vi "数据采集传输系统.vi"(8 "停止 2":bool) -> ()   [LabVIEW 2016]
uses:
  <vilib>/Averna/Notify Icon/NotifyIcon.llb/BalloonIcon.ctl
  <vilib>/Utility/miscctls.llb/LVPointTypeDef.ctl
  <vilib>/Utility/config.llb/Read Key (String).vi
  <vilib>/Utility/config.llb/Read Key (I32).vi
  <vilib>/Utility/config.llb/Read Key (Boolean).vi
  <vilib>/Utility/config.llb/Write Key (String).vi
  <vilib>/Utility/config.llb/Write Key (U32).vi
  <vilib>/Utility/config.llb/Write Key (I32).vi
  <vilib>/Utility/config.llb/Write Key (Boolean).vi
  <vilib>/Averna/Notify Icon/NotifyIcon.llb/GetSelectedItemEvent.vi
  <vilib>/Averna/Notify Icon/NotifyIcon.llb/SetVisible.vi
  <vilib>/Averna/Notify Icon/NotifyIcon.llb/SetMenuDefaultItem.vi
  <vilib>/Averna/Notify Icon/NotifyIcon.llb/SetTipText.vi
  <vilib>/Averna/Notify Icon/NotifyIcon.llb/NotifyIcon.lvclass
  <vilib>/Utility/config.llb/NI_LVConfig.lvlib
  data/FreeMem.dll
  <vilib>/ptbypt/NI_PtbyPt.lvlib
panel:
  in  "日志、参数发送":bool
  in  "2011发送":bool
  in  "判断数据反馈":bool
  in  "数据发送协议":enum16{"2005-212协议", "2017-212协议"}(ring)=enum."2017-212协议"
  in  "数据发送通道":enum16{"TCP", "VISA"}(ring)
  in  "baud rate":u32=9600 caption="波特率"
  in  "VISA resource name":refnum<visa-resource-name> caption="VISA资源名称"
  in  "查询质控数据起始时间":bool
  in  "返回主界面":bool
  out "零点核查索引起始时间":string
  out "跨度核查索引起始时间":string
  out "加标回收索引起始时间":string
  out "标样核查索引起始时间":string
  out "数据接收超时指示灯":bool
  in  "重发时间":T1(ring)
  in  "重发日期":T2(ring)
  in  "锁":bool
  in  "开机启动":bool
  in  "确定更改起始时间":bool
  in  "更改起始时间":bool
  in  "数据发送起始时间":timestamp format="%<%.3X\n%Y/%m/%d>T"
  in  "每周自动重发":bool=TRUE
  in  "确定":bool
  in  "返回":bool
  in  "PW":string
  in  "MN":string
  in  "PORT":string
  in  "IP":string
  in  "站点设备":string
  in  "站点名称":string
  out "设置超时时间/min":i32=1
  in  "实时数据发送时间间隔/min":u32=1
  out "空闲时间/s":string
  out "状态信息":T3={"1st Error to Convert "=63, "步骤 "=enum."打开连接", "元素"="实时数据", "TCP服务端掉线计数"=4, "TCP掉线时间节点"="2019/05/08 15:24:17"} {"1st Error to Convert" items=["无错误", "参数错误", "内存已满", "超出区域", "文件结束", "文件已打开", "一般文件IO错误", "未找到文件", "文件权限错误", "磁盘已满", "路径副本", "打开过多文件", "未启用", "未找到资源文件", "无法添加资源", "未找到资源", "未找到图像", "图像内存错误", "画笔不存在", "配置错误类型", "配置未找到解析段", "配置解析错误", "配置内存错误", "错误外部代码格式", "错误外部代码偏移量", "外部代码不存在", "空窗口", "销毁窗口错误", "空菜单", "打印已中止", "错误打印记录", "打印驱动程序错误", "打印时窗口错误", "打印时内存错误", "打印对话框错误", "一般打印错误", "无效设备引用句柄", "设备未找到", "设备参数错误", "设备单位错误", "无法打开设备", "设备调用已中止", "一般错误", "用户已取消", "对象ID过低", "对象ID过高", "对象不在堆中", "未知的堆", "错误DefProc ID", "DefProc不在表格中", "范围外信息", "空方法", "未知信息", "不支持管理器调用", "错误地址", "连接过程中", "连接超时", "连接过程中", "不支持网络属性", "网络错误", "正在使用的地址", "系统缺少内存", "连接已中止", "连接已拒绝", "连接未建立", "连接已建立", "连接已关闭", "初始化错误（交互应用程序管理器）", "错误事件发生", "等待无约束事件发生处理程序", "事件发生队列溢出", "错误路径", "未发出信号量", "未识别类型（交互应用程序管理器）"]}
  out "系统时间":string
  out "实时小时数据上传":bool
  out "系统状态改变":bool
  out "软件版本":string
  out "掉线指示":bool
  out "核查数据上传":bool
  out "通信状态":bool
  out "重发数据":bool
  out "配置信息":T4
  in  "参数配置":bool
  out "查询数据发送":bool
  out "读取报文显示":string
  out "发送报文显示":string
  out "心跳包":bool
  in  "参数数值":T5={"CODMn"=TRUE, "CODCr"=TRUE, "DO"=TRUE, "铜"=TRUE, "PH"=TRUE, "氨氮"=TRUE, "比电导率"=TRUE, "水温"=TRUE, "盐度(海水)"=TRUE, "浊度"=TRUE, "总氮"=TRUE, "总磷"=TRUE, "叶绿素a"=TRUE, "藻密度"=TRUE, "水位"=TRUE, "流速"=TRUE, "瞬时流量"=TRUE, "累积流量"=TRUE}
  in  "系统编码选择框":string(combo)="地表水质量监测"
  out "主队列输出":refnum<queue>
  in  "TCP掉线时间节点":string
  out "TCP服务端掉线计数":i32
  out "元素":string
  out "步骤":T6(ring)
  out "1st Error to Convert":i32(ring)=56 items=["无错误", "参数错误", "内存已满", "超出区域", "文件结束", "文件已打开", "一般文件IO错误", "未找到文件", "文件权限错误", "磁盘已满", "路径副本", "打开过多文件", "未启用", "未找到资源文件", "无法添加资源", "未找到资源", "未找到图像", "图像内存错误", "画笔不存在", "配置错误类型", "配置未找到解析段", "配置解析错误", "配置内存错误", "错误外部代码格式", "错误外部代码偏移量", "外部代码不存在", "空窗口", "销毁窗口错误", "空菜单", "打印已中止", "错误打印记录", "打印驱动程序错误", "打印时窗口错误", "打印时内存错误", "打印对话框错误", "一般打印错误", "无效设备引用句柄", "设备未找到", "设备参数错误", "设备单位错误", "无法打开设备", "设备调用已中止", "一般错误", "用户已取消", "对象ID过低", "对象ID过高", "对象不在堆中", "未知的堆", "错误DefProc ID", "DefProc不在表格中", "范围外信息", "空方法", "未知信息", "不支持管理器调用", "错误地址", "连接过程中", "连接超时", "连接过程中", "不支持网络属性", "网络错误", "正在使用的地址", "系统缺少内存", "连接已中止", "连接已拒绝", "连接未建立", "连接已建立", "连接已关闭", "初始化错误（交互应用程序管理器）", "错误事件发生", "等待无约束事件发生处理程序", "事件发生队列溢出", "错误路径", "未发出信号量", "未识别类型（交互应用程序管理器）"]
  out "QN":string
  out "时间QN":string
  out "系统编码ST":string
  out "命令编码CN":string
  out "密码PW":string
  out "设备编码MN":string
  out "拆分包及应答Flag":string
  out "数据":string
  in  "实时数据参数选择框":T7={"水样测量数据"=FALSE, "零点核查数据"=TRUE, "跨度核查数据"=TRUE, "加标回收数据"=TRUE, "平行样数据"=FALSE, "标样核查"=TRUE, "集成干预测试"=TRUE}
  out "数据输出":string
  in  "table元素":string
  out "数组":string[](array[string])
  out "数组 2":string[](array[string])
  out "空闲时间":dbl
  out "错误输出":errorcluster
  out "error out":errorcluster
  # "数 据 采 集 传 输 系 统"
  # "读取的参数区"
  # "水样测量数据"
  # "空白测试数据"
  # "跨度核查数据"
  # "加标回收数据"
  # "平行样数据"
  # "标样核查"
  # "集成干预测试"
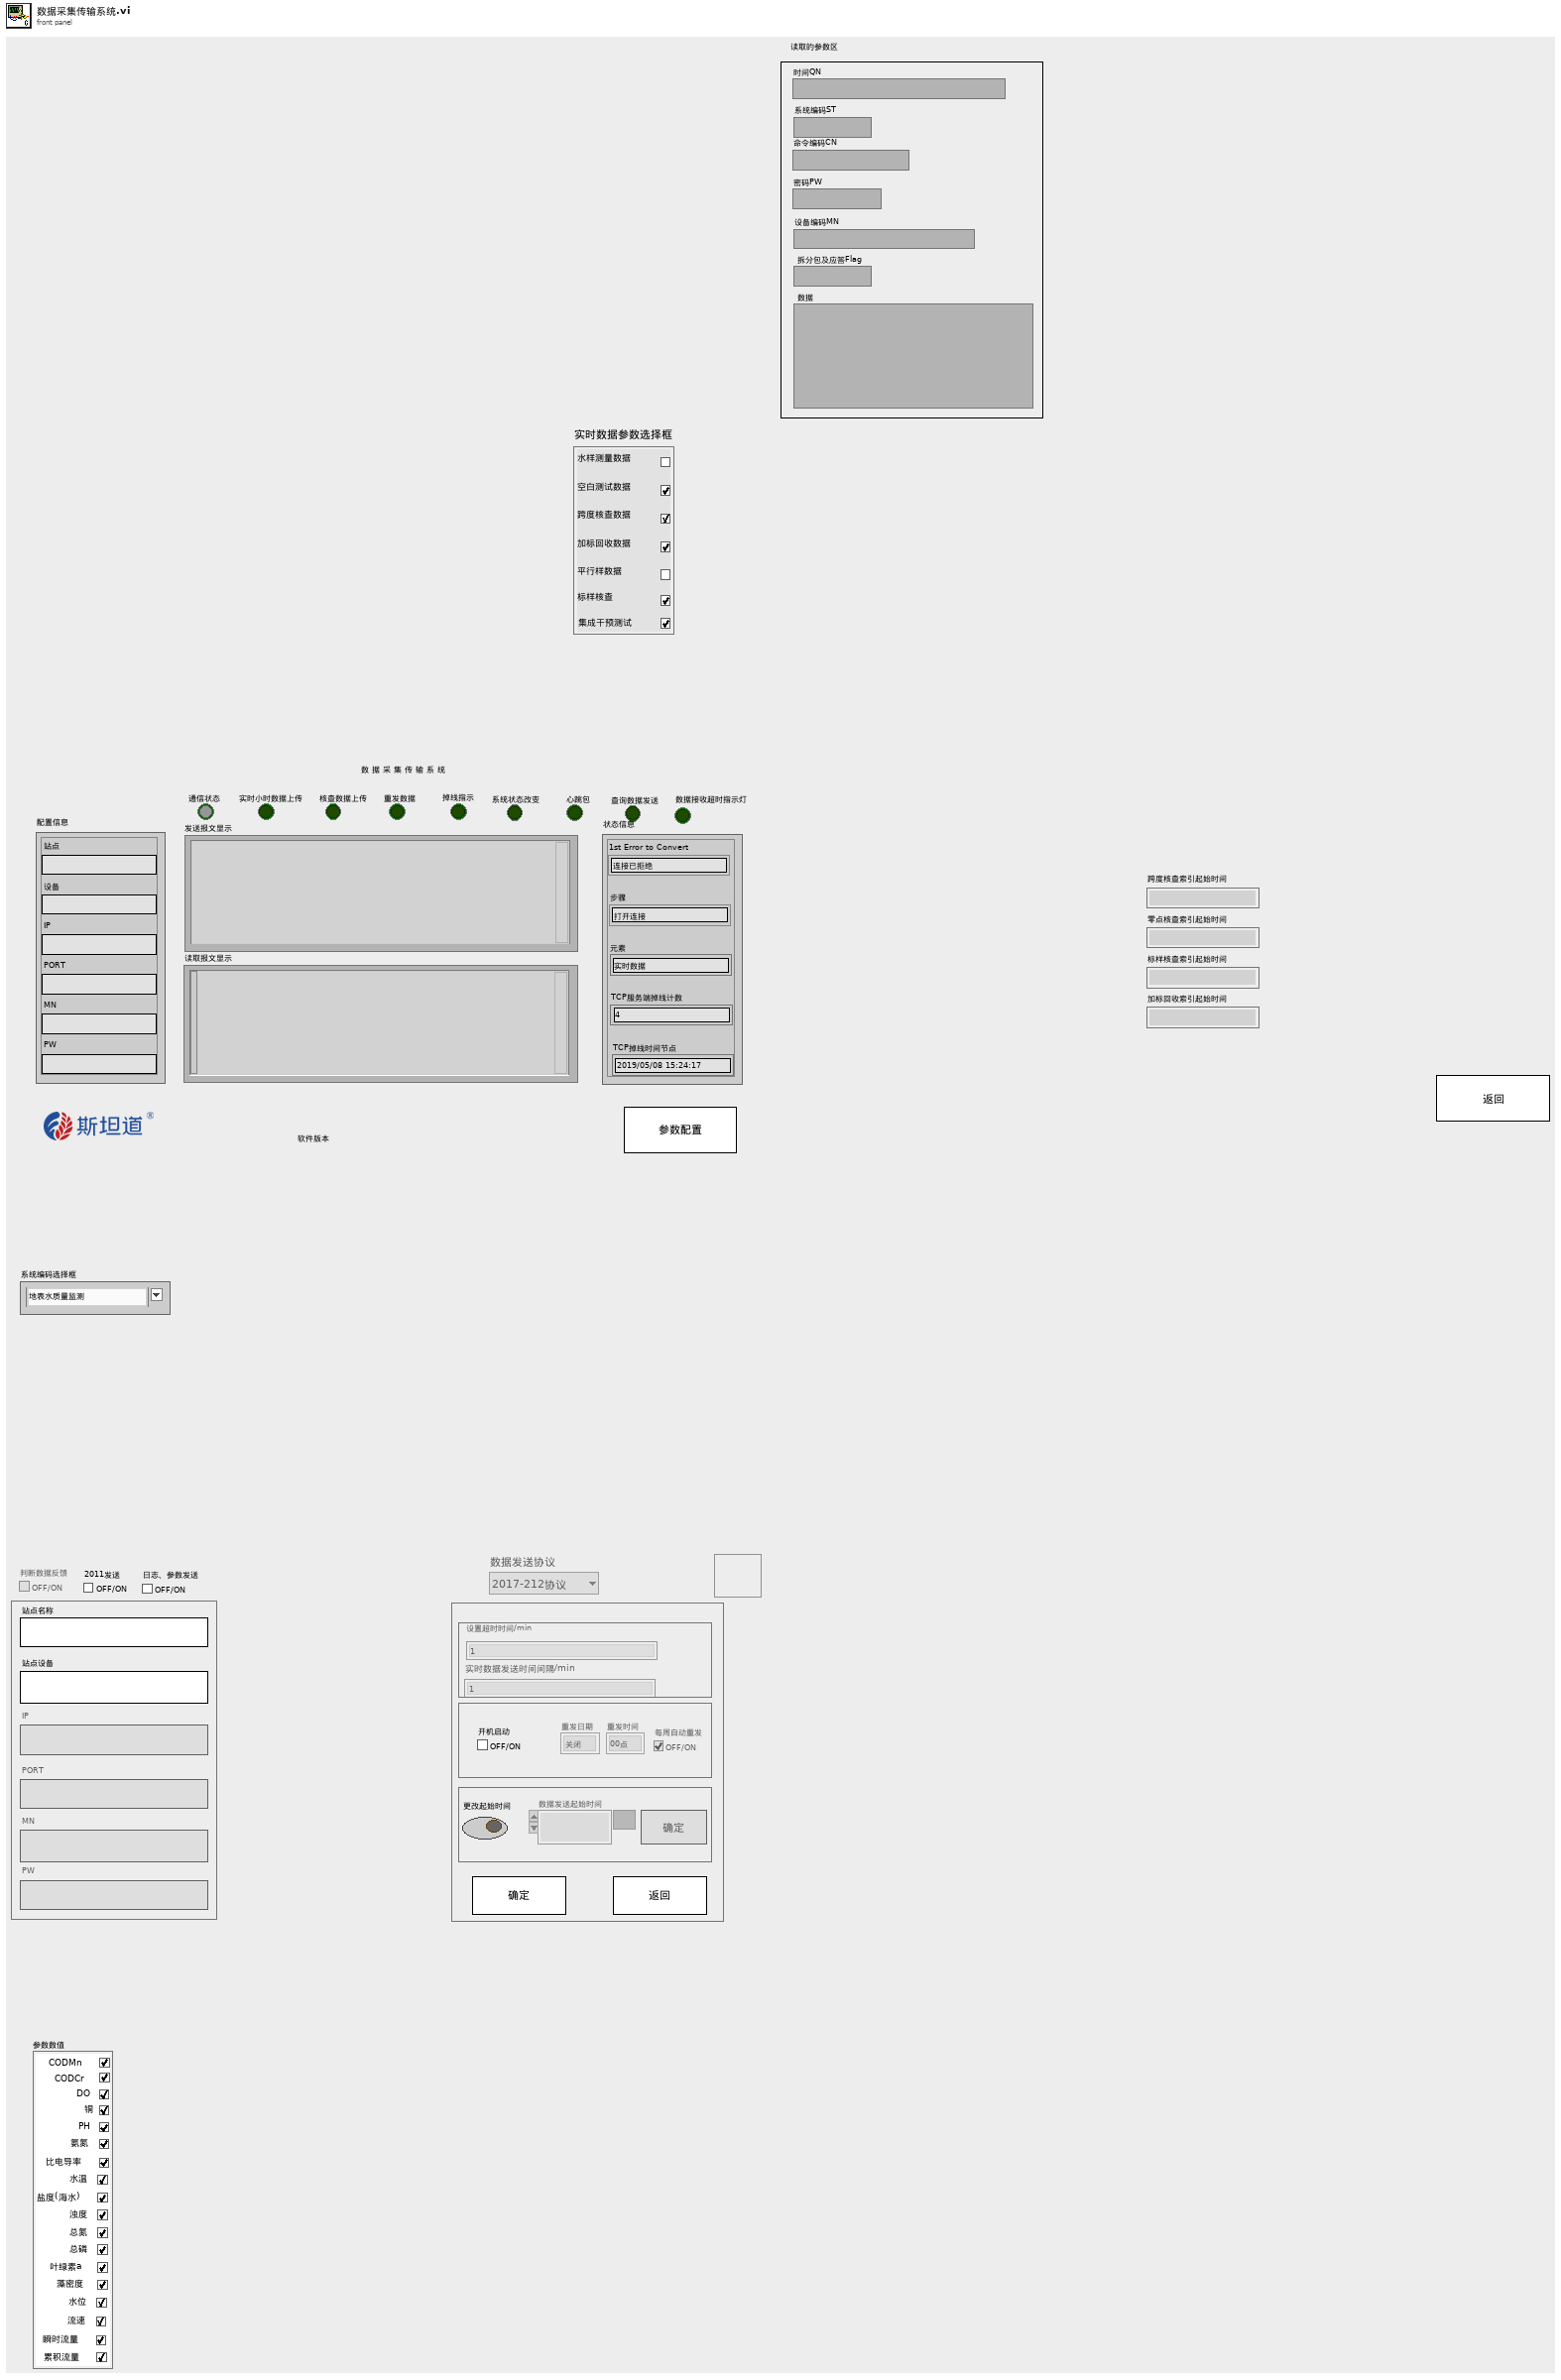
[diagram p1: front panel]
types:
  T1 = enum16{"00点", "01点", "02点", "03点", "04点", "05点", "06点", "07点", "08点", "09点", "10点", "11点", "12点", "13点", "14点", "15点", "16点", "17点", "18点", "19点", "20点", "21点", "22点", "23点"}
  T2 = enum16{"关闭", "星期日", "星期一", "星期二", "星期三", "星期四", "星期五", "星期六"}
  T3 = cluster{"1st Error to Convert ":i32, "步骤 ":enum16{"初始化", "打开连接", "表格比对", "发送数据", "读取数据", "数据处理"}, "元素":string, "TCP服务端掉线计数":i32, "TCP掉线时间节点":string}
  T4 = cluster{"站点":string, "设备":string, "IP":string, "PORT":string, "MN":string, "PW":string}
  T5 = cluster{"CODMn":bool, "CODCr":bool, "DO":bool, "铜":bool, "PH":bool, "氨氮":bool, "比电导率":bool, "水温":bool, "盐度(海水)":bool, "浊度":bool, "总氮":bool, "总磷":bool, "叶绿素a":bool, "藻密度":bool, "水位":bool, "流速":bool, "瞬时流量":bool, "累积流量":bool}
  T6 = enum16{"初始化", "打开连接", "表格比对", "发送数据", "读取数据", "数据处理"}
  T7 = cluster{"水样测量数据":bool, "零点核查数据":bool, "跨度核查数据":bool, "加标回收数据":bool, "平行样数据":bool, "标样核查":bool, "集成干预测试":bool}
  T8 = typedef "NI_LVConfig.lvlib/Config Data RefNum.ctl" = refnum<k1>
  T9 = typedef "LVDateTimeRec.ctl" = cluster{"秒数的小数部分":dbl, "秒":i32, "分":i32, "时":i32, "日":i32, "月":i32, "年":i32, "天数（周）":i32, "天数（年）":i32, "DST":i32}
  T10 = cluster{"PH":string[][], "CODCr":string[][], "氨氮":string[][], "CODMn":string[][], "总氮":string[][], "总磷":string[][], "电导率":string[][], "水温":string[][], "DO":string[][], "浊度":string[][], "叶绿素":string[][], "藻密度":string[][], "铜":string[][], "盐度":string[][], "水位":string[][], "流速":string[][], "瞬时流量":string[][], "累积流量":string[][]}
  T11 = typedef "LVPointTypeDef.ctl" = cluster{"Horizontal":i16, "Vertical":i16}
  T12 = enum8{"Enabled", "Disabled", "Disabled and Grayed Out"}
  T13 = typedef "imagedata.ctl" = cluster{"image type":i32, "image depth":i32, "image":u8[], "mask":u8[], "colors":u32[], "Rectangle":cluster{"left":i16, "top":i16, "right":i16, "bottom":i16}}
  T14 = enum32{"invalid app kind", "Development System", "Run Time System", "Student Edition", "Embedded LabVIEW", "Evaluation", "Custom"}
  T15 = enum32{"Invalid", "Standard", "Closed", "Hidden", "Minimized", "Maximized"}
  T16 = enum16{"水样测试", "小时数据", "日志信息", "报警信息", "零点核查", "标样核查", "平行样", "加标回收"}
  T17 = enum16{"CODMn", "CODCr", "氨氮", "总磷", "总氮", "数采仪"}
  T18 = cluster{"高锰酸盐":string, "化学需氧量":string, "氨氮":string, "总磷":string, "总氮":string, "数采仪":string, "高锰酸盐":bool, "化学需氧量":bool, "氨氮":bool, "总磷":bool, "总氮":bool, "数采仪":bool}
  T19 = typedef "NotifyIcon.lvlib/NotifyIcon.lvclass/BalloonIcon.ctl" = enum32{"None", "Information", "Warning", "Error"}
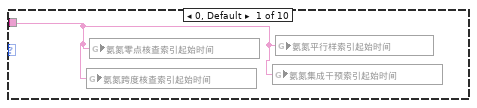
[diagram p5: hidden frame]
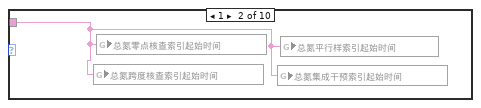
[diagram p6: hidden frame]
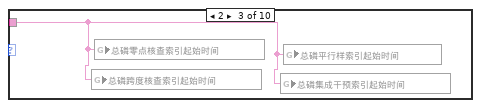
[diagram p7: hidden frame]
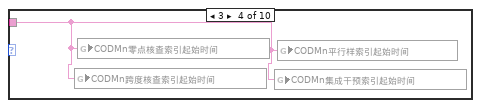
[diagram p8: hidden frame]
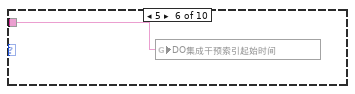
[diagram p9: hidden frame]
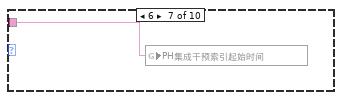
[diagram p10: hidden frame]
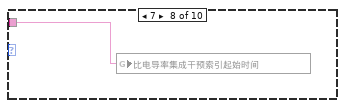
[diagram p11: hidden frame]
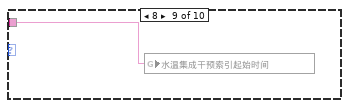
[diagram p12: hidden frame]
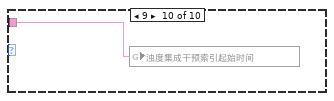
[diagram p13: hidden frame]
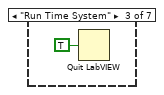
[diagram p16: hidden frame]
diagram:
  w23 = string[] ["OPEN线程一", "APP_SEPARATOR", "EXIT线程一"]
  (unwired) string[] ["CODMn", "CODCr", "DO", "DOper", "PH", "氨氮", "电导率", "水温", "盐度", "浊度", "总氮", "总磷", "叶绿素a", "藻密度", "水位", "流速", "瞬时流量", "累积流量"] ("查询参数数组")
  (unwired) 0 items=["无错误", "参数错误", "内存已满", "超出区域", "文件结束", "文件已打开", "一般文件IO错误", "未找到文件", "文件权限错误", "磁盘已满", "路径副本", "打开过多文件", "未启用", "未找到资源文件", "无法添加资源", "未找到资源", "未找到图像", "图像内存错误", "画笔不存在", "配置错误类型", "配置未找到解析段", "配置解析错误", "配置内存错误", "错误外部代码格式", "错误外部代码偏移量", "外部代码不存在", "空窗口", "销毁窗口错误", "空菜单", "打印已中止", "错误打印记录", "打印驱动程序错误", "打印时窗口错误", "打印时内存错误", "打印对话框错误", "一般打印错误", "无效设备引用句柄", "设备未找到", "设备参数错误", "设备单位错误", "无法打开设备", "设备调用已中止", "一般错误", "用户已取消", "对象ID过低", "对象ID过高", "对象不在堆中", "未知的堆", "错误DefProc ID", "DefProc不在表格中", "范围外信息", "空方法", "未知信息", "不支持管理器调用", "错误地址", "连接过程中", "连接超时", "连接过程中", "不支持网络属性", "网络错误", "正在使用的地址", "系统缺少内存", "连接已中止", "连接已拒绝", "连接未建立", "连接已建立", "连接已关闭", "初始化错误（交互应用程序管理器）", "错误事件发生", "等待无约束事件发生处理程序", "事件发生队列溢出", "错误路径", "未发出信号量", "未识别类型（交互应用程序管理器）"] ("1st Error to Convert")
  # "6."
  # "3."
  # "1."
  # "判定当数据没有传送完毕并掉线，将数据存储入临时表格"
  # "上传本地时间点的实时数据"
  # "目前时间太短，如果掉线了，数据存不了临时表格"
  # "获取需要发送的数据表"
  n1 = Cluster To Array(cluster="参数数值") -> (array=w33:bool[])
  n2 = for {
    tunnel: w33 -> [_] mode=indexing
    tunnel: [w73] -> w32
    i -> [w73]
    w62 = "线程一数据重发功能" ("section")
    # "初始化水样搜索起始时间"
    n3 = case shown="3" w73 {
      tunnel: [w104 w106 w108 w110 w112 w114 w116 w118 w120 w122 w124 w126 w128 w130 w132 w134 w136 w138] -> w77
      frame 0, Default {
        n4 = control-ref of="CODMn"() -> (w105:refnum<vi>)
        n5 = property class="Bool (严格)"(reference=w105) -> ("Label.Text"=w104:string)  [unwired: 1 in, 2 out]
      }
      frame 1 {
        n6 = control-ref of="CODCr"() -> (w107:refnum<vi>)
        n7 = property class="Bool (严格)"(reference=w107) -> ("Label.Text"=w106:string)  [unwired: 1 in, 2 out]
      }
      frame 2 {
        n8 = control-ref of="DO"() -> (w109:refnum<vi>)
        n9 = property class="Bool (严格)"(reference=w109) -> ("Label.Text"=w108:string)  [unwired: 1 in, 2 out]
      }
      frame 3 {
        n10 = control-ref of="铜"() -> (w111:refnum<vi>)
        n11 = property class="Bool (严格)"(reference=w111) -> ("Label.Text"=w110:string)  [unwired: 1 in, 2 out]
      }
      frame 4 {
        n12 = control-ref of="PH"() -> (w113:refnum<vi>)
        n13 = property class="Bool (严格)"(reference=w113) -> ("Label.Text"=w112:string)  [unwired: 1 in, 2 out]
      }
      frame 5 {
        n14 = control-ref of="氨氮"() -> (w115:refnum<vi>)
        n15 = property class="Bool (严格)"(reference=w115) -> ("Label.Text"=w114:string)  [unwired: 1 in, 2 out]
      }
      frame 6 {
        n16 = control-ref of="比电导率"() -> (w117:refnum<vi>)
        n17 = property class="Bool (严格)"(reference=w117) -> ("Label.Text"=w116:string)  [unwired: 1 in, 2 out]
      }
      frame 7 {
        n18 = control-ref of="水温"() -> (w119:refnum<vi>)
        n19 = property class="Bool (严格)"(reference=w119) -> ("Label.Text"=w118:string)  [unwired: 1 in, 2 out]
      }
      frame 8 {
        n20 = control-ref of="盐度(海水)"() -> (w121:refnum<vi>)
        n21 = property class="Bool (严格)"(reference=w121) -> ("Label.Text"=w120:string)  [unwired: 1 in, 2 out]
      }
      frame 9 {
        n22 = control-ref of="浊度"() -> (w123:refnum<vi>)
        n23 = property class="Bool (严格)"(reference=w123) -> ("Label.Text"=w122:string)  [unwired: 1 in, 2 out]
      }
      frame 10 {
        n24 = control-ref of="总氮"() -> (w125:refnum<vi>)
        n25 = property class="Bool (严格)"(reference=w125) -> ("Label.Text"=w124:string)  [unwired: 1 in, 2 out]
      }
      frame 11 {
        n26 = control-ref of="总磷"() -> (w127:refnum<vi>)
        n27 = property class="Bool (严格)"(reference=w127) -> ("Label.Text"=w126:string)  [unwired: 1 in, 2 out]
      }
      frame 12 {
        n28 = control-ref of="叶绿素a"() -> (w129:refnum<vi>)
        n29 = property class="Bool (严格)"(reference=w129) -> ("Label.Text"=w128:string)  [unwired: 1 in, 2 out]
      }
      frame 13 {
        n30 = control-ref of="藻密度"() -> (w131:refnum<vi>)
        n31 = property class="Bool (严格)"(reference=w131) -> ("Label.Text"=w130:string)  [unwired: 1 in, 2 out]
      }
      frame 14 {
        n32 = control-ref of="水位"() -> (w133:refnum<vi>)
        n33 = property class="Bool (严格)"(reference=w133) -> ("Label.Text"=w132:string)  [unwired: 1 in, 2 out]
      }
      frame 15 {
        n34 = control-ref of="流速"() -> (w135:refnum<vi>)
        n35 = property class="Bool (严格)"(reference=w135) -> ("Label.Text"=w134:string)  [unwired: 1 in, 2 out]
      }
      frame 16 {
        n36 = control-ref of="瞬时流量"() -> (w137:refnum<vi>)
        n37 = property class="Bool (严格)"(reference=w137) -> ("Label.Text"=w136:string)  [unwired: 1 in, 2 out]
      }
      frame 17 {
        n38 = control-ref of="累积流量"() -> (w139:refnum<vi>)
        n39 = property class="Bool (严格)"(reference=w139) -> ("Label.Text"=w138:string)  [unwired: 1 in, 2 out]
      }
    }
    n40 = call <vilib>:"Application Directory.vi"() -> ("Application Directory"=w83:path)
    n41 = Build Path(base path=w83, name or relative path="data\\Set.ini" ("名称或相对路径")) -> (appended path=w81:path)
    n42 = call <vilib>:"Open Config Data.vi"("configuration file path"=w81) -> ("error out"=w79:errorcluster, "refnum"=w80:T8)  [unwired: 8 in, 1 out]
    n43 = call-poly <vilib>:"Read Key.vi"("section"="线程一数据搜索起始时间", "error in (no error)"=w79, "key"=w77, "refnum"=w80) -> ("error out"=w71:errorcluster, "value"=w74:string, "refnum out"=w72:T8)  [unwired: 4 in, 1 out]
    n44 = Empty String/Path?(string/path=w74) -> (empty?=w76:bool)
    n45 = case shown="真" w76 {
      tunnel: [w84 "1904/01/01 00:00:00"] -> w75
      tunnel: w74 -> [w84 _]
      frame False {
      }
      frame True {
      }
    }
    n46 = call-poly <vilib>:"Read Key.vi"("section"=w62, "error in (no error)"=w71, "key"="重发功能", "refnum"=w72) -> ("error out"=w65:errorcluster, "value"=w69:bool, "refnum out"=w66:T8)  [unwired: 4 in, 1 out]
    n47 = local write "每周自动重发"(w69) -> ()
    n48 = call-poly <vilib>:"Read Key.vi"("section"=w62, "error in (no error)"=w65, "key"="重发日期", "refnum"=w66) -> ("error out"=w63:errorcluster, "value"=w59:i32, "refnum out"=w64:T8)  [unwired: 4 in, 1 out]
    n49 = local write "重发日期"(w59) -> ()
    n50 = case shown="3" w73 {
      tunnel: w75 -> [w86 w87 w88 w89 w90 w91 w92 w93 w94 w95 w96 w97 w98 w99 w100 w101 w102 w103]
      frame 0, Default {
        n51 = global write "全局 水样时间.vi" "time1"(w86) -> ()
      }
      frame 1 {
        n52 = global write "全局 水样时间.vi" "time2"(w87) -> ()
      }
      frame 2 {
        n53 = global write "全局 水样时间.vi" "time3"(w88) -> ()
      }
      frame 3 {
        n54 = global write "全局 水样时间.vi" "time4"(w89) -> ()
      }
      frame 4 {
        n55 = global write "全局 水样时间.vi" "time5"(w90) -> ()
      }
      frame 5 {
        n56 = global write "全局 水样时间.vi" "time6"(w91) -> ()
      }
      frame 6 {
        n57 = global write "全局 水样时间.vi" "time7"(w92) -> ()
      }
      frame 7 {
        n58 = global write "全局 水样时间.vi" "time8"(w93) -> ()
      }
      frame 8 {
        n59 = global write "全局 水样时间.vi" "time9"(w94) -> ()
      }
      frame 9 {
        n60 = global write "全局 水样时间.vi" "time10"(w95) -> ()
      }
      frame 10 {
        n61 = global write "全局 水样时间.vi" "time11"(w96) -> ()
      }
      frame 11 {
        n62 = global write "全局 水样时间.vi" "time12"(w97) -> ()
      }
      frame 12 {
        n63 = global write "全局 水样时间.vi" "time13"(w98) -> ()
      }
      frame 13 {
        n64 = global write "全局 水样时间.vi" "time14"(w99) -> ()
      }
      frame 14 {
        n65 = global write "全局 水样时间.vi" "time15"(w100) -> ()
      }
      frame 15 {
        n66 = global write "全局 水样时间.vi" "time16"(w101) -> ()
      }
      frame 16 {
        n67 = global write "全局 水样时间.vi" "time17"(w102) -> ()
      }
      frame 17 {
        n68 = global write "全局 水样时间.vi" "time18"(w103) -> ()
      }
    }
    n69 = call-poly <vilib>:"Read Key.vi"("section"=w62, "error in (no error)"=w63, "key"="重发时间", "refnum"=w64) -> ("error out"=w60:errorcluster, "value"=w58:i32, "refnum out"=w61:T8)  [unwired: 4 in, 1 out]
    n70 = local write "重发时间"(w58) -> ()
    n71 = call <vilib>:"Close Config Data.vi"("error in (no error)"=w60, "refnum"=w61) -> ()  [unwired: 8 in, 2 out]
  }
  n72 = Obtain Queue(name (unnamed)="数据发送" ("名称（未命名）"), element data type="") -> (queue out=w38:refnum<queue>, error out=w37:errorcluster)  [unwired: 3 in, 1 out]
  n73 = Obtain Queue(name (unnamed)="实时数据参数选择" ("名称（未命名）"), element data type="") -> (queue out=w39:refnum<queue>, error out=w36:errorcluster)  [unwired: 3 in, 1 out]
  n74 = while {
    tunnel: w38 -> [w155]
    stop <- FALSE stop-if-true
    # "核查和质控数据的定期发送在实时数据周期上传"
    # "指定周期发一次核查数据，仪器参数日志"
    n75 = local read "核查数据上传"() -> (w141:bool)
    n76 = local read "查询数据发送"() -> (w150:bool)
    n77 = local read "实时小时数据上传"() -> (w154:bool)
    n78 = local read "重发数据"() -> (w151:bool)
    n79 = Multiply(x="实时数据发送时间间隔/min", y=u32 60000 ("等待时间（毫秒）")) -> (x*y=w158:u32)
    n80 = local read "步骤"() -> (w149:T6)
    n81 = Not(x=w141) -> (.not. x?=w140:bool)
    n82 = Not(x=w150) -> (.not. x?=w146:bool)
    n83 = Wait (ms)(milliseconds to wait=w158) -> ()  [unwired: 1 out]
    n84 = Not(x=w151) -> (.not. x?=w145:bool)
    n85 = Not(x=w154) -> (.not. x?=w152:bool)
    n86 = First Call?() -> (First Call?: T/F=w156:bool)
    n87 = Equal?(x=w149, y=T6."读取数据" ("步骤")) -> (x = y?=w147:bool)
    n88 = case shown="真" w156 {
      tunnel: w155 -> [_ _]
      frame False {
      }
      frame True {
        (unwired) "1994/01/01 00:00:00"
        # "上传最近一年的质控数据"
        n89 = Get Date/Time In Seconds() -> (seconds since 1Jan1904=w193:timestamp)
        n90 = Seconds To Date/Time(time stamp (now)=w193) -> (date time rec=w191:T9)  [unwired: 1 in]
        n91 = Unbundle By Name(w191) -> ("年"=w192:i32)
        n92 = Decrement(x=w192) -> (x-1=w190:i32)
        n93 = Bundle By Name(cluster=w191, "年"=w190) -> (w188:T9)
        n94 = Date/Time To Seconds(2:w188) -> (0:w189:timestamp)  [unwired: 1 in]
        n95 = Format Date/Time String(time format string (%c)="%Y/%m/%d %H:%M:%S" ("时间格式字符串(%c)"), seconds (now)=w189) -> (date/time string=w186:string)  [unwired: 1 in]
        n96 = global write "全局 时间2.vi" "跨度核查索引起始时间"(w186) -> ()
        n97 = global write "全局 时间2.vi" "零点核查索引起始时间"(w186) -> ()
        n98 = global write "全局 时间2.vi" "平行样索引起始时间"(w186) -> ()
        n99 = global write "全局 时间2.vi" "加标回收索引起始时间"(w186) -> ()
        n100 = global write "全局 时间2.vi" "标样核查索引起始时间"(w186) -> ()
        n101 = call <vilib>:"Application Directory.vi"() -> ("Application Directory"=w183:path)
        n102 = Build Path(base path=w183, name or relative path="data\\hecha.ini" ("名称或相对路径")) -> (appended path=w185:path)
        n103 = call <vilib>:"Open Config Data.vi"("configuration file path"=w185) -> ("error out"=w179:errorcluster, "refnum"=w180:T8)  [unwired: 8 in, 1 out]
        n104 = vi-ref "全局 时间2.vi"() -> (w181:refnum<vi>)
        n105 = call <userlib>:"Read Panel from INI__ogtk.vi"("error in (no error)"=w179, "VI ref"=w181, "refnum"=w180) -> ("error out"=w178:errorcluster, "refnum out"=w182:T8)  [unwired: 7 in]
        n106 = call <vilib>:"Close Config Data.vi"("error in (no error)"=w178, "refnum"=w182) -> ("error out"=w177:errorcluster)  [unwired: 8 in, 1 out]
        n107 = disable-structure shown="禁用" {
          disable-tunnel: w186 -> [w196 _]
          disable-tunnel: w177 -> [w194 _]
          frame Disabled {
            n108 = for {
              N: 10 -> [_]
              tunnel: w196 -> [w197]
              tunnel: w194 -> [_]
              i -> [w198]
              n109 = case shown="4" w198 {
                tunnel: w197 -> [w199 w200 w201 w202 w203 w204 w205 w206 w207 w208]
                frame 0, Default {
                  n110 = global write "全局 时间2.vi" "氨氮跨度核查索引起始时间"(w199) -> ()
                  n111 = global write "全局 时间2.vi" "氨氮零点核查索引起始时间"(w199) -> ()
                  n112 = global write "全局 时间2.vi" "氨氮集成干预索引起始时间"(w199) -> ()
                  n113 = global write "全局 时间2.vi" "氨氮平行样索引起始时间"(w199) -> ()
                }
                frame 1 {
                  n114 = global write "全局 时间2.vi" "总氮跨度核查索引起始时间"(w200) -> ()
                  n115 = global write "全局 时间2.vi" "总氮零点核查索引起始时间"(w200) -> ()
                  n116 = global write "全局 时间2.vi" "总氮集成干预索引起始时间"(w200) -> ()
                  n117 = global write "全局 时间2.vi" "总氮平行样索引起始时间"(w200) -> ()
                }
                frame 2 {
                  n118 = global write "全局 时间2.vi" "总磷跨度核查索引起始时间"(w201) -> ()
                  n119 = global write "全局 时间2.vi" "总磷零点核查索引起始时间"(w201) -> ()
                  n120 = global write "全局 时间2.vi" "总磷集成干预索引起始时间"(w201) -> ()
                  n121 = global write "全局 时间2.vi" "总磷平行样索引起始时间"(w201) -> ()
                }
                frame 3 {
                  n122 = global write "全局 时间2.vi" "CODMn跨度核查索引起始时间"(w202) -> ()
                  n123 = global write "全局 时间2.vi" "CODMn零点核查索引起始时间"(w202) -> ()
                  n124 = global write "全局 时间2.vi" "CODMn集成干预索引起始时间"(w202) -> ()
                  n125 = global write "全局 时间2.vi" "CODMn平行样索引起始时间"(w202) -> ()
                }
                frame 4 {
                  n126 = global write "全局 时间2.vi" "CODCr跨度核查索引起始时间"(w203) -> ()
                  n127 = global write "全局 时间2.vi" "CODCr零点核查索引起始时间"(w203) -> ()
                  n128 = global write "全局 时间2.vi" "CODCr集成干预索引起始时间"(w203) -> ()
                  n129 = global write "全局 时间2.vi" "CODCr平行样索引起始时间"(w203) -> ()
                }
                frame 5 {
                  n130 = global write "全局 时间2.vi" "DO集成干预索引起始时间"(w204) -> ()
                }
                frame 6 {
                  n131 = global write "全局 时间2.vi" "PH集成干预索引起始时间"(w205) -> ()
                }
                frame 7 {
                  n132 = global write "全局 时间2.vi" "比电导率集成干预索引起始时间"(w206) -> ()
                }
                frame 8 {
                  n133 = global write "全局 时间2.vi" "水温集成干预索引起始时间"(w207) -> ()
                }
                frame 9 {
                  n134 = global write "全局 时间2.vi" "浊度集成干预索引起始时间"(w208) -> ()
                }
              }
            }
          }
          frame Enabled {
          }
        }
      }
    }
    n135 = local read "数据发送协议"() -> (w144:enum16{"2005-212协议", "2017-212协议"})
    n136 = Equal?(x=w144, y=enum16{"2005-212协议", "2017-212协议"}."2017-212协议" ("数据发送协议")) -> (x = y?=w142:bool)
    n137 = Compound Arithmetic op=AND ("复合运算")(w140, w142, w145, w146, w147, w152) -> (w153:bool)
    n138 = case shown="真" w153 {
      tunnel: w155 -> [_ w165]
      frame False {
      }
      frame True {
        n139 = call "实时数据参数入列队.vi"("实时数据参数选择框"="实时数据参数选择框") -> ("错误输出"=w167:errorcluster)  [unwired: 10 in]
        n140 = local read "日志、参数发送"() -> (w161:bool)
        n141 = call <vilib>:"Clear Errors.vi"("error in (no error)"=w167) -> ()  [unwired: 5 in, 2 out]
        n142 = Enqueue Element(queue=w165, element="send" ("元素")) -> (queue out=w164:refnum<queue>, error out=w163:errorcluster)  [unwired: 2 in, 1 out]
        n143 = case shown="真" w161 {
          tunnel: w164 -> [_ w174]
          tunnel: w163 -> [_ w173]
          frame False {
          }
          frame True {
            n144 = Enqueue Element(queue=w174, element="操作日志" ("元素"), error in (no error)=w173) -> (queue out=w171:refnum<queue>, error out=w170:errorcluster)  [unwired: 1 in, 1 out]
            n145 = Enqueue Element(queue=w171, element="仪器参数" ("元素"), error in (no error)=w170) -> (queue out=w169:refnum<queue>, error out=w168:errorcluster)  [unwired: 1 in, 1 out]
            n146 = Enqueue Element(queue=w169, element="报警信息" ("元素"), error in (no error)=w168) -> ()  [unwired: 1 in, 3 out]
          }
        }
      }
    }
  }
  n147 = while "While循环" {
    tunnel: w38 -> [w221]
    tunnel: w39 -> [w225]
    tunnel: w37 -> [w224]
    tunnel: w36 -> [w223]
    stop <- FALSE stop-if-true
    # "判定数据发送时要发送实时数据"
    # "所有的主动上传数据都是有数据才会上传"
    n148 = Get Queue Status(queue=w221) -> (# elements in queue=w213:i32)  [unwired: 2 in, 7 out]
    n149 = local read "查询数据发送"() -> (w219:bool)
    n150 = global read "全局 数据发送重叠.vi" "主动上报数据中"() -> (w211:bool)
    n151 = local read "重发数据"() -> (w210:bool)
    n152 = Not Equal To 0?(x=w213) -> (x != 0?=w220:bool)
    n153 = And(x=w220, y=w219) -> (x .and. y?=w212:bool)
    n154 = call <vilib>:"Boolean Crossing PtByPt.vi"("direction"=enum16{"either", "false-true", "true-false"}."false-true", "input"=w212) -> ("crossing"=w218:bool)  [unwired: 1 in]
    n155 = Not(x=w211) -> (.not. x?=w215:bool)
    n156 = Not(x=w210) -> (.not. x?=w209:bool)
    n157 = Not(x=w219) -> (.not. x?=w216:bool)
    n158 = case shown="真" w218 {
      frame False {
      }
      frame True {
        n159 = Get Date/Time In Seconds() -> (seconds since 1Jan1904=w231:timestamp)
        n160 = Seconds To Date/Time(time stamp (now)=w231) -> (date time rec=w228:T9)  [unwired: 1 in]
        n161 = Date/Time To Seconds(2:w228) -> (0:w230:timestamp)  [unwired: 1 in]
        n162 = Format Date/Time String(time format string (%c)="%Y/%m/%d %H:%M:%S" ("时间格式字符串(%c)"), seconds (now)=w230) -> (date/time string=w227:string)  [unwired: 1 in]
        n163 = global write "全局 数据发送重叠.vi" "数据发送重叠开始时间戳"(w227) -> ()
      }
    }
    n164 = Compound Arithmetic op=AND ("复合运算")(w216, w215, w209) -> (w214:bool)
    n165 = Wait (ms)(milliseconds to wait=u32 1000 ("等待时间（毫秒）")) -> ()  [unwired: 1 out]
    n166 = case shown="真" w214 {
      tunnel: w221 -> [_ w241]
      tunnel: w225 -> [_ w240]
      tunnel: w224 -> [_ w239]
      tunnel: w223 -> [_ w238]
      tunnel: w213 -> [_ w234]
      tunnel: w212 -> [_ w233]
      frame False {
        n167 = local write "核查数据上传"(FALSE ("数据上传")) -> ()
      }
      frame True {
        n168 = Equal To 0?(x=w234) -> (x = 0?=w235:bool)
        n169 = global write "全局 数据发送重叠.vi" "数据发送重叠"(w233) -> ()
        n170 = Not(x=w235) -> (.not. x?=w236:bool)
        n171 = local write "核查数据上传"(w236) -> ()
        n172 = Dequeue Element(queue=w241, error in (no error)=w239) -> (element=w237:string)  [unwired: 1 in, 3 out]
        n173 = case shown="\"send\"" w237 {
          tunnel: w240 -> [_ w243 _ _ _ _ _ _ _ _ _]
          tunnel: w238 -> [_ w242 _ _ _ _ _ _ _ _ _]
          frame "假", Default {
          }
          frame "send" {
            # "间隔时间上传"
            n174 = while {
              tunnel: w243 -> [w247]
              tunnel: w242 -> [w244]
              stop <- w248 stop-if-true
              n175 = Dequeue Element(queue=w247, error in (no error)=w244) -> (queue out=w246:refnum<queue>, element=w249:string)  [unwired: 1 in, 2 out]
              n176 = case shown="\"空白测试\"" w249 {
                tunnel: [_ _ _ w415 _ _ _ w622] -> w248
                tunnel: w246 -> [_ _ _ _ _ _ _ w625]
                frame "水样测试" {
                  n177 = flat-sequence {
                    frame #0 {
                      n178 = global write "全局 小时数据发送次数.vi" "小时数据发送次数"(0 ("小时数据发送次数")) -> ()
                      n179 = global write "全局 实时数据参数.vi" "实时数据参数"("水样测试") -> ()
                      n180 = global write "全局1.vi" "枚举"(enum16{"返回请求应答", "上传数据", "返回执行结果"}."上传数据" ("枚举")) -> ()
                    }
                    frame #1 {
                      n181 = call "从数据库获取数据通用可配置(子VI).vi"("table输入"="实时数据" ("新元素/子数组"), "列队名（唯一）"="a") -> ()  [unwired: 8 in, 2 out]
                    }
                    frame #2 {
                      n182 = call "实时小时数据处理整合 (子VI).vi"("枚举"=enum16{"实时数据排序", "小时数据排序"}."实时数据排序") -> ("已排序的数组"=w256:string[])  [unwired: 10 in]
                      n183 = Array Size(array=w256) -> (size(s)=w257:i32)
                      n184 = global write "全局 数据数组大小.vi" "数据数组大小"(w257) -> ()
                    }
                    frame #3 {
                      n185 = while {
                        stop <- w262 stop-if-true
                        n186 = property on="TCP服务端掉线计数" class="DigNum (严格)"() -> ("Value"=w265:i32)  [unwired: 2 in, 2 out]
                        n187 = Greater Or Equal?(x=w265, y=1) -> (x >= y?=w264:bool)
                        n188 = case shown="假" w264 {
                          frame False {
                            n189 = global read "全局 数据数组大小.vi" "数据数组大小"() -> (w267:i32)
                            n190 = Greater Than 0?(x=w267) -> (x > 0?=w268:bool)
                            n191 = case shown="真" w268 {
                              frame False {
                              }
                              frame True {
                                n192 = local read "MN"() -> (w274:string)
                                n193 = local read "PW"() -> (w273:string)
                                n194 = local read "数据发送通道"() -> (w272:enum16{"TCP", "VISA"})
                                n195 = call "数据编码.vi"("table输入"="实时数据" ("新元素/子数组"), "MN"=w274, "PW"=w273) -> ("通讯包字符串"=w269:string)  [unwired: 11 in, 1 out]
                                n196 = local write "发送报文显示"(w269) -> ()
                                n197 = call "VISATCP组合选择发送.vi"("数据发送通道"=w272, "命令"="write", "写入缓冲区"=w269) -> ("错误输出"=→"错误输出":errorcluster)  [unwired: 9 in, 3 out]
                                n198 = Build Array(w269) -> (w276:string[])
                                n199 = call "发送数据记录到文档(子VI).vi"("数组"=w276) -> ()  [unwired: 9 in, 1 out]
                                "核查数据上传" <- TRUE ("主动数据上传")
                              }
                            }
                          }
                          frame True {
                          }
                        }
                        n200 = Wait (ms)(milliseconds to wait=u32 500 ("等待时间（毫秒）")) -> ()  [unwired: 1 out]
                        n201 = global read "全局 数据数组大小.vi" "数据数组大小"() -> (w259:i32)
                        n202 = global read "全局 小时数据发送次数.vi" "小时数据发送次数"() -> (w263:i32)
                        n203 = Decrement(x=w259) -> (x-1=w258:i32)
                        n204 = Greater Or Equal?(x=w263, y=w258) -> (x >= y?=w261:bool)
                        n205 = Compound Arithmetic op=OR ("复合运算")(w261) -> (w262:bool)
                      }
                    }
                  }
                }
                frame "空白测试" {
                  n206 = flat-sequence {
                    frame #0 {
                      n207 = global write "全局 小时数据发送次数.vi" "小时数据发送次数"(0 ("小时数据发送次数")) -> ()
                      n208 = global write "全局 实时数据参数.vi" "实时数据参数"("空白测试") -> ()
                      n209 = global write "全局1.vi" "枚举"(enum16{"返回请求应答", "上传数据", "返回执行结果"}."上传数据" ("枚举")) -> ()
                    }
                    frame #1 {
                      n210 = call "从数据库获取数据通用可配置(子VI).vi"("table输入"="实时数据" ("新元素/子数组"), "列队名（唯一）"="b") -> ()  [unwired: 8 in, 2 out]
                    }
                    frame #2 {
                      n211 = for {
                        N: 5 -> [_]
                        i -> [w285]
                        # "行数大于零"
                        n212 = case shown="3" w285 {
                          tunnel: [w289 w290 w291 w292 w293] -> w284
                          frame 0, Default {
                            n213 = global read "全局 所有参数.vi" "氨氮"() -> (w289:string[][])
                          }
                          frame 1 {
                            n214 = global read "全局 所有参数.vi" "总氮"() -> (w290:string[][])
                          }
                          frame 2 {
                            n215 = global read "全局 所有参数.vi" "总磷"() -> (w291:string[][])
                          }
                          frame 3 {
                            n216 = global read "全局 所有参数.vi" "CODMn"() -> (w292:string[][])
                          }
                          frame 4 {
                            n217 = global read "全局 所有参数.vi" "CODCr"() -> (w293:string[][])
                          }
                        }
                        n218 = Array Size(array=w284) -> (size(s)=w287:i32[])
                        n219 = Index Array(array=w287) -> (element=w286:i32)  [unwired: 1 in]
                        n220 = Greater Than 0?(x=w286) -> (x > 0?=w288:bool)
                        n221 = case shown="真" w288 {
                          tunnel: w285 -> [_ w299]
                          tunnel: w286 -> [_ _]
                          tunnel: w284 -> [_ w297]
                          frame False {
                          }
                          frame True {
                            # "最新时间戳加1分钟"
                            n222 = Index Array(array=w297, index (row)=0 ("禁用的索引 (行)"), index (col)=0 ("禁用的索引 (列)")) -> (element=w296:string)
                            n223 = call "日期时间字符串转换分钟数加一.vi"("data[0]"=w296) -> ("日期/时间字符串"=w295:string)  [unwired: 10 in]
                            n224 = case shown="0, 默认" w299 {
                              tunnel: w295 -> [w300 w301 w302 w303 w304]
                              frame 0, Default {
                                n225 = global write "全局 时间2.vi" "氨氮零点核查索引起始时间"(w300) -> ()
                              }
                              frame 1 {
                                n226 = global write "全局 时间2.vi" "总氮零点核查索引起始时间"(w301) -> ()
                              }
                              frame 2 {
                                n227 = global write "全局 时间2.vi" "总磷零点核查索引起始时间"(w302) -> ()
                              }
                              frame 3 {
                                n228 = global write "全局 时间2.vi" "CODMn零点核查索引起始时间"(w303) -> ()
                              }
                              frame 4 {
                                n229 = global write "全局 时间2.vi" "CODCr零点核查索引起始时间"(w304) -> ()
                              }
                            }
                          }
                        }
                      }
                    }
                    frame #3 {
                      n230 = call <vilib>:"Application Directory.vi"() -> ("Application Directory"=w318:path)
                      n231 = Build Path(base path=w318, name or relative path="data\\hecha.ini" ("名称或相对路径")) -> (appended path=w316:path)
                      n232 = call <vilib>:"Open Config Data.vi"("configuration file path"=w316) -> ("error out"=w312:errorcluster, "refnum"=w315:T8)  [unwired: 8 in, 1 out]
                      n233 = call "数据处理整合 (子VI).vi"("枚举"=enum16{"实时数据排序", "小时数据排序"}."实时数据排序") -> ("已排序的数组"=w321:string[])  [unwired: 10 in]
                      n234 = vi-ref "全局 时间2.vi"() -> (w314:refnum<vi>)
                      n235 = Array Size(array=w321) -> (size(s)=w320:i32)
                      n236 = call <userlib>:"Write Panel to INI__ogtk.vi"("error in (no error)"=w312, "VI ref"=w314, "refnum"=w315) -> ("error out"=w311:errorcluster, "refnum out"=w313:T8)  [unwired: 7 in]
                      n237 = call <vilib>:"Close Config Data.vi"("error in (no error)"=w311, "refnum"=w313) -> ("error out"=w306:errorcluster, "file path"=w305:path)  [unwired: 8 in]
                      n238 = global write "全局 数据数组大小.vi" "数据数组大小"(w320) -> ()
                      n239 = Open/Create/Replace File(file path (use dialog)=w305, error in=w306) -> (refnum out=w309:refnum<file>, error out=w310:errorcluster)  [unwired: 4 in, 1 out]
                      n240 = Flush File(refnum=w309, error in=w310) -> (refnum out=w308:refnum<file>, error out=w307:errorcluster)
                      n241 = Close File(refnum=w308, error in=w307) -> ()  [unwired: 2 out]
                    }
                    frame #4 {
                      n242 = while {
                        stop <- w324 stop-if-true
                        n243 = property on="TCP服务端掉线计数" class="DigNum (严格)"() -> ("Value"=w328:i32)  [unwired: 2 in, 2 out]
                        n244 = Greater Or Equal?(x=w328, y=1) -> (x >= y?=w327:bool)
                        n245 = case shown="假" w327 {
                          frame False {
                            n246 = global read "全局 数据数组大小.vi" "数据数组大小"() -> (w331:i32)
                            n247 = Greater Than 0?(x=w331) -> (x > 0?=w330:bool)
                            n248 = case shown="真" w330 {
                              frame False {
                              }
                              frame True {
                                w332 = 0 ("禁用的索引 (列)")
                                n249 = global read "插值后的新数组.vi" "插值后的数组元素"() -> (w342:T10)
                                n250 = local write "核查数据上传"(TRUE ("数据上传")) -> ()
                                n251 = local read "MN"() -> (w338:string)
                                n252 = local read "PW"() -> (w337:string)
                                n253 = local read "数据发送通道"() -> (w336:enum16{"TCP", "VISA"})
                                n254 = call "数据编码.vi"("table输入"="实时数据" ("新元素/子数组"), "MN"=w338, "PW"=w337) -> ("通讯包字符串"=w334:string)  [unwired: 11 in, 1 out]
                                n255 = Unbundle By Name(w342) -> ("氨氮"=w341:string[][])
                                n256 = local write "发送报文显示"(w334) -> ()
                                n257 = Build Array(w334) -> (w344:string[])
                                n258 = call "VISATCP组合选择发送.vi"("数据发送通道"=w336, "命令"="write", "写入缓冲区"=w334) -> ("错误输出"=w333:errorcluster)  [unwired: 9 in, 3 out]
                                n259 = Index Array(array=w341, index (row)=w332, index (col)=w332) -> (element=w340:string)
                                n260 = call "发送数据记录到文档(子VI).vi"("数组"=w344) -> ()  [unwired: 9 in, 1 out]
                                n261 = local write "错误输出"(w333) -> ()
                                n262 = call "日期时间字符串转换分钟数加一.vi"("data[0]"=w340) -> ("日期/时间字符串"=w339:string)  [unwired: 10 in]
                                n263 = global write "全局 时间2.vi" "零点核查索引起始时间"(w339) -> ()
                              }
                            }
                          }
                          frame True {
                          }
                        }
                        n264 = Wait (ms)(milliseconds to wait=u32 500 ("等待时间（毫秒）")) -> ()  [unwired: 1 out]
                        n265 = global read "全局 数据数组大小.vi" "数据数组大小"() -> (w322:i32)
                        n266 = global read "全局 小时数据发送次数.vi" "小时数据发送次数"() -> (w326:i32)
                        n267 = Greater Or Equal?(x=w326, y=w322) -> (x >= y?=w325:bool)
                        n268 = Compound Arithmetic op=OR ("复合运算")(w325) -> (w324:bool)
                      }
                    }
                  }
                }
                frame "跨度核查" {
                  n269 = flat-sequence {
                    frame #0 {
                      n270 = global write "全局 小时数据发送次数.vi" "小时数据发送次数"(0 ("小时数据发送次数")) -> ()
                      n271 = global write "全局 实时数据参数.vi" "实时数据参数"("跨度核查") -> ()
                      n272 = global write "全局1.vi" "枚举"(enum16{"返回请求应答", "上传数据", "返回执行结果"}."上传数据" ("枚举")) -> ()
                    }
                    frame #1 {
                      n273 = call "从数据库获取数据通用可配置(子VI).vi"("table输入"="实时数据" ("新元素/子数组"), "列队名（唯一）"="c") -> ()  [unwired: 8 in, 2 out]
                    }
                    frame #2 {
                      n274 = for {
                        N: 5 -> [_]
                        i -> [w352]
                        # "行数大于零"
                        n275 = case shown="3" w352 {
                          tunnel: [w357 w358 w359 w360 w361] -> w353
                          frame 0, Default {
                            n276 = global read "全局 所有参数.vi" "氨氮"() -> (w357:string[][])
                          }
                          frame 1 {
                            n277 = global read "全局 所有参数.vi" "总氮"() -> (w358:string[][])
                          }
                          frame 2 {
                            n278 = global read "全局 所有参数.vi" "总磷"() -> (w359:string[][])
                          }
                          frame 3 {
                            n279 = global read "全局 所有参数.vi" "CODMn"() -> (w360:string[][])
                          }
                          frame 4 {
                            n280 = global read "全局 所有参数.vi" "CODCr"() -> (w361:string[][])
                          }
                        }
                        n281 = Array Size(array=w353) -> (size(s)=w355:i32[])
                        n282 = Index Array(array=w355) -> (element=w354:i32)  [unwired: 1 in]
                        n283 = Greater Than 0?(x=w354) -> (x > 0?=w356:bool)
                        n284 = case shown="真" w356 {
                          tunnel: w352 -> [_ w367]
                          tunnel: w354 -> [_ _]
                          tunnel: w353 -> [_ w365]
                          frame False {
                          }
                          frame True {
                            # "最新时间戳加1分钟"
                            n285 = Index Array(array=w365, index (row)=0 ("禁用的索引 (行)"), index (col)=0 ("禁用的索引 (列)")) -> (element=w364:string)
                            n286 = call "日期时间字符串转换分钟数加一.vi"("data[0]"=w364) -> ("日期/时间字符串"=w363:string)  [unwired: 10 in]
                            n287 = case shown="3" w367 {
                              tunnel: w363 -> [w368 w369 w370 w371 w372]
                              frame 0, Default {
                                n288 = global write "全局 时间2.vi" "氨氮跨度核查索引起始时间"(w368) -> ()
                              }
                              frame 1 {
                                n289 = global write "全局 时间2.vi" "总氮跨度核查索引起始时间"(w369) -> ()
                              }
                              frame 2 {
                                n290 = global write "全局 时间2.vi" "总磷跨度核查索引起始时间"(w370) -> ()
                              }
                              frame 3 {
                                n291 = global write "全局 时间2.vi" "CODMn跨度核查索引起始时间"(w371) -> ()
                              }
                              frame 4 {
                                n292 = global write "全局 时间2.vi" "CODCr跨度核查索引起始时间"(w372) -> ()
                              }
                            }
                          }
                        }
                      }
                    }
                    frame #3 {
                      n293 = call <vilib>:"Application Directory.vi"() -> ("Application Directory"=w386:path)
                      n294 = call "数据处理整合 (子VI).vi"("枚举"=enum16{"实时数据排序", "小时数据排序"}."实时数据排序") -> ("已排序的数组"=w389:string[])  [unwired: 10 in]
                      n295 = Build Path(base path=w386, name or relative path="data\\hecha.ini" ("名称或相对路径")) -> (appended path=w384:path)
                      n296 = call <vilib>:"Open Config Data.vi"("configuration file path"=w384) -> ("error out"=w380:errorcluster, "refnum"=w383:T8)  [unwired: 8 in, 1 out]
                      n297 = Array Size(array=w389) -> (size(s)=w388:i32)
                      n298 = vi-ref "全局 时间2.vi"() -> (w382:refnum<vi>)
                      n299 = global write "全局 数据数组大小.vi" "数据数组大小"(w388) -> ()
                      n300 = call <userlib>:"Write Panel to INI__ogtk.vi"("error in (no error)"=w380, "VI ref"=w382, "refnum"=w383) -> ("error out"=w379:errorcluster, "refnum out"=w381:T8)  [unwired: 7 in]
                      n301 = call <vilib>:"Close Config Data.vi"("error in (no error)"=w379, "refnum"=w381) -> ("error out"=w374:errorcluster, "file path"=w373:path)  [unwired: 8 in]
                      n302 = Open/Create/Replace File(file path (use dialog)=w373, error in=w374) -> (refnum out=w377:refnum<file>, error out=w378:errorcluster)  [unwired: 4 in, 1 out]
                      n303 = Flush File(refnum=w377, error in=w378) -> (refnum out=w376:refnum<file>, error out=w375:errorcluster)
                      n304 = Close File(refnum=w376, error in=w375) -> ()  [unwired: 2 out]
                    }
                    frame #4 {
                      n305 = while {
                        stop <- w392 stop-if-true
                        n306 = property on="TCP服务端掉线计数" class="DigNum (严格)"() -> ("Value"=w396:i32)  [unwired: 2 in, 2 out]
                        n307 = property on="TCP服务端掉线计数" class="DigNum (严格)" props=["Value"]() -> ()  [unwired: 2 in, 3 out]
                        n308 = Greater Or Equal?(x=w396, y=1) -> (x >= y?=w395:bool)
                        n309 = case shown="假" w395 {
                          frame False {
                            n310 = global read "全局 数据数组大小.vi" "数据数组大小"() -> (w399:i32)
                            n311 = Greater Than 0?(x=w399) -> (x > 0?=w398:bool)
                            n312 = case shown="真" w398 {
                              frame False {
                              }
                              frame True {
                                w400 = 0 ("禁用的索引 (列)")
                                n313 = global read "插值后的新数组.vi" "插值后的数组元素"() -> (w410:T10)
                                n314 = local read "QN"() -> (w413:string)
                                n315 = local read "MN"() -> (w406:string)
                                n316 = local read "PW"() -> (w405:string)
                                n317 = local read "数据发送通道"() -> (w404:enum16{"TCP", "VISA"})
                                n318 = Unbundle By Name(w410) -> ("氨氮"=w409:string[][])
                                n319 = call "数据编码.vi"("table输入"="实时数据" ("新元素/子数组"), "QN"=w413, "MN"=w406, "PW"=w405) -> ("通讯包字符串"=w402:string)  [unwired: 10 in, 1 out]
                                n320 = local write "发送报文显示"(w402) -> ()
                                n321 = Index Array(array=w409, index (row)=w400, index (col)=w400) -> (element=w408:string)
                                n322 = call "VISATCP组合选择发送.vi"("数据发送通道"=w404, "命令"="write", "写入缓冲区"=w402) -> ("错误输出"=w401:errorcluster)  [unwired: 9 in, 3 out]
                                n323 = Build Array(w402) -> (w412:string[])
                                n324 = local write "核查数据上传"(TRUE ("数据上传")) -> ()
                                n325 = call "日期时间字符串转换分钟数加一.vi"("data[0]"=w408) -> ("日期/时间字符串"=w407:string)  [unwired: 10 in]
                                n326 = local write "错误输出"(w401) -> ()
                                n327 = call "发送数据记录到文档(子VI).vi"("数组"=w412) -> ()  [unwired: 9 in, 1 out]
                                n328 = global write "全局 时间2.vi" "跨度核查索引起始时间"(w407) -> ()
                              }
                            }
                          }
                          frame True {
                          }
                        }
                        n329 = Wait (ms)(milliseconds to wait=u32 500 ("等待时间（毫秒）")) -> ()  [unwired: 1 out]
                        n330 = global read "全局 数据数组大小.vi" "数据数组大小"() -> (w390:i32)
                        n331 = global read "全局 小时数据发送次数.vi" "小时数据发送次数"() -> (w394:i32)
                        n332 = Greater Or Equal?(x=w394, y=w390) -> (x >= y?=w393:bool)
                        n333 = Compound Arithmetic op=OR ("复合运算")(w393) -> (w392:bool)
                      }
                    }
                  }
                }
                frame "标样核查" {
                  n334 = flat-sequence {
                    tunnel: [w424] -> w415
                    frame #0 {
                      n335 = global write "全局 小时数据发送次数.vi" "小时数据发送次数"(0 ("小时数据发送次数")) -> ()
                      n336 = global write "全局 实时数据参数.vi" "实时数据参数"("核查数据") -> ()
                      n337 = global write "全局1.vi" "枚举"(enum16{"返回请求应答", "上传数据", "返回执行结果"}."上传数据" ("枚举")) -> ()
                    }
                    frame #1 {
                      n338 = call "从数据库获取数据通用可配置(子VI).vi"("table输入"="实时数据" ("新元素/子数组"), "列队名（唯一）"="n") -> ()  [unwired: 8 in, 2 out]
                    }
                    frame #2 {
                      n339 = call "数据处理整合 (子VI).vi"("枚举"=enum16{"实时数据排序", "小时数据排序"}."实时数据排序") -> ("已排序的数组"=w423:string[])  [unwired: 10 in]
                      n340 = Array Size(array=w423) -> (size(s)=w422:i32)
                      n341 = global write "全局 数据数组大小.vi" "数据数组大小"(w422) -> ()
                    }
                    frame #3 {
                      n342 = while {
                        tunnel: [w425] -> w424
                        stop <- w425 stop-if-true
                        n343 = property on="TCP服务端掉线计数" class="DigNum (严格)"() -> ("Value"=w431:i32)  [unwired: 2 in, 2 out]
                        n344 = property on="TCP服务端掉线计数" class="DigNum (严格)" props=["Value"]() -> ()  [unwired: 2 in, 3 out]
                        n345 = Greater Or Equal?(x=w431, y=1) -> (x >= y?=w430:bool)
                        n346 = case shown="假" w430 {
                          frame False {
                            n347 = global read "全局 数据数组大小.vi" "数据数组大小"() -> (w434:i32)
                            n348 = Greater Than 0?(x=w434) -> (x > 0?=w433:bool)
                            n349 = case shown="真" w433 {
                              frame False {
                              }
                              frame True {
                                w435 = 0 ("禁用的索引 (列)")
                                n350 = global read "插值后的新数组.vi" "插值后的数组元素"() -> (w445:T10)
                                n351 = local read "QN"() -> (w448:string)
                                n352 = local read "MN"() -> (w441:string)
                                n353 = local read "PW"() -> (w440:string)
                                n354 = local read "数据发送通道"() -> (w439:enum16{"TCP", "VISA"})
                                n355 = Unbundle By Name(w445) -> ("氨氮"=w444:string[][])
                                n356 = call "数据编码.vi"("table输入"="实时数据" ("新元素/子数组"), "QN"=w448, "MN"=w441, "PW"=w440) -> ("通讯包字符串"=w437:string)  [unwired: 10 in, 1 out]
                                n357 = local write "发送报文显示"(w437) -> ()
                                n358 = call "VISATCP组合选择发送.vi"("数据发送通道"=w439, "命令"="write", "写入缓冲区"=w437) -> ("错误输出"=w436:errorcluster)  [unwired: 9 in, 3 out]
                                n359 = Index Array(array=w444, index (row)=w435, index (col)=w435) -> (element=w443:string)
                                n360 = Build Array(w437) -> (w447:string[])
                                n361 = local write "核查数据上传"(TRUE ("数据上传")) -> ()
                                n362 = call "日期时间字符串转换分钟数加一.vi"("data[0]"=w443) -> ("日期/时间字符串"=w442:string)  [unwired: 10 in]
                                n363 = local write "错误输出"(w436) -> ()
                                n364 = call "发送数据记录到文档(子VI).vi"("数组"=w447) -> ()  [unwired: 9 in, 1 out]
                                n365 = global write "全局 时间2.vi" "标样核查索引起始时间"(w442) -> ()
                              }
                            }
                          }
                          frame True {
                          }
                        }
                        n366 = Wait (ms)(milliseconds to wait=u32 500 ("等待时间（毫秒）")) -> ()  [unwired: 1 out]
                        n367 = global read "全局 数据数组大小.vi" "数据数组大小"() -> (w426:i32)
                        n368 = global read "全局 小时数据发送次数.vi" "小时数据发送次数"() -> (w429:i32)
                        n369 = Greater Or Equal?(x=w429, y=w426) -> (x >= y?=w428:bool)
                        n370 = Compound Arithmetic op=OR ("复合运算")(w428) -> (w425:bool)
                      }
                    }
                  }
                }
                frame "加标回收" {
                  n371 = flat-sequence {
                    frame #0 {
                      n372 = global write "全局 小时数据发送次数.vi" "小时数据发送次数"(0 ("小时数据发送次数")) -> ()
                      n373 = global write "全局 实时数据参数.vi" "实时数据参数"("加标回收测试") -> ()
                      n374 = global write "全局1.vi" "枚举"(enum16{"返回请求应答", "上传数据", "返回执行结果"}."上传数据" ("枚举")) -> ()
                    }
                    frame #1 {
                      n375 = call "从数据库获取数据通用可配置(子VI).vi"("table输入"="加标回收" ("新元素/子数组"), "列队名（唯一）"="d") -> ()  [unwired: 8 in, 2 out]
                    }
                    frame #2 {
                      n376 = call "加标回收数据处理整合 (子VI).vi"("枚举"=enum16{"实时数据排序", "小时数据排序"}."实时数据排序") -> ("已排序的数组"=w456:string[])  [unwired: 10 in]
                      n377 = Array Size(array=w456) -> (size(s)=w457:i32)
                      n378 = global write "全局 数据数组大小.vi" "数据数组大小"(w457) -> ()
                    }
                    frame #3 {
                      n379 = while {
                        stop <- w460 stop-if-true
                        n380 = property on="TCP服务端掉线计数" class="DigNum (严格)"() -> ("Value"=w465:i32)  [unwired: 2 in, 2 out]
                        n381 = Greater Or Equal?(x=w465, y=1) -> (x >= y?=w463:bool)
                        n382 = case shown="假" w463 {
                          frame False {
                            n383 = global read "全局 数据数组大小.vi" "数据数组大小"() -> (w467:i32)
                            n384 = Greater Than 0?(x=w467) -> (x > 0?=w466:bool)
                            n385 = case shown="真" w466 {
                              frame False {
                              }
                              frame True {
                                n386 = global read "全局 数据数组大小.vi" "数据数组大小"() -> (w477:i32)
                                n387 = global read "插值后的新数组.vi" "插值后的数组元素"() -> (w480:T10)
                                n388 = local read "MN"() -> (w473:string)
                                n389 = local read "PW"() -> (w472:string)
                                n390 = local read "数据发送通道"() -> (w471:enum16{"TCP", "VISA"})
                                n391 = Decrement(x=w477) -> (x-1=w476:i32)
                                n392 = call "数据编码.vi"("table输入"="实时数据" ("新元素/子数组"), "MN"=w473, "PW"=w472) -> ("通讯包字符串"=w469:string)  [unwired: 11 in, 1 out]
                                n393 = Unbundle By Name(w480) -> ("氨氮"=w479:string[][])
                                n394 = local write "发送报文显示"(w469) -> ()
                                n395 = call "VISATCP组合选择发送.vi"("数据发送通道"=w471, "命令"="write", "写入缓冲区"=w469) -> ("错误输出"=w468:errorcluster)  [unwired: 9 in, 3 out]
                                n396 = Index Array(array=w479, index (row)=w476, index (col)=0 ("禁用的索引 (列)")) -> (element=w475:string)
                                n397 = local write "核查数据上传"(TRUE ("数据上传")) -> ()
                                n398 = Build Array(w469) -> (w482:string[])
                                n399 = call "日期时间字符串转换分钟数加一.vi"("data[0]"=w475) -> ("日期/时间字符串"=w474:string)  [unwired: 10 in]
                                n400 = local write "错误输出"(w468) -> ()
                                n401 = call "发送数据记录到文档(子VI).vi"("数组"=w482) -> ()  [unwired: 9 in, 1 out]
                                n402 = global write "全局 时间2.vi" "加标回收索引起始时间"(w474) -> ()
                              }
                            }
                          }
                          frame True {
                          }
                        }
                        n403 = Wait (ms)(milliseconds to wait=u32 500 ("等待时间（毫秒）")) -> ()  [unwired: 1 out]
                        n404 = global read "全局 数据数组大小.vi" "数据数组大小"() -> (w458:i32)
                        n405 = global read "全局 小时数据发送次数.vi" "小时数据发送次数"() -> (w462:i32)
                        n406 = Greater Or Equal?(x=w462, y=w458) -> (x >= y?=w461:bool)
                        n407 = Compound Arithmetic op=OR ("复合运算")(w461) -> (w460:bool)
                      }
                    }
                  }
                }
                frame "平行样" {
                  n408 = flat-sequence {
                    frame #0 {
                      n409 = global write "全局 小时数据发送次数.vi" "小时数据发送次数"(0 ("小时数据发送次数")) -> ()
                      n410 = global write "全局 实时数据参数.vi" "实时数据参数"("平行样测试") -> ()
                      n411 = global write "全局1.vi" "枚举"(enum16{"返回请求应答", "上传数据", "返回执行结果"}."上传数据" ("枚举")) -> ()
                    }
                    frame #1 {
                      n412 = call "从数据库获取数据通用可配置(子VI).vi"("table输入"="平行样测试" ("新元素/子数组"), "列队名（唯一）"="e") -> ()  [unwired: 8 in, 2 out]
                    }
                    frame #2 {
                      n413 = for {
                        N: 5 -> [_]
                        i -> [w490]
                        # "行数大于零"
                        n414 = case shown="3" w490 {
                          tunnel: [w495 w496 w497 w498 w499] -> w491
                          frame 0, Default {
                            n415 = global read "全局 所有参数.vi" "氨氮"() -> (w495:string[][])
                          }
                          frame 1 {
                            n416 = global read "全局 所有参数.vi" "总氮"() -> (w496:string[][])
                          }
                          frame 2 {
                            n417 = global read "全局 所有参数.vi" "总磷"() -> (w497:string[][])
                          }
                          frame 3 {
                            n418 = global read "全局 所有参数.vi" "CODMn"() -> (w498:string[][])
                          }
                          frame 4 {
                            n419 = global read "全局 所有参数.vi" "CODCr"() -> (w499:string[][])
                          }
                        }
                        n420 = Array Size(array=w491) -> (size(s)=w493:i32[])
                        n421 = Index Array(array=w493) -> (element=w492:i32)  [unwired: 1 in]
                        n422 = Greater Than 0?(x=w492) -> (x > 0?=w494:bool)
                        n423 = case shown="真" w494 {
                          tunnel: w490 -> [_ w505]
                          tunnel: w492 -> [_ _]
                          tunnel: w491 -> [_ w503]
                          frame False {
                          }
                          frame True {
                            # "最新时间戳加1分钟"
                            n424 = Index Array(array=w503, index (row)=0 ("禁用的索引 (行)"), index (col)=0 ("禁用的索引 (列)")) -> (element=w502:string)
                            n425 = call "日期时间字符串转换分钟数加一.vi"("data[0]"=w502) -> ("日期/时间字符串"=w501:string)  [unwired: 10 in]
                            n426 = case shown="0, 默认" w505 {
                              tunnel: w501 -> [w506 w507 w508 w509 w510]
                              frame 0, Default {
                                n427 = global write "全局 时间2.vi" "氨氮平行样索引起始时间"(w506) -> ()
                              }
                              frame 1 {
                                n428 = global write "全局 时间2.vi" "总氮平行样索引起始时间"(w507) -> ()
                              }
                              frame 2 {
                                n429 = global write "全局 时间2.vi" "总磷平行样索引起始时间"(w508) -> ()
                              }
                              frame 3 {
                                n430 = global write "全局 时间2.vi" "CODMn平行样索引起始时间"(w509) -> ()
                              }
                              frame 4 {
                                n431 = global write "全局 时间2.vi" "CODCr平行样索引起始时间"(w510) -> ()
                              }
                            }
                          }
                        }
                      }
                    }
                    frame #3 {
                      n432 = call "数据处理整合 (子VI).vi"("枚举"=enum16{"实时数据排序", "小时数据排序"}."实时数据排序") -> ("已排序的数组"=w527:string[])  [unwired: 10 in]
                      n433 = Array Size(array=w527) -> (size(s)=w526:i32)
                      n434 = call <vilib>:"Application Directory.vi"() -> ("Application Directory"=w524:path)
                      n435 = Build Path(base path=w524, name or relative path="data\\hecha.ini" ("名称或相对路径")) -> (appended path=w522:path)
                      n436 = global write "全局 数据数组大小.vi" "数据数组大小"(w526) -> ()
                      n437 = call <vilib>:"Open Config Data.vi"("configuration file path"=w522) -> ("error out"=w518:errorcluster, "refnum"=w521:T8)  [unwired: 8 in, 1 out]
                      n438 = vi-ref "全局 时间2.vi"() -> (w520:refnum<vi>)
                      n439 = call <userlib>:"Write Panel to INI__ogtk.vi"("error in (no error)"=w518, "VI ref"=w520, "refnum"=w521) -> ("error out"=w517:errorcluster, "refnum out"=w519:T8)  [unwired: 7 in]
                      n440 = call <vilib>:"Close Config Data.vi"("error in (no error)"=w517, "refnum"=w519) -> ("error out"=w512:errorcluster, "file path"=w511:path)  [unwired: 8 in]
                      n441 = Open/Create/Replace File(file path (use dialog)=w511, error in=w512) -> (refnum out=w515:refnum<file>, error out=w516:errorcluster)  [unwired: 4 in, 1 out]
                      n442 = Flush File(refnum=w515, error in=w516) -> (refnum out=w514:refnum<file>, error out=w513:errorcluster)
                      n443 = Close File(refnum=w514, error in=w513) -> ()  [unwired: 2 out]
                    }
                    frame #4 {
                      n444 = while {
                        stop <- w530 stop-if-true
                        n445 = property on="TCP服务端掉线计数" class="DigNum (严格)"() -> ("Value"=w536:i32)  [unwired: 2 in, 2 out]
                        n446 = property on="TCP服务端掉线计数" class="DigNum (严格)" props=["Value"]() -> ()  [unwired: 2 in, 3 out]
                        n447 = Greater Or Equal?(x=w536, y=1) -> (x >= y?=w534:bool)
                        n448 = case shown="假" w534 {
                          frame False {
                            n449 = global read "全局 数据数组大小.vi" "数据数组大小"() -> (w538:i32)
                            n450 = Greater Than 0?(x=w538) -> (x > 0?=w537:bool)
                            n451 = case shown="真" w537 {
                              frame False {
                              }
                              frame True {
                                n452 = local read "MN"() -> (w544:string)
                                n453 = local read "PW"() -> (w543:string)
                                n454 = local read "数据发送通道"() -> (w542:enum16{"TCP", "VISA"})
                                n455 = local write "核查数据上传"(TRUE ("数据上传")) -> ()
                                n456 = call "数据编码.vi"("table输入"="实时数据" ("新元素/子数组"), "MN"=w544, "PW"=w543) -> ("通讯包字符串"=w540:string)  [unwired: 11 in, 1 out]
                                n457 = local write "发送报文显示"(w540) -> ()
                                n458 = call "VISATCP组合选择发送.vi"("数据发送通道"=w542, "命令"="write", "写入缓冲区"=w540) -> ("错误输出"=w539:errorcluster)  [unwired: 9 in, 3 out]
                                n459 = Build Array(w540) -> (w546:string[])
                                n460 = call "发送数据记录到文档(子VI).vi"("数组"=w546) -> ()  [unwired: 9 in, 1 out]
                                n461 = local write "错误输出"(w539) -> ()
                              }
                            }
                          }
                          frame True {
                          }
                        }
                        n462 = Wait (ms)(milliseconds to wait=u32 500 ("等待时间（毫秒）")) -> ()  [unwired: 1 out]
                        n463 = global read "全局 数据数组大小.vi" "数据数组大小"() -> (w533:i32)
                        n464 = global read "全局 小时数据发送次数.vi" "小时数据发送次数"() -> (w532:i32)
                        n465 = Decrement(x=w533) -> (x-1=w529:i32)
                        n466 = Greater Or Equal?(x=w532, y=w529) -> (x >= y?=w531:bool)
                        n467 = Compound Arithmetic op=OR ("复合运算")(w531) -> (w530:bool)
                      }
                    }
                  }
                }
                frame "集成干预" {
                  n468 = flat-sequence {
                    frame #0 {
                      n469 = global write "全局 小时数据发送次数.vi" "小时数据发送次数"(0 ("小时数据发送次数")) -> ()
                      n470 = global write "全局 实时数据参数.vi" "实时数据参数"("集成干预测试") -> ()
                      n471 = global write "全局1.vi" "枚举"(enum16{"返回请求应答", "上传数据", "返回执行结果"}."上传数据" ("枚举")) -> ()
                    }
                    frame #1 {
                      n472 = call "从数据库获取数据通用可配置(子VI).vi"("table输入"="集成干预测试" ("新元素/子数组"), "列队名（唯一）"="f") -> ()  [unwired: 8 in, 2 out]
                    }
                    frame #2 {
                      n473 = for {
                        N: 10 -> [_]
                        i -> [w554]
                        # "行数大于零"
                        n474 = case shown="9" w554 {
                          tunnel: [w559 w560 w561 w562 w563 w564 w565 w566 w567 w568] -> w555
                          frame 0, Default {
                            n475 = global read "全局 所有参数.vi" "氨氮"() -> (w559:string[][])
                          }
                          frame 1 {
                            n476 = global read "全局 所有参数.vi" "总氮"() -> (w560:string[][])
                          }
                          frame 2 {
                            n477 = global read "全局 所有参数.vi" "总磷"() -> (w561:string[][])
                          }
                          frame 3 {
                            n478 = global read "全局 所有参数.vi" "CODMn"() -> (w562:string[][])
                          }
                          frame 4 {
                            n479 = global read "全局 所有参数.vi" "CODCr"() -> (w563:string[][])
                          }
                          frame 5 {
                            n480 = global read "全局 所有参数.vi" "DO"() -> (w564:string[][])
                          }
                          frame 6 {
                            n481 = global read "全局 所有参数.vi" "PH"() -> (w565:string[][])
                          }
                          frame 7 {
                            n482 = global read "全局 所有参数.vi" "电导率"() -> (w566:string[][])
                          }
                          frame 8 {
                            n483 = global read "全局 所有参数.vi" "水温"() -> (w567:string[][])
                          }
                          frame 9 {
                            n484 = global read "全局 所有参数.vi" "浊度"() -> (w568:string[][])
                          }
                        }
                        n485 = Array Size(array=w555) -> (size(s)=w557:i32[])
                        n486 = Index Array(array=w557) -> (element=w556:i32)  [unwired: 1 in]
                        n487 = Greater Than 0?(x=w556) -> (x > 0?=w558:bool)
                        n488 = case shown="真" w558 {
                          tunnel: w554 -> [_ w574]
                          tunnel: w556 -> [_ _]
                          tunnel: w555 -> [_ w572]
                          frame False {
                          }
                          frame True {
                            # "最新时间戳加1分钟"
                            n489 = Index Array(array=w572, index (row)=0 ("禁用的索引 (行)"), index (col)=0 ("禁用的索引 (列)")) -> (element=w571:string)
                            n490 = call "日期时间字符串转换分钟数加一.vi"("data[0]"=w571) -> ("日期/时间字符串"=w570:string)  [unwired: 10 in]
                            n491 = case shown="9" w574 {
                              tunnel: w570 -> [w575 w576 w577 w578 w579 w580 w581 w582 w583 w584]
                              frame 0, Default {
                                n492 = global write "全局 时间2.vi" "氨氮集成干预索引起始时间"(w575) -> ()
                              }
                              frame 1 {
                                n493 = global write "全局 时间2.vi" "总氮集成干预索引起始时间"(w576) -> ()
                              }
                              frame 2 {
                                n494 = global write "全局 时间2.vi" "总磷集成干预索引起始时间"(w577) -> ()
                              }
                              frame 3 {
                                n495 = global write "全局 时间2.vi" "CODMn集成干预索引起始时间"(w578) -> ()
                              }
                              frame 4 {
                                n496 = global write "全局 时间2.vi" "CODCr集成干预索引起始时间"(w579) -> ()
                              }
                              frame 5 {
                                n497 = global write "全局 时间2.vi" "DO集成干预索引起始时间"(w580) -> ()
                              }
                              frame 6 {
                                n498 = global write "全局 时间2.vi" "PH集成干预索引起始时间"(w581) -> ()
                              }
                              frame 7 {
                                n499 = global write "全局 时间2.vi" "比电导率集成干预索引起始时间"(w582) -> ()
                              }
                              frame 8 {
                                n500 = global write "全局 时间2.vi" "水温集成干预索引起始时间"(w583) -> ()
                              }
                              frame 9 {
                                n501 = global write "全局 时间2.vi" "浊度集成干预索引起始时间"(w584) -> ()
                              }
                            }
                          }
                        }
                      }
                    }
                    frame #3 {
                      n502 = call "数据处理整合 (子VI).vi"("枚举"=enum16{"实时数据排序", "小时数据排序"}."实时数据排序") -> ("已排序的数组"=w601:string[])  [unwired: 10 in]
                      n503 = Array Size(array=w601) -> (size(s)=w600:i32)
                      n504 = call <vilib>:"Application Directory.vi"() -> ("Application Directory"=w598:path)
                      n505 = Build Path(base path=w598, name or relative path="data\\hecha.ini" ("名称或相对路径")) -> (appended path=w596:path)
                      n506 = global write "全局 数据数组大小.vi" "数据数组大小"(w600) -> ()
                      n507 = call <vilib>:"Open Config Data.vi"("configuration file path"=w596) -> ("error out"=w592:errorcluster, "refnum"=w595:T8)  [unwired: 8 in, 1 out]
                      n508 = vi-ref "全局 时间2.vi"() -> (w594:refnum<vi>)
                      n509 = call <userlib>:"Write Panel to INI__ogtk.vi"("error in (no error)"=w592, "VI ref"=w594, "refnum"=w595) -> ("error out"=w591:errorcluster, "refnum out"=w593:T8)  [unwired: 7 in]
                      n510 = call <vilib>:"Close Config Data.vi"("error in (no error)"=w591, "refnum"=w593) -> ("error out"=w586:errorcluster, "file path"=w585:path)  [unwired: 8 in]
                      n511 = Open/Create/Replace File(file path (use dialog)=w585, error in=w586) -> (refnum out=w589:refnum<file>, error out=w590:errorcluster)  [unwired: 4 in, 1 out]
                      n512 = Flush File(refnum=w589, error in=w590) -> (refnum out=w588:refnum<file>, error out=w587:errorcluster)
                      n513 = Close File(refnum=w588, error in=w587) -> ()  [unwired: 2 out]
                    }
                    frame #4 {
                      n514 = while {
                        stop <- w604 stop-if-true
                        n515 = property on="TCP服务端掉线计数" class="DigNum (严格)"() -> ("Value"=w610:i32)  [unwired: 2 in, 2 out]
                        n516 = property on="TCP服务端掉线计数" class="DigNum (严格)" props=["Value"]() -> ()  [unwired: 2 in, 3 out]
                        n517 = Greater Or Equal?(x=w610, y=1) -> (x >= y?=w608:bool)
                        n518 = case shown="假" w608 {
                          frame False {
                            n519 = global read "全局 数据数组大小.vi" "数据数组大小"() -> (w612:i32)
                            n520 = Greater Than 0?(x=w612) -> (x > 0?=w611:bool)
                            n521 = case shown="真" w611 {
                              frame False {
                              }
                              frame True {
                                n522 = local read "MN"() -> (w618:string)
                                n523 = local read "PW"() -> (w617:string)
                                n524 = local read "数据发送通道"() -> (w616:enum16{"TCP", "VISA"})
                                n525 = local write "核查数据上传"(TRUE ("数据上传")) -> ()
                                n526 = call "数据编码.vi"("table输入"="实时数据" ("新元素/子数组"), "MN"=w618, "PW"=w617) -> ("通讯包字符串"=w614:string)  [unwired: 11 in, 1 out]
                                n527 = local write "发送报文显示"(w614) -> ()
                                n528 = call "VISATCP组合选择发送.vi"("数据发送通道"=w616, "命令"="write", "写入缓冲区"=w614) -> ("错误输出"=w613:errorcluster)  [unwired: 9 in, 3 out]
                                n529 = Build Array(w614) -> (w620:string[])
                                n530 = call "发送数据记录到文档(子VI).vi"("数组"=w620) -> ()  [unwired: 9 in, 1 out]
                                n531 = local write "错误输出"(w613) -> ()
                              }
                            }
                          }
                          frame True {
                          }
                        }
                        n532 = Wait (ms)(milliseconds to wait=u32 500 ("等待时间（毫秒）")) -> ()  [unwired: 1 out]
                        n533 = global read "全局 数据数组大小.vi" "数据数组大小"() -> (w607:i32)
                        n534 = global read "全局 小时数据发送次数.vi" "小时数据发送次数"() -> (w606:i32)
                        n535 = Decrement(x=w607) -> (x-1=w603:i32)
                        n536 = Greater Or Equal?(x=w606, y=w603) -> (x >= y?=w605:bool)
                        n537 = Compound Arithmetic op=OR ("复合运算")(w605) -> (w604:bool)
                      }
                    }
                  }
                }
                frame "", Default {
                  n538 = Get Queue Status(queue=w625) -> (# elements in queue=w624:i32)  [unwired: 2 in, 7 out]
                  n539 = Equal To 0?(x=w624) -> (x = 0?=w623:bool)
                  n540 = case shown="真" w623 {
                    tunnel: [_ TRUE] -> w622
                    frame False {
                    }
                    frame True {
                    }
                  }
                }
              }
              n541 = Wait (ms)(milliseconds to wait=u32 1000 ("等待时间（毫秒）")) -> ()  [unwired: 1 out]
            }
          }
          frame "小时数据" {
            # "间隔时间上传"
            n542 = flat-sequence {
              frame #0 {
                # "发送前2小时的数据"
                n543 = global write "全局 小时数据发送次数.vi" "小时数据发送次数"(1 ("小时数据发送次数")) -> ()
                n544 = global write "全局1.vi" "枚举"(enum16{"返回请求应答", "上传数据", "返回执行结果"}."上传数据" ("枚举")) -> ()
              }
              frame #1 {
                n545 = call "从数据库获取数据通用可配置(子VI).vi"("table输入"="小时数据" ("新元素/子数组"), "列队名（唯一）"="XS" ("名称（未命名）")) -> ()  [unwired: 8 in, 2 out]
              }
              frame #2 {
                n546 = property on="TCP服务端掉线计数" class="DigNum (严格)"() -> ("Value"=w632:i32)  [unwired: 2 in, 2 out]
                n547 = Greater Or Equal?(x=w632, y=1) -> (x >= y?=w631:bool)
                n548 = case shown="假" w631 {
                  frame False {
                    # "数据处理整合"
                    n549 = call "实时小时数据处理整合 (子VI).vi"("枚举"=enum16{"实时数据排序", "小时数据排序"}."小时数据排序") -> ("已排序的数组"=w634:string[])  [unwired: 10 in]
                    n550 = Array Size(array=w634) -> (size(s)=w637:i32)
                    n551 = global write "全局 数据数组大小.vi" "数据数组大小"(1 ("数据数组大小")) -> ()
                    n552 = Greater Than 0?(x=w637) -> (x > 0?=w638:bool)
                    n553 = case shown="真" w638 {
                      frame False {
                      }
                      frame True {
                        n554 = local write "核查数据上传"(TRUE ("数据上传")) -> ()
                        n555 = Get Date/Time In Seconds() -> (seconds since 1Jan1904=w649:timestamp)
                        n556 = Format Date/Time String(time format string (%c)="%Y%m%d%H%M%S%3u" ("时间格式字符串(%c)"), seconds (now)=w649) -> (date/time string=w650:string)  [unwired: 1 in]
                        n557 = local read "MN"() -> (w644:string)
                        n558 = local read "PW"() -> (w643:string)
                        n559 = Search and Replace String(input string=w650, search string="." ("搜索字符串")) -> (result string=w652:string)  [unwired: 6 in, 3 out]
                        n560 = local read "数据发送通道"() -> (w642:enum16{"TCP", "VISA"})
                        n561 = call "数据编码.vi"("table输入"="小时数据" ("新元素/子数组"), "QN"=w652, "MN"=w644, "PW"=w643) -> ("通讯包字符串"=w640:string)  [unwired: 10 in, 1 out]
                        n562 = local write "发送报文显示"(w640) -> ()
                        n563 = call "VISATCP组合选择发送.vi"("数据发送通道"=w642, "命令"="write", "写入缓冲区"=w640) -> ("错误输出"=w639:errorcluster)  [unwired: 9 in, 3 out]
                        n564 = Build Array(w640) -> (w646:string[])
                        n565 = local write "错误输出"(w639) -> ()
                        n566 = call "发送数据记录到文档(子VI).vi"("数组"=w646) -> ()  [unwired: 9 in, 1 out]
                      }
                    }
                  }
                  frame True {
                  }
                }
              }
            }
          }
          frame "操作日志" {
            # "间隔时间上传"
            # "直接1分钟查询 一次,有数据就按数据上传,没数据就不上传,在数据发送那边有做处理"
            n567 = flat-sequence {
              frame #0 {
                # "时间"
                n568 = global read "全局 数据发送重叠.vi" "数据发送重叠开始时间戳"() -> (w654:string)
                n569 = global read "全局 数据发送重叠.vi" "数据发送重叠"() -> (w653:bool)
                n570 = global write "全局 小时数据发送次数.vi" "小时数据发送次数"(0 ("小时数据发送次数")) -> ()
                n571 = global write "全局1.vi" "枚举"(enum16{"返回请求应答", "上传数据", "返回执行结果"}."上传数据" ("枚举")) -> ()
                n572 = call "日志信息主动发送(子VI).vi"("是否正在查询数据"=w653, "查询数据发送时间节点"=w654) -> ()  [unwired: 10 in]
              }
              frame #1 {
                n573 = call "获取操作日志 (子VI).vi"("table输入"="操作日志") -> ()  [unwired: 11 in]
              }
              frame #2 {
                n574 = call "数据处理整合 (子VI).vi"("枚举"=enum16{"实时数据排序", "小时数据排序"}."实时数据排序") -> ("已排序的数组"=w660:string[])  [unwired: 10 in]
                n575 = Array Size(array=w660) -> (size(s)=w659:i32)
                n576 = global write "全局 数据数组大小.vi" "数据数组大小"(w659) -> ()
              }
              frame #3 {
                n577 = while {
                  stop <- w661 stop-if-true
                  # "判定是否存表"
                  n578 = property on="TCP服务端掉线计数" class="DigNum (严格)"() -> ("Value"=w667:i32)  [unwired: 2 in, 2 out]
                  n579 = Greater Or Equal?(x=w667, y=1) -> (x >= y?=w666:bool)
                  n580 = case shown="假" w666 {
                    frame False {
                      n581 = global read "全局 数据数组大小.vi" "数据数组大小"() -> (w669:i32)
                      n582 = Greater Than 0?(x=w669) -> (x > 0?=w670:bool)
                      n583 = case shown="真" w670 {
                        frame False {
                        }
                        frame True {
                          n584 = global read "全局 小时数据发送次数.vi" "小时数据发送次数"() -> (w679:i32)
                          n585 = local write "核查数据上传"(TRUE ("数据上传")) -> ()
                          n586 = Get Date/Time In Seconds() -> (seconds since 1Jan1904=w684:timestamp)
                          n587 = Increment(x=w679) -> (x+1=w678:i32)
                          n588 = Format Date/Time String(time format string (%c)="%Y%m%d%H%M%S%3u" ("时间格式字符串(%c)"), seconds (now)=w684) -> (date/time string=w683:string)  [unwired: 1 in]
                          n589 = global write "全局 小时数据发送次数.vi" "小时数据发送次数"(w678) -> ()
                          n590 = Search and Replace String(input string=w683, search string="." ("搜索字符串")) -> (result string=w681:string)  [unwired: 6 in, 3 out]
                          n591 = local read "MN"() -> (w676:string)
                          n592 = local read "PW"() -> (w675:string)
                          n593 = call "数据编码.vi"("table输入"="操作日志" ("新元素/子数组"), "QN"=w681, "MN"=w676, "PW"=w675) -> ("通讯包字符串"=w672:string)  [unwired: 10 in, 1 out]
                          n594 = local read "数据发送通道"() -> (w674:enum16{"TCP", "VISA"})
                          n595 = local write "发送报文显示"(w672) -> ()
                          n596 = call "VISATCP组合选择发送.vi"("数据发送通道"=w674, "命令"="write", "写入缓冲区"=w672) -> ("错误输出"=w671:errorcluster)  [unwired: 9 in, 3 out]
                          n597 = Build Array(w672) -> (w680:string[])
                          n598 = local write "错误输出"(w671) -> ()
                          n599 = call "发送数据记录到文档(子VI).vi"("数组"=w680) -> ()  [unwired: 9 in, 1 out]
                        }
                      }
                    }
                    frame True {
                    }
                  }
                  n600 = Wait (ms)(milliseconds to wait=u32 500 ("等待时间（毫秒）")) -> ()  [unwired: 1 out]
                  n601 = global read "全局 数据数组大小.vi" "数据数组大小"() -> (w663:i32)
                  n602 = global read "全局 小时数据发送次数.vi" "小时数据发送次数"() -> (w665:i32)
                  n603 = Decrement(x=w663) -> (x-1=w662:i32)
                  n604 = Greater Or Equal?(x=w665, y=w662) -> (x >= y?=w661:bool)
                }
              }
            }
          }
          frame "仪器参数" {
            # "间隔时间上传"
            # "直接1分钟查询 一次,有数据就按数据上传,没数据就不上传,在数据发送那边有做处理"
            n605 = flat-sequence {
              frame #0 {
                # "时间"
                n606 = global read "全局 数据发送重叠.vi" "数据发送重叠开始时间戳"() -> (w688:string)
                n607 = global read "全局 数据发送重叠.vi" "数据发送重叠"() -> (w687:bool)
                n608 = global write "全局 小时数据发送次数.vi" "小时数据发送次数"(0 ("小时数据发送次数")) -> ()
                n609 = global write "全局1.vi" "枚举"(enum16{"返回请求应答", "上传数据", "返回执行结果"}."上传数据" ("枚举")) -> ()
                n610 = call "日志信息主动发送(子VI).vi"("是否正在查询数据"=w687, "查询数据发送时间节点"=w688) -> ()  [unwired: 10 in]
              }
              frame #1 {
                n611 = call "获取操作日志 (子VI).vi"("table输入"="仪器参数") -> ()  [unwired: 11 in]
              }
              frame #2 {
                n612 = call "数据处理整合 (子VI).vi"("枚举"=enum16{"实时数据排序", "小时数据排序"}."实时数据排序") -> ("已排序的数组"=w694:string[])  [unwired: 10 in]
                n613 = Array Size(array=w694) -> (size(s)=w693:i32)
                n614 = global write "全局 数据数组大小.vi" "数据数组大小"(w693) -> ()
              }
              frame #3 {
                n615 = while {
                  stop <- w695 stop-if-true
                  # "判定是否存表"
                  n616 = property on="TCP服务端掉线计数" class="DigNum (严格)"() -> ("Value"=w701:i32)  [unwired: 2 in, 2 out]
                  n617 = Greater Or Equal?(x=w701, y=1) -> (x >= y?=w700:bool)
                  n618 = case shown="假" w700 {
                    frame False {
                      n619 = global read "全局 数据数组大小.vi" "数据数组大小"() -> (w703:i32)
                      n620 = Greater Than 0?(x=w703) -> (x > 0?=w704:bool)
                      n621 = case shown="真" w704 {
                        frame False {
                        }
                        frame True {
                          n622 = global read "全局 小时数据发送次数.vi" "小时数据发送次数"() -> (w713:i32)
                          n623 = local write "核查数据上传"(TRUE ("数据上传")) -> ()
                          n624 = Get Date/Time In Seconds() -> (seconds since 1Jan1904=w718:timestamp)
                          n625 = Increment(x=w713) -> (x+1=w712:i32)
                          n626 = Format Date/Time String(time format string (%c)="%Y%m%d%H%M%S%3u" ("时间格式字符串(%c)"), seconds (now)=w718) -> (date/time string=w717:string)  [unwired: 1 in]
                          n627 = global write "全局 小时数据发送次数.vi" "小时数据发送次数"(w712) -> ()
                          n628 = Search and Replace String(input string=w717, search string="." ("搜索字符串")) -> (result string=w715:string)  [unwired: 6 in, 3 out]
                          n629 = local read "MN"() -> (w710:string)
                          n630 = local read "PW"() -> (w709:string)
                          n631 = call "数据编码.vi"("table输入"="仪器参数" ("新元素/子数组"), "QN"=w715, "MN"=w710, "PW"=w709) -> ("通讯包字符串"=w706:string)  [unwired: 10 in, 1 out]
                          n632 = local read "数据发送通道"() -> (w708:enum16{"TCP", "VISA"})
                          n633 = local write "发送报文显示"(w706) -> ()
                          n634 = call "VISATCP组合选择发送.vi"("数据发送通道"=w708, "命令"="write", "写入缓冲区"=w706) -> ("错误输出"=w705:errorcluster)  [unwired: 9 in, 3 out]
                          n635 = Build Array(w706) -> (w714:string[])
                          n636 = local write "错误输出"(w705) -> ()
                          n637 = call "发送数据记录到文档(子VI).vi"("数组"=w714) -> ()  [unwired: 9 in, 1 out]
                        }
                      }
                    }
                    frame True {
                    }
                  }
                  n638 = Wait (ms)(milliseconds to wait=u32 500 ("等待时间（毫秒）")) -> ()  [unwired: 1 out]
                  n639 = global read "全局 数据数组大小.vi" "数据数组大小"() -> (w697:i32)
                  n640 = global read "全局 小时数据发送次数.vi" "小时数据发送次数"() -> (w699:i32)
                  n641 = Decrement(x=w697) -> (x-1=w696:i32)
                  n642 = Greater Or Equal?(x=w699, y=w696) -> (x >= y?=w695:bool)
                }
              }
            }
          }
          frame "系统状态" {
            # "直接1分钟查询 一次,有变化就按上传,没变化就不上传"
            n643 = flat-sequence {
              frame #0 {
                # "时间"
                n644 = global write "全局 小时数据发送次数.vi" "小时数据发送次数"(0 ("小时数据发送次数")) -> ()
                n645 = global write "全局 数据数组大小.vi" "数据数组大小"(1 ("数据数组大小")) -> ()
                n646 = global write "全局1.vi" "枚举"(enum16{"返回请求应答", "上传数据", "返回执行结果"}."上传数据" ("枚举")) -> ()
              }
              frame #1 {
                # "判定是否存表"
                n647 = property on="TCP服务端掉线计数" class="DigNum (严格)"() -> ("Value"=w725:i32)  [unwired: 2 in, 2 out]
                n648 = Greater Or Equal?(x=w725, y=1) -> (x >= y?=w724:bool)
                n649 = case shown="假" w724 {
                  frame False {
                    n650 = global read "全局 数据数组大小.vi" "数据数组大小"() -> (w727:i32)
                    n651 = Greater Than 0?(x=w727) -> (x > 0?=w728:bool)
                    n652 = case shown="真" w728 {
                      frame False {
                      }
                      frame True {
                        n653 = global read "全局 小时数据发送次数.vi" "小时数据发送次数"() -> (w737:i32)
                        n654 = local write "核查数据上传"(TRUE ("数据上传")) -> ()
                        n655 = Get Date/Time In Seconds() -> (seconds since 1Jan1904=w742:timestamp)
                        n656 = Increment(x=w737) -> (x+1=w736:i32)
                        n657 = Format Date/Time String(time format string (%c)="%Y%m%d%H%M%S%3u" ("时间格式字符串(%c)"), seconds (now)=w742) -> (date/time string=w741:string)  [unwired: 1 in]
                        n658 = global write "全局 小时数据发送次数.vi" "小时数据发送次数"(w736) -> ()
                        n659 = Search and Replace String(input string=w741, search string="." ("搜索字符串")) -> (result string=w739:string)  [unwired: 6 in, 3 out]
                        n660 = local read "MN"() -> (w734:string)
                        n661 = local read "PW"() -> (w733:string)
                        n662 = call "数据编码.vi"("table输入"="系统状态" ("新元素/子数组"), "QN"=w739, "MN"=w734, "PW"=w733) -> ("通讯包字符串"=w730:string)  [unwired: 10 in, 1 out]
                        n663 = local read "数据发送通道"() -> (w732:enum16{"TCP", "VISA"})
                        n664 = local write "发送报文显示"(w730) -> ()
                        n665 = call "VISATCP组合选择发送.vi"("数据发送通道"=w732, "命令"="write", "写入缓冲区"=w730) -> ("错误输出"=w729:errorcluster)  [unwired: 9 in, 3 out]
                        n666 = Build Array(w730) -> (w738:string[])
                        n667 = local write "错误输出"(w729) -> ()
                        n668 = call "发送数据记录到文档(子VI).vi"("数组"=w738) -> ()  [unwired: 9 in, 1 out]
                      }
                    }
                  }
                  frame True {
                  }
                }
              }
            }
          }
          frame "运行模式" {
            # "直接1分钟查询 一次,有变化就按上传,没变化就不上传"
            n669 = flat-sequence {
              frame #0 {
                # "时间"
                n670 = global write "全局 小时数据发送次数.vi" "小时数据发送次数"(0 ("小时数据发送次数")) -> ()
                n671 = global write "全局 数据数组大小.vi" "数据数组大小"(1 ("数据数组大小")) -> ()
                n672 = global write "全局1.vi" "枚举"(enum16{"返回请求应答", "上传数据", "返回执行结果"}."上传数据" ("枚举")) -> ()
              }
              frame #1 {
                # "判定是否存表"
                n673 = property on="TCP服务端掉线计数" class="DigNum (严格)"() -> ("Value"=w749:i32)  [unwired: 2 in, 2 out]
                n674 = Greater Or Equal?(x=w749, y=1) -> (x >= y?=w748:bool)
                n675 = case shown="假" w748 {
                  frame False {
                    n676 = global read "全局 数据数组大小.vi" "数据数组大小"() -> (w751:i32)
                    n677 = Greater Than 0?(x=w751) -> (x > 0?=w752:bool)
                    n678 = case shown="真" w752 {
                      frame False {
                      }
                      frame True {
                        n679 = global read "全局 小时数据发送次数.vi" "小时数据发送次数"() -> (w761:i32)
                        n680 = local write "核查数据上传"(TRUE ("数据上传")) -> ()
                        n681 = Get Date/Time In Seconds() -> (seconds since 1Jan1904=w766:timestamp)
                        n682 = Increment(x=w761) -> (x+1=w760:i32)
                        n683 = Format Date/Time String(time format string (%c)="%Y%m%d%H%M%S%3u" ("时间格式字符串(%c)"), seconds (now)=w766) -> (date/time string=w765:string)  [unwired: 1 in]
                        n684 = global write "全局 小时数据发送次数.vi" "小时数据发送次数"(w760) -> ()
                        n685 = Search and Replace String(input string=w765, search string="." ("搜索字符串")) -> (result string=w763:string)  [unwired: 6 in, 3 out]
                        n686 = local read "MN"() -> (w757:string)
                        n687 = local read "PW"() -> (w758:string)
                        n688 = local read "数据发送通道"() -> (w756:enum16{"TCP", "VISA"})
                        n689 = call "数据编码.vi"("table输入"="运行模式" ("新元素/子数组"), "QN"=w763, "MN"=w757, "PW"=w758) -> ("通讯包字符串"=w753:string)  [unwired: 10 in, 1 out]
                        n690 = local write "发送报文显示"(w753) -> ()
                        n691 = call "VISATCP组合选择发送.vi"("数据发送通道"=w756, "命令"="write", "写入缓冲区"=w753) -> ("错误输出"=w754:errorcluster)  [unwired: 9 in, 3 out]
                        n692 = Build Array(w753) -> (w762:string[])
                        n693 = local write "错误输出"(w754) -> ()
                        n694 = call "发送数据记录到文档(子VI).vi"("数组"=w762) -> ()  [unwired: 9 in, 1 out]
                      }
                    }
                  }
                  frame True {
                  }
                }
              }
            }
          }
          frame "测量周期" {
            # "直接1分钟查询 一次,有变化就按上传,没变化就不上传"
            n695 = flat-sequence {
              frame #0 {
                # "时间"
                n696 = global write "全局 小时数据发送次数.vi" "小时数据发送次数"(0 ("小时数据发送次数")) -> ()
                n697 = global write "全局 数据数组大小.vi" "数据数组大小"(1 ("数据数组大小")) -> ()
                n698 = global write "全局1.vi" "枚举"(enum16{"返回请求应答", "上传数据", "返回执行结果"}."上传数据" ("枚举")) -> ()
              }
              frame #1 {
                # "判定是否存表"
                n699 = property on="TCP服务端掉线计数" class="DigNum (严格)"() -> ("Value"=w773:i32)  [unwired: 2 in, 2 out]
                n700 = Greater Or Equal?(x=w773, y=1) -> (x >= y?=w772:bool)
                n701 = case shown="假" w772 {
                  frame False {
                    n702 = global read "全局 数据数组大小.vi" "数据数组大小"() -> (w775:i32)
                    n703 = Greater Than 0?(x=w775) -> (x > 0?=w776:bool)
                    n704 = case shown="真" w776 {
                      frame False {
                      }
                      frame True {
                        n705 = global read "全局 小时数据发送次数.vi" "小时数据发送次数"() -> (w785:i32)
                        n706 = local write "核查数据上传"(TRUE ("数据上传")) -> ()
                        n707 = Get Date/Time In Seconds() -> (seconds since 1Jan1904=w790:timestamp)
                        n708 = Increment(x=w785) -> (x+1=w784:i32)
                        n709 = Format Date/Time String(time format string (%c)="%Y%m%d%H%M%S%3u" ("时间格式字符串(%c)"), seconds (now)=w790) -> (date/time string=w789:string)  [unwired: 1 in]
                        n710 = global write "全局 小时数据发送次数.vi" "小时数据发送次数"(w784) -> ()
                        n711 = Search and Replace String(input string=w789, search string="." ("搜索字符串")) -> (result string=w787:string)  [unwired: 6 in, 3 out]
                        n712 = local read "MN"() -> (w782:string)
                        n713 = local read "PW"() -> (w781:string)
                        n714 = call "数据编码.vi"("table输入"="测量周期" ("新元素/子数组"), "QN"=w787, "MN"=w782, "PW"=w781) -> ("通讯包字符串"=w778:string)  [unwired: 10 in, 1 out]
                        n715 = local read "数据发送通道"() -> (w780:enum16{"TCP", "VISA"})
                        n716 = local write "发送报文显示"(w778) -> ()
                        n717 = call "VISATCP组合选择发送.vi"("数据发送通道"=w780, "命令"="write", "写入缓冲区"=w778) -> ("错误输出"=w777:errorcluster)  [unwired: 9 in, 3 out]
                        n718 = Build Array(w778) -> (w786:string[])
                        n719 = local write "错误输出"(w777) -> ()
                        n720 = call "发送数据记录到文档(子VI).vi"("数组"=w786) -> ()  [unwired: 9 in, 1 out]
                      }
                    }
                  }
                  frame True {
                  }
                }
              }
            }
          }
          frame "超标留样" {
            # "直接1分钟查询 一次,有变化就按上传,没变化就不上传"
            n721 = flat-sequence {
              frame #0 {
                # "时间"
                n722 = global write "全局 小时数据发送次数.vi" "小时数据发送次数"(0 ("小时数据发送次数")) -> ()
                n723 = global write "全局 数据数组大小.vi" "数据数组大小"(1 ("数据数组大小")) -> ()
                n724 = global write "全局1.vi" "枚举"(enum16{"返回请求应答", "上传数据", "返回执行结果"}."上传数据" ("枚举")) -> ()
              }
              frame #1 {
                # "判定是否存表"
                n725 = property on="TCP服务端掉线计数" class="DigNum (严格)"() -> ("Value"=w797:i32)  [unwired: 2 in, 2 out]
                n726 = Greater Or Equal?(x=w797, y=1) -> (x >= y?=w796:bool)
                n727 = case shown="假" w796 {
                  frame False {
                    n728 = global read "全局 数据数组大小.vi" "数据数组大小"() -> (w799:i32)
                    n729 = Greater Than 0?(x=w799) -> (x > 0?=w800:bool)
                    n730 = case shown="真" w800 {
                      frame False {
                      }
                      frame True {
                        n731 = global read "全局 小时数据发送次数.vi" "小时数据发送次数"() -> (w809:i32)
                        n732 = local write "核查数据上传"(TRUE ("数据上传")) -> ()
                        n733 = Get Date/Time In Seconds() -> (seconds since 1Jan1904=w814:timestamp)
                        n734 = Increment(x=w809) -> (x+1=w808:i32)
                        n735 = Format Date/Time String(time format string (%c)="%Y%m%d%H%M%S%3u" ("时间格式字符串(%c)"), seconds (now)=w814) -> (date/time string=w813:string)  [unwired: 1 in]
                        n736 = global write "全局 小时数据发送次数.vi" "小时数据发送次数"(w808) -> ()
                        n737 = Search and Replace String(input string=w813, search string="." ("搜索字符串")) -> (result string=w811:string)  [unwired: 6 in, 3 out]
                        n738 = local read "MN"() -> (w806:string)
                        n739 = local read "PW"() -> (w805:string)
                        n740 = call "数据编码.vi"("table输入"="超标留样" ("新元素/子数组"), "QN"=w811, "MN"=w806, "PW"=w805) -> ("通讯包字符串"=w802:string)  [unwired: 10 in, 1 out]
                        n741 = local read "数据发送通道"() -> (w804:enum16{"TCP", "VISA"})
                        n742 = local write "发送报文显示"(w802) -> ()
                        n743 = call "VISATCP组合选择发送.vi"("数据发送通道"=w804, "命令"="write", "写入缓冲区"=w802) -> ("错误输出"=w801:errorcluster)  [unwired: 9 in, 3 out]
                        n744 = Build Array(w802) -> (w810:string[])
                        n745 = local write "错误输出"(w801) -> ()
                        n746 = call "发送数据记录到文档(子VI).vi"("数组"=w810) -> ()  [unwired: 9 in, 1 out]
                      }
                    }
                  }
                  frame True {
                  }
                }
              }
            }
          }
          frame "报警信息" {
            # "间隔时间上传"
            # "直接1分钟查询 一次,有数据就按数据上传,没数据为空的不传,在数据发送那边有做处理"
            n747 = flat-sequence {
              frame #0 {
                # "分钟时间间隔"
                n748 = global read "全局 数据发送重叠.vi" "数据发送重叠开始时间戳"() -> (w818:string)
                n749 = global read "全局 数据发送重叠.vi" "数据发送重叠"() -> (w817:bool)
                n750 = global write "全局 小时数据发送次数.vi" "小时数据发送次数"(0 ("小时数据发送次数")) -> ()
                n751 = global write "全局1.vi" "枚举"(enum16{"返回请求应答", "上传数据", "返回执行结果"}."上传数据" ("枚举")) -> ()
                n752 = call "日志信息主动发送(子VI).vi"("是否正在查询数据"=w817, "查询数据发送时间节点"=w818) -> ()  [unwired: 10 in]
              }
              frame #1 {
                n753 = call "获取报警信息 (子VI).vi"() -> ()  [unwired: 12 in]
              }
              frame #2 {
                n754 = call "数据处理整合 (子VI).vi"("枚举"=enum16{"实时数据排序", "小时数据排序"}."实时数据排序") -> ("已排序的数组"=w823:string[])  [unwired: 10 in]
                n755 = Array Size(array=w823) -> (size(s)=w822:i32)
                n756 = global write "全局 数据数组大小.vi" "数据数组大小"(w822) -> ()
              }
              frame #3 {
                n757 = while {
                  stop <- w824 stop-if-true
                  # "判定是否存表"
                  n758 = property on="TCP服务端掉线计数" class="DigNum (严格)"() -> ("Value"=w830:i32)  [unwired: 2 in, 2 out]
                  n759 = Greater Or Equal?(x=w830, y=1) -> (x >= y?=w829:bool)
                  n760 = case shown="假" w829 {
                    frame False {
                      # "判定数据不为空才发"
                      n761 = global read "全局 数据数组大小.vi" "数据数组大小"() -> (w832:i32)
                      n762 = Greater Than 0?(x=w832) -> (x > 0?=w833:bool)
                      n763 = case shown="真" w833 {
                        frame False {
                          n764 = local write "核查数据上传"(FALSE ("数据上传")) -> ()
                        }
                        frame True {
                          n765 = global read "全局 小时数据发送次数.vi" "小时数据发送次数"() -> (w842:i32)
                          n766 = Get Date/Time In Seconds() -> (seconds since 1Jan1904=w847:timestamp)
                          n767 = Increment(x=w842) -> (x+1=w841:i32)
                          n768 = Format Date/Time String(time format string (%c)="%Y%m%d%H%M%S%3u" ("时间格式字符串(%c)"), seconds (now)=w847) -> (date/time string=w846:string)  [unwired: 1 in]
                          n769 = global write "全局 小时数据发送次数.vi" "小时数据发送次数"(w841) -> ()
                          n770 = Search and Replace String(input string=w846, search string="." ("搜索字符串")) -> (result string=w844:string)  [unwired: 6 in, 3 out]
                          n771 = local read "MN"() -> (w840:string)
                          n772 = local read "PW"() -> (w839:string)
                          n773 = local read "数据发送通道"() -> (w838:enum16{"TCP", "VISA"})
                          n774 = call "数据编码.vi"("table输入"="报警信息" ("新元素/子数组"), "QN"=w844, "MN"=w840, "PW"=w839) -> ("通讯包字符串"=w836:string)  [unwired: 10 in, 1 out]
                          n775 = local write "发送报文显示"(w836) -> ()
                          n776 = Build Array(w836) -> (w843:string[])
                          n777 = call "VISATCP组合选择发送.vi"("数据发送通道"=w838, "命令"="write", "写入缓冲区"=w836) -> ("错误输出"=w835:errorcluster)  [unwired: 9 in, 3 out]
                          n778 = local write "错误输出"(w835) -> ()
                          n779 = call "发送数据记录到文档(子VI).vi"("数组"=w843) -> ()  [unwired: 9 in, 1 out]
                        }
                      }
                    }
                    frame True {
                    }
                  }
                  n780 = Wait (ms)(milliseconds to wait=u32 500 ("等待时间（毫秒）")) -> ()  [unwired: 1 out]
                  n781 = global read "全局 数据数组大小.vi" "数据数组大小"() -> (w826:i32)
                  n782 = global read "全局 小时数据发送次数.vi" "小时数据发送次数"() -> (w828:i32)
                  n783 = Decrement(x=w826) -> (x-1=w825:i32)
                  n784 = Greater Or Equal?(x=w828, y=w825) -> (x >= y?=w824:bool)
                }
              }
            }
          }
          frame "环境参数" {
            # "间隔时间上传"
            # "直接1分钟查询 一次,有数据就按数据上传,没数据为空的不传,在数据发送那边有做处理"
            n785 = disable-structure shown="禁用" {
              frame Disabled {
                n786 = flat-sequence {
                  frame #0 {
                    # "分钟时间间隔"
                    n787 = global read "全局 数据发送重叠.vi" "数据发送重叠开始时间戳"() -> (w851:string)
                    n788 = global read "全局 数据发送重叠.vi" "数据发送重叠"() -> (w850:bool)
                    n789 = global write "全局 小时数据发送次数.vi" "小时数据发送次数"(0 ("小时数据发送次数")) -> ()
                    n790 = global write "全局1.vi" "枚举"(enum16{"返回请求应答", "上传数据", "返回执行结果"}."上传数据" ("枚举")) -> ()
                    n791 = call "日志信息主动发送(子VI).vi"("是否正在查询数据"=w850, "查询数据发送时间节点"=w851) -> ()  [unwired: 10 in]
                  }
                  frame #1 {
                    n792 = call "获取环境参数 (子VI).vi"() -> ()  [unwired: 12 in]
                  }
                  frame #2 {
                    n793 = call "数据处理整合 (子VI).vi"("枚举"=enum16{"实时数据排序", "小时数据排序"}."实时数据排序") -> ("已排序的数组"=w856:string[])  [unwired: 10 in]
                    n794 = Array Size(array=w856) -> (size(s)=w855:i32)
                    n795 = global write "全局 数据数组大小.vi" "数据数组大小"(w855) -> ()
                  }
                  frame #3 {
                    n796 = while {
                      stop <- w857 stop-if-true
                      # "判定是否存表"
                      n797 = property on="TCP服务端掉线计数" class="DigNum (严格)"() -> ("Value"=w863:i32)  [unwired: 2 in, 2 out]
                      n798 = Greater Or Equal?(x=w863, y=1) -> (x >= y?=w862:bool)
                      n799 = case shown="假" w862 {
                        frame False {
                          # "判定数据不为空才发"
                          n800 = global read "全局 数据数组大小.vi" "数据数组大小"() -> (w865:i32)
                          n801 = Greater Than 0?(x=w865) -> (x > 0?=w866:bool)
                          n802 = case shown="真" w866 {
                            frame False {
                            }
                            frame True {
                              n803 = global read "全局 小时数据发送次数.vi" "小时数据发送次数"() -> (w873:i32)
                              n804 = local write "核查数据上传"(TRUE ("数据上传")) -> ()
                              n805 = Get Date/Time In Seconds() -> (seconds since 1Jan1904=w878:timestamp)
                              n806 = Increment(x=w873) -> (x+1=w872:i32)
                              n807 = Format Date/Time String(time format string (%c)="%Y%m%d%H%M%S%3u" ("时间格式字符串(%c)"), seconds (now)=w878) -> (date/time string=w877:string)  [unwired: 1 in]
                              n808 = global write "全局 小时数据发送次数.vi" "小时数据发送次数"(w872) -> ()
                              n809 = Search and Replace String(input string=w877, search string="." ("搜索字符串")) -> (result string=w875:string)  [unwired: 6 in, 3 out]
                              n810 = local read "MN"() -> (w881:string)
                              n811 = local read "PW"() -> (w880:string)
                              n812 = local read "数据发送通道"() -> (w869:enum16{"TCP", "VISA"})
                              n813 = call "数据编码.vi"("table输入"="报警信息" ("新元素/子数组"), "QN"=w875, "MN"=w881, "PW"=w880) -> ("通讯包字符串"=w868:string)  [unwired: 10 in, 1 out]
                              n814 = local write "发送报文显示"(w868) -> ()
                              n815 = call "VISATCP组合选择发送.vi"("数据发送通道"=w869, "命令"="write", "写入缓冲区"=w868) -> ("错误输出"=w867:errorcluster)  [unwired: 9 in, 3 out]
                              n816 = Build Array(w868) -> (w874:string[])
                              n817 = local write "错误输出"(w867) -> ()
                              n818 = call "发送数据记录到文档(子VI).vi"("数组"=w874) -> ()  [unwired: 9 in, 1 out]
                            }
                          }
                        }
                        frame True {
                        }
                      }
                      n819 = Wait (ms)(milliseconds to wait=u32 500 ("等待时间（毫秒）")) -> ()  [unwired: 1 out]
                      n820 = global read "全局 数据数组大小.vi" "数据数组大小"() -> (w859:i32)
                      n821 = global read "全局 小时数据发送次数.vi" "小时数据发送次数"() -> (w861:i32)
                      n822 = Decrement(x=w859) -> (x-1=w858:i32)
                      n823 = Greater Or Equal?(x=w861, y=w858) -> (x >= y?=w857:bool)
                    }
                  }
                }
              }
              frame Enabled {
              }
            }
          }
        }
      }
    }
  }
  n824 = while {
    tunnel: w38 -> [w886]
    stop <- FALSE stop-if-true
    # "和工控机通讯系统状态改变主动上传"
    # "整点发送小时数据(禁用）运行模式运行周期"
    n825 = Multiply(x=u32 1, y=u32 1000 ("等待时间（毫秒）")) -> (x*y=w892:u32)
    n826 = case shown="真" "每周自动重发" {
      frame False {
      }
      frame True {
        (unwired) T1."00点"
        (unwired) T2."关闭"
        # "自动重发水样数据"
        n827 = Get Date/Time In Seconds() -> (seconds since 1Jan1904=w957:timestamp)
        n828 = Seconds To Date/Time(time stamp (now)=w957) -> (date time rec=w951:T9)  [unwired: 1 in]
        n829 = Unbundle By Name(w951) -> ("天数（周）"=w956:i32, "时"=w946:i32, "分"=w955:i32)
        n830 = Equal To 0?(x=w955) -> (x = 0?=w952:bool)
        n831 = Equal?(x=w956, y="重发日期") -> (x = y?=w954:bool)
        n832 = Equal?(x=w946, y="重发时间") -> (x = y?=w953:bool)
        n833 = Compound Arithmetic op=AND ("复合运算")(w954, w953, w952) -> (w950:bool)
        n834 = call <vilib>:"Boolean Crossing PtByPt.vi"("direction"=enum16{"either", "false-true", "true-false"}."false-true", "input"=w950) -> ("crossing"=w949:bool)  [unwired: 1 in]
        n835 = case shown="真" w949 {
          tunnel: w951 -> [_ w959]
          frame False {
          }
          frame True {
            n836 = local read "参数数值"() -> (w964:T5)
            n837 = Unbundle By Name(w959) -> ("日"=w962:i32)
            n838 = Cluster To Array(cluster=w964) -> (array=w965:bool[])
            n839 = Subtract(x=w962, y=7) -> (x-y=w960:i32)
            n840 = Bundle By Name(cluster=w959, "日"=w960) -> (w963:T9)
            n841 = Date/Time To Seconds(2:w963) -> (0:w958:timestamp)  [unwired: 1 in]
            n842 = for {
              tunnel: w965 -> [_] mode=indexing
              tunnel: w958 -> [w966]
              i -> [w967]
              n843 = Format Date/Time String(time format string (%c)="%Y/%m/%d %H:%M:%S" ("时间格式字符串(%c)"), seconds (now)=w966) -> (date/time string=w968:string)  [unwired: 1 in]
              n844 = case shown="16" w967 {
                tunnel: w968 -> [w970 w971 w972 w973 w974 w975 w976 w977 w978 w979 w980 w981 w982 w983 w984 w985 w986 w987]
                frame 0, Default {
                  n845 = global write "全局 水样时间.vi" "time1"(w970) -> ()
                }
                frame 1 {
                  n846 = global write "全局 水样时间.vi" "time2"(w971) -> ()
                }
                frame 2 {
                  n847 = global write "全局 水样时间.vi" "time3"(w972) -> ()
                }
                frame 3 {
                  n848 = global write "全局 水样时间.vi" "time4"(w973) -> ()
                }
                frame 4 {
                  n849 = global write "全局 水样时间.vi" "time5"(w974) -> ()
                }
                frame 5 {
                  n850 = global write "全局 水样时间.vi" "time6"(w975) -> ()
                }
                frame 6 {
                  n851 = global write "全局 水样时间.vi" "time7"(w976) -> ()
                }
                frame 7 {
                  n852 = global write "全局 水样时间.vi" "time8"(w977) -> ()
                }
                frame 8 {
                  n853 = global write "全局 水样时间.vi" "time9"(w978) -> ()
                }
                frame 9 {
                  n854 = global write "全局 水样时间.vi" "time10"(w979) -> ()
                }
                frame 10 {
                  n855 = global write "全局 水样时间.vi" "time11"(w980) -> ()
                }
                frame 11 {
                  n856 = global write "全局 水样时间.vi" "time12"(w981) -> ()
                }
                frame 12 {
                  n857 = global write "全局 水样时间.vi" "time13"(w982) -> ()
                }
                frame 13 {
                  n858 = global write "全局 水样时间.vi" "time14"(w983) -> ()
                }
                frame 14 {
                  n859 = global write "全局 水样时间.vi" "time15"(w984) -> ()
                }
                frame 15 {
                  n860 = global write "全局 水样时间.vi" "time16"(w985) -> ()
                }
                frame 16 {
                  n861 = global write "全局 水样时间.vi" "time17"(w986) -> ()
                }
                frame 17 {
                  n862 = global write "全局 水样时间.vi" "time18"(w987) -> ()
                }
              }
            }
          }
        }
      }
    }
    n863 = Wait (ms)(milliseconds to wait=w892) -> ()  [unwired: 1 out]
    n864 = First Call?() -> (First Call?: T/F=w883:bool)
    n865 = case shown="假" w883 {
      tunnel: ["读取" ("读取写入选择") "打开" ("读取写入选择")] -> w889
      frame False {
      }
      frame True {
      }
    }
    n866 = call "Modbus Master.vi"("Unit ID"=u8 1, "读取写入选择"=w889) -> ("register values"=w887:u16[], "error out"=w884:errorcluster)  [unwired: 8 in]
    n867 = case shown="无错误" w884 {
      tunnel: w887 -> [w898 _]
      tunnel: w886 -> [w896 _]
      frame No Error {
        # "防止由于MBtcp错误导致状态为0发送至平台"
        n868 = global read "全局1.vi" "register values"() -> (w897:u16[])
        n869 = flat-sequence {
          tunnel: w898 -> [w904]
          tunnel: w897 -> [w924]
          tunnel: w896 -> [w900]
          tunnel: [w904] -> w899
          tunnel: w899 -> [w944]
          frame #0 {
            n870 = Index Array(array=w904) -> (element #1=w911:u16, element #2=w923:u16, element #3=w922:u16, element #4=w921:u16, element #5=w920:u16, element #6=w919:u16, element #7=w909:u16, element #8=w903:u16)  [unwired: 8 in]
            n871 = Index Array(array=w924) -> (element #1=w910:u16, element #2=w918:u16, element #3=w917:u16, element #4=w916:u16, element #5=w915:u16, element #6=w914:u16, element #7=w908:u16, element #8=w902:u16)  [unwired: 8 in]
            n872 = Build Array(w923, w922, w921, w920, w919) -> (w913:u16[])
            n873 = Build Array(w918, w917, w916, w915, w914) -> (w912:u16[])
            n874 = Not Equal?(x=w911, y=w910) -> (x != y?=w906:bool)
            n875 = Not Equal?(x=w909, y=w908) -> (x != y?=w907:bool)
            n876 = Not Equal?(x=w903, y=w902) -> (x != y?=w901:bool)
            n877 = Not Equal?(x=w913, y=w912) -> (x != y?=w905:bool[])
            n878 = while {
              tunnel: w900 -> [w933]
              tunnel: w905 -> [w930] mode=indexing
              i -> [w932]
              stop <- w928 stop-if-true
              n879 = Greater Or Equal?(x=w932, y=4) -> (x >= y?=w929:bool)
              n880 = Or(x=w930, y=w929) -> (x .or. y?=w928:bool)
              n881 = case shown="真" w930 {
                tunnel: w933 -> [_ w935]
                frame False {
                }
                frame True {
                  n882 = local write "系统状态改变"(TRUE ("系统状态改变")) -> ()
                  n883 = Enqueue Element(queue=w935, element="系统状态" ("元素")) -> ()  [unwired: 2 in, 3 out]
                }
              }
            }
            n884 = case shown="真" w906 {
              tunnel: w900 -> [_ w941]
              frame False {
              }
              frame True {
                n885 = Enqueue Element(queue=w941, element="运行模式" ("元素")) -> ()  [unwired: 2 in, 3 out]
                "系统状态改变" <- TRUE
              }
            }
            n886 = case shown="真" w901 {
              tunnel: w900 -> [_ w926]
              frame False {
              }
              frame True {
                n887 = local write "系统状态改变"(TRUE ("系统状态改变")) -> ()
                n888 = Enqueue Element(queue=w926, element="超标留样" ("元素")) -> ()  [unwired: 2 in, 3 out]
              }
            }
            n889 = case shown="真" w907 {
              tunnel: w900 -> [_ w938]
              frame False {
              }
              frame True {
                n890 = local write "系统状态改变"(TRUE ("系统状态改变")) -> ()
                n891 = Enqueue Element(queue=w938, element="测量周期" ("元素")) -> ()  [unwired: 2 in, 3 out]
              }
            }
          }
          frame #1 {
            n892 = global write "全局1.vi" "register values"(w944) -> ()
            n893 = local write "系统状态改变"(FALSE ("系统状态改变")) -> ()
          }
        }
      }
      frame Error {
      }
    }
  }
  n894 = while "While循环" {
    tunnel: [w1004] -> _
    tunnel: w32 -> [w998]
    stop <- FALSE stop-if-true
    w988 = FALSE ("小时数据上传")
    # "实时、小时数据出数据就上传"
    n895 = property on="TCP服务端掉线计数" class="DigNum (严格)"() -> ("Value"=w1001:i32)  [unwired: 2 in, 2 out]
    n896 = local read "查询数据发送"() -> (w993:bool)
    n897 = local read "核查数据上传"() -> (w992:bool)
    n898 = local read "重发数据"() -> (w994:bool)
    n899 = local read "步骤"() -> (w1003:T6)
    n900 = local write "实时小时数据上传"(w988) -> ()
    n901 = global write "全局 数据发送重叠.vi" "主动上报数据中"(w988) -> ()
    n902 = Greater Or Equal?(x=w998, y=17) -> (x >= y?=w997:bool)
    n903 = Equal To 0?(x=w1001) -> (x = 0?=w999:bool)
    n904 = Not(x=w994) -> (.not. x?=w991:bool)
    n905 = Not(x=w993) -> (.not. x?=w990:bool)
    n906 = Not(x=w992) -> (.not. x?=w989:bool)
    n907 = Equal?(x=w1003, y=T6."读取数据" ("步骤")) -> (x = y?=w1000:bool)
    n908 = Wait (ms)(milliseconds to wait=u32 75430 ("等待时间（毫秒）")) -> ()  [unwired: 1 out]
    n909 = Compound Arithmetic op=AND ("复合运算")(w1000, w999, w997, w991, w990, w989) -> (w995:bool)
    n910 = case shown="真" w995 {
      tunnel: [_ w1009] -> w1004
      frame False {
        w1007 = FALSE ("小时数据上传")
        n911 = local write "实时小时数据上传"(w1007) -> ()
        n912 = global write "全局 数据发送重叠.vi" "主动上报数据中"(w1007) -> ()
      }
      frame True {
        n913 = flat-sequence {
          tunnel: [w1018] -> w1008
          tunnel: [w1384] -> w1009
          tunnel: w1008 -> [w1384]
          frame #0 {
            w1010 = TRUE ("小时数据上传")
            n914 = disable-structure shown="启用" {
              frame Disabled {
                n915 = call "读取-删除文件.vi"() -> ("error out"=w1011:errorcluster, "文本"=w1012:string[])  [unwired: 10 in]
                n916 = for {
                  tunnel: w1012 -> [w1015] mode=indexing
                  tunnel: [w1014] -> _ mode=indexing
                  tunnel: w1011 -> [w1013]
                  n917 = local read item#-1() -> (w1016)
                  n918 = call "数据补发判定有限循环.vi"("错误输入（无错误）"=w1013, "数据输入"=w1015, 10:w1016) -> ("error out"=w1014:errorcluster)  [unwired: 8 in]
                }
              }
              frame Enabled {
              }
            }
            n919 = global write "全局 数据发送重叠.vi" "主动上报数据中"(w1010) -> ()
            "实时小时数据上传" <- w1010
          }
          frame #1 {
            n920 = local read "数据发送协议"() -> (w1017:enum16{"2005-212协议", "2017-212协议"})
            n921 = case shown="\"2017-212协议\", 默认" w1017 {
              tunnel: [_ w1154] -> w1018
              frame "2005-212协议" {
                n922 = local read "参数数值"() -> (w1022:T5)
                n923 = Cluster To Array(cluster=w1022) -> (array=w1021:bool[])
                n924 = for {
                  tunnel: w1021 -> [_] mode=indexing
                  tunnel: [w1066] -> w1020
                  i -> [w1060]
                  w1061 = "1904/01/01 00:00:00"
                  (unwired) " where 时间 between #"
                  w1064 = "database1.mdb" ("database")
                  (unwired) "'and 数据类型 ='N' and 时间 between "
                  w1068 = 0 ("索引 (行)")
                  n925 = case shown="12" w1060 {
                    tunnel: [w1118 w1120 w1122 w1124 w1126 w1128 w1130 w1132 w1134 w1136 w1138 w1140 w1142 w1144 w1146 w1148 w1150 w1152] -> w1063
                    frame 0, Default {
                      n926 = control-ref of="CODMn"() -> (w1119:refnum<vi>)
                      n927 = property class="Bool (严格)"(reference=w1119) -> ("Label.Text"=w1118:string)  [unwired: 1 in, 2 out]
                    }
                    frame 1 {
                      n928 = control-ref of="CODCr"() -> (w1121:refnum<vi>)
                      n929 = property class="Bool (严格)"(reference=w1121) -> ("Label.Text"=w1120:string)  [unwired: 1 in, 2 out]
                    }
                    frame 2 {
                      n930 = control-ref of="DO"() -> (w1123:refnum<vi>)
                      n931 = property class="Bool (严格)"(reference=w1123) -> ("Label.Text"=w1122:string)  [unwired: 1 in, 2 out]
                    }
                    frame 3 {
                      n932 = control-ref of="铜"() -> (w1125:refnum<vi>)
                      n933 = property class="Bool (严格)"(reference=w1125) -> ("Label.Text"=w1124:string)  [unwired: 1 in, 2 out]
                    }
                    frame 4 {
                      n934 = control-ref of="PH"() -> (w1127:refnum<vi>)
                      n935 = property class="Bool (严格)"(reference=w1127) -> ("Label.Text"=w1126:string)  [unwired: 1 in, 2 out]
                    }
                    frame 5 {
                      n936 = control-ref of="氨氮"() -> (w1129:refnum<vi>)
                      n937 = property class="Bool (严格)"(reference=w1129) -> ("Label.Text"=w1128:string)  [unwired: 1 in, 2 out]
                    }
                    frame 6 {
                      n938 = control-ref of="比电导率"() -> (w1131:refnum<vi>)
                      n939 = property class="Bool (严格)"(reference=w1131) -> ("Label.Text"=w1130:string)  [unwired: 1 in, 2 out]
                    }
                    frame 7 {
                      n940 = control-ref of="水温"() -> (w1133:refnum<vi>)
                      n941 = property class="Bool (严格)"(reference=w1133) -> ("Label.Text"=w1132:string)  [unwired: 1 in, 2 out]
                    }
                    frame 8 {
                      n942 = control-ref of="盐度(海水)"() -> (w1135:refnum<vi>)
                      n943 = property class="Bool (严格)"(reference=w1135) -> ("Label.Text"=w1134:string)  [unwired: 1 in, 2 out]
                    }
                    frame 9 {
                      n944 = control-ref of="浊度"() -> (w1137:refnum<vi>)
                      n945 = property class="Bool (严格)"(reference=w1137) -> ("Label.Text"=w1136:string)  [unwired: 1 in, 2 out]
                    }
                    frame 10 {
                      n946 = control-ref of="总氮"() -> (w1139:refnum<vi>)
                      n947 = property class="Bool (严格)"(reference=w1139) -> ("Label.Text"=w1138:string)  [unwired: 1 in, 2 out]
                    }
                    frame 11 {
                      n948 = control-ref of="总磷"() -> (w1141:refnum<vi>)
                      n949 = property class="Bool (严格)"(reference=w1141) -> ("Label.Text"=w1140:string)  [unwired: 1 in, 2 out]
                    }
                    frame 12 {
                      n950 = control-ref of="叶绿素a"() -> (w1143:refnum<vi>)
                      n951 = property class="Bool (严格)"(reference=w1143) -> ("Label.Text"=w1142:string)  [unwired: 1 in, 2 out]
                    }
                    frame 13 {
                      n952 = control-ref of="藻密度"() -> (w1145:refnum<vi>)
                      n953 = property class="Bool (严格)"(reference=w1145) -> ("Label.Text"=w1144:string)  [unwired: 1 in, 2 out]
                    }
                    frame 14 {
                      n954 = control-ref of="水位"() -> (w1147:refnum<vi>)
                      n955 = property class="Bool (严格)"(reference=w1147) -> ("Label.Text"=w1146:string)  [unwired: 1 in, 2 out]
                    }
                    frame 15 {
                      n956 = control-ref of="流速"() -> (w1149:refnum<vi>)
                      n957 = property class="Bool (严格)"(reference=w1149) -> ("Label.Text"=w1148:string)  [unwired: 1 in, 2 out]
                    }
                    frame 16 {
                      n958 = control-ref of="瞬时流量"() -> (w1151:refnum<vi>)
                      n959 = property class="Bool (严格)"(reference=w1151) -> ("Label.Text"=w1150:string)  [unwired: 1 in, 2 out]
                    }
                    frame 17 {
                      n960 = control-ref of="累积流量"() -> (w1153:refnum<vi>)
                      n961 = property class="Bool (严格)"(reference=w1153) -> ("Label.Text"=w1152:string)  [unwired: 1 in, 2 out]
                    }
                  }
                  n962 = Get Date/Time In Seconds() -> (seconds since 1Jan1904=w1072:timestamp)
                  n963 = Format Date/Time String(time format string (%c)="%Y/%m/%d %H:%M:%S" ("时间格式字符串(%c)"), seconds (now)=w1072) -> (date/time string=w1062:string)  [unwired: 1 in]
                  n964 = Format Into String(format string="#%s#" ("初始字符串"), w1061) -> (resulting string=w1070:string)  [unwired: 2 in, 1 out]
                  n965 = Format Into String(format string="#%s#" ("初始字符串"), w1062) -> (resulting string=w1065:string)  [unwired: 2 in, 1 out]
                  n966 = case shown="0, 默认" w1060 {
                    selector: w1060 -> [_ w1104]
                    tunnel: w1070 -> [w1099 w1109]
                    tunnel: [w1098 w1110] -> w1069
                    tunnel: w1065 -> [w1095 w1108]
                    tunnel: w1064 -> [_ w1107]
                    tunnel: w1063 -> [_ w1106]
                    tunnel: w1061 -> [_ w1101]
                    tunnel: w1062 -> [_ w1103]
                    frame 0, Default {
                      n967 = Concatenate Strings("where 测量模式 ='水样测试" ("condition"), "'and 时间 between ", w1099, "and" ("字符串"), w1095, " order by 时间 desc" ("字符串")) -> (w1098:string)
                    }
                    frame 14..17 {
                      n968 = call "流量数据规范小时时间戳.vi"("字符串"=w1101) -> ("result string"=w1100:string)  [unwired: 10 in]
                      n969 = call "database1查询.vi"("时间2"=w1103, "table"=w1106, "时间1"=w1100, "database"=w1107) -> ("error out"=w1102:errorcluster, "data"=w1105:string[][])  [unwired: 4 in, 1 out]
                      n970 = call <vilib>:"Clear Errors.vi"("error in (no error)"=w1102) -> ()  [unwired: 5 in, 2 out]
                      n971 = case shown="14" w1104 {
                        tunnel: w1105 -> [_ w1114 w1115 w1116 w1117]
                        frame 0, Default {
                        }
                        frame 14 {
                          n972 = global write "全局流量数据小时.vi" "水位"(w1114) -> ()
                        }
                        frame 15 {
                          n973 = global write "全局流量数据小时.vi" "流速"(w1115) -> ()
                        }
                        frame 16 {
                          n974 = global write "全局流量数据小时.vi" "瞬时流量"(w1116) -> ()
                        }
                        frame 17 {
                          n975 = global write "全局流量数据小时.vi" "累积流量"(w1117) -> ()
                        }
                      }
                      n976 = Concatenate Strings(" where 时间 between ", w1109, "and" ("字符串"), w1108, " order by 时间 desc" ("字符串")) -> (w1110:string)
                    }
                  }
                  n977 = call "SQL查询.vi"("condition"=w1069, "table输入"=w1063, "database"=w1064) -> ("error out"=w1066:errorcluster, "data"=w1059:string[][])  [unwired: 7 in]
                  n978 = call "短日期时间转长日期格式.vi"("data"=w1059) -> ("输出数组"=w1067:string[][])  [unwired: 10 in]
                  n979 = case shown="3" w1060 {
                    tunnel: w1059 -> [w1075 w1076 w1077 w1078 w1079 w1080 w1081 w1082 w1083 w1084 w1085 w1086 w1087 w1088 w1089 w1090 w1091 w1092]
                    frame 0, Default {
                      n980 = global write "全局 所有参数.vi" "CODMn"(w1075) -> ()
                    }
                    frame 1 {
                      n981 = global write "全局 所有参数.vi" "CODCr"(w1076) -> ()
                    }
                    frame 2 {
                      n982 = global write "全局 所有参数.vi" "DO"(w1077) -> ()
                    }
                    frame 3 {
                      n983 = global write "全局 所有参数.vi" "铜"(w1078) -> ()
                    }
                    frame 4 {
                      n984 = global write "全局 所有参数.vi" "PH"(w1079) -> ()
                    }
                    frame 5 {
                      n985 = global write "全局 所有参数.vi" "氨氮"(w1080) -> ()
                    }
                    frame 6 {
                      n986 = global write "全局 所有参数.vi" "电导率"(w1081) -> ()
                    }
                    frame 7 {
                      n987 = global write "全局 所有参数.vi" "水温"(w1082) -> ()
                    }
                    frame 8 {
                      n988 = global write "全局 所有参数.vi" "盐度"(w1083) -> ()
                    }
                    frame 9 {
                      n989 = global write "全局 所有参数.vi" "浊度"(w1084) -> ()
                    }
                    frame 10 {
                      n990 = global write "全局 所有参数.vi" "总氮"(w1085) -> ()
                    }
                    frame 11 {
                      n991 = global write "全局 所有参数.vi" "总磷"(w1086) -> ()
                    }
                    frame 12 {
                      n992 = global write "全局 所有参数.vi" "叶绿素"(w1087) -> ()
                    }
                    frame 13 {
                      n993 = global write "全局 所有参数.vi" "藻密度"(w1088) -> ()
                    }
                    frame 14 {
                      n994 = global write "全局 所有参数.vi" "水位"(w1089) -> ()
                    }
                    frame 15 {
                      n995 = global write "全局 所有参数.vi" "流速"(w1090) -> ()
                    }
                    frame 16 {
                      n996 = global write "全局 所有参数.vi" "瞬时流量"(w1091) -> ()
                    }
                    frame 17 {
                      n997 = global write "全局 所有参数.vi" "累积流量"(w1092) -> ()
                    }
                  }
                  n998 = Index Array(array=w1067, index (row)=w1068, index (col)=w1068) -> ()  [unwired: 1 out]
                }
                n999 = flat-sequence {
                  tunnel: w1020 -> [w1023]
                  tunnel: [w1023] -> w1019
                  tunnel: w1019 -> [w1029]
                  tunnel: [w1028] -> _
                  frame #0 {
                    n1000 = global write "全局 小时数据发送次数.vi" "小时数据发送次数"(0 ("小时数据发送次数")) -> ()
                    n1001 = call "数据处理直接插入整合 (子VI).vi"() -> ()  [unwired: 12 in]
                    n1002 = global write "全局1.vi" "枚举"(enum16{"返回请求应答", "上传数据", "返回执行结果"}."上传数据" ("枚举")) -> ()
                    n1003 = global write "全局 实时数据参数.vi" "实时数据参数"("水样测试" ("实时数据参数")) -> ()
                    n1004 = global write "全局 水样时间.vi" "选择发送的参数"("氨氮" ("选择发送的参数")) -> ()
                  }
                  frame #1 {
                    # "实时数据的大小"
                    n1005 = flat-sequence {
                      tunnel: [w1035] -> w1032
                      tunnel: [w1034] -> w1030
                      tunnel: w1029 -> [w1033]
                      tunnel: w1032 -> [_]
                      tunnel: [w1048] -> w1031
                      tunnel: w1030 -> [w1048]
                      tunnel: w1031 -> [w1056]
                      tunnel: [w1050] -> w1028
                      frame #0 {
                        n1006 = Get Date/Time In Seconds() -> (seconds since 1Jan1904=w1043:timestamp)
                        n1007 = Format Date/Time String(time format string (%c)="%Y%m%d%H%M%S%3u" ("时间格式字符串(%c)"), seconds (now)=w1043) -> (date/time string=w1044:string)  [unwired: 1 in]
                        n1008 = Search and Replace String(input string=w1044, search string="." ("搜索字符串")) -> (result string=w1046:string)  [unwired: 6 in, 3 out]
                        n1009 = local read "MN"() -> (w1039:string)
                        n1010 = local read "PW"() -> (w1038:string)
                        n1011 = local read "数据发送通道"() -> (w1037:enum16{"TCP", "VISA"})
                        n1012 = call "数据编码.vi"("table输入"="小时数据" ("新元素/子数组"), "QN"=w1046, "MN"=w1039, "PW"=w1038) -> ("通讯包字符串"=w1035:string)  [unwired: 10 in, 1 out]
                        n1013 = Build Array(w1035) -> (w1040:string[])
                        n1014 = local write "发送报文显示"(w1035) -> ()
                        n1015 = call "VISATCP组合选择发送.vi"("数据发送通道"=w1037, "命令"="write", "写入缓冲区"=w1035) -> ()  [unwired: 9 in, 4 out]
                        n1016 = call "发送数据记录到文档(子VI).vi"("错误输入"=w1033, "数组"=w1040) -> ("错误输出"=w1034:errorcluster)  [unwired: 8 in]
                      }
                      frame #1 {
                        n1017 = global write "全局 小时数据发送次数.vi" "小时数据发送次数"(0 ("小时数据发送次数")) -> ()
                        n1018 = Wait (ms)(milliseconds to wait=u32 500 ("等待时间（毫秒）")) -> ()  [unwired: 1 out]
                      }
                      frame #2 {
                        n1019 = local read "MN"() -> (w1055:string)
                        n1020 = local read "PW"() -> (w1054:string)
                        n1021 = call "数据编码.vi"("table输入"="实时数据" ("新元素/子数组"), "错误常量 2"=w1056, "MN"=w1055, "PW"=w1054) -> ("通讯包字符串"=w1051:string)  [unwired: 10 in, 1 out]
                        n1022 = Build Array(w1051) -> (w1058:string[])
                        n1023 = local read "数据发送通道"() -> (w1053:enum16{"TCP", "VISA"})
                        n1024 = local write "发送报文显示"(w1051) -> ()
                        n1025 = call "发送数据记录到文档(子VI).vi"("数组"=w1058) -> ()  [unwired: 9 in, 1 out]
                        n1026 = call "VISATCP组合选择发送.vi"("数据发送通道"=w1053, "命令"="write", "写入缓冲区"=w1051) -> ("错误输出"=w1050:errorcluster)  [unwired: 9 in, 3 out]
                      }
                    }
                  }
                }
              }
              frame "2017-212协议", Default {
                n1027 = local read "参数数值"() -> (w1156:T5)
                n1028 = Cluster To Array(cluster=w1156) -> (array=w1155:bool[])
                n1029 = for {
                  tunnel: w1155 -> [_] mode=indexing
                  tunnel: [w1163] -> w1154 mode=indexing
                  tunnel: [w1163] -> _
                  i -> [w1161]
                  (unwired) " where 时间 between #"
                  w1160 = "database1.mdb" ("database")
                  (unwired) "'and 数据类型 ='N' and 时间 between "
                  w1177 = 0 ("索引 (行)")
                  n1030 = case shown="3" w1161 {
                    tunnel: [w1347 w1349 w1351 w1353 w1355 w1357 w1359 w1361 w1363 w1365 w1367 w1369 w1371 w1373 w1375 w1377 w1379 w1381] -> w1159
                    frame 0, Default {
                      n1031 = control-ref of="CODMn"() -> (w1348:refnum<vi>)
                      n1032 = property class="Bool (严格)"(reference=w1348) -> ("Label.Text"=w1347:string)  [unwired: 1 in, 2 out]
                    }
                    frame 1 {
                      n1033 = control-ref of="CODCr"() -> (w1350:refnum<vi>)
                      n1034 = property class="Bool (严格)"(reference=w1350) -> ("Label.Text"=w1349:string)  [unwired: 1 in, 2 out]
                    }
                    frame 2 {
                      n1035 = control-ref of="DO"() -> (w1352:refnum<vi>)
                      n1036 = property class="Bool (严格)"(reference=w1352) -> ("Label.Text"=w1351:string)  [unwired: 1 in, 2 out]
                    }
                    frame 3 {
                      n1037 = control-ref of="铜"() -> (w1354:refnum<vi>)
                      n1038 = property class="Bool (严格)"(reference=w1354) -> ("Label.Text"=w1353:string)  [unwired: 1 in, 2 out]
                    }
                    frame 4 {
                      n1039 = control-ref of="PH"() -> (w1356:refnum<vi>)
                      n1040 = property class="Bool (严格)"(reference=w1356) -> ("Label.Text"=w1355:string)  [unwired: 1 in, 2 out]
                    }
                    frame 5 {
                      n1041 = control-ref of="氨氮"() -> (w1358:refnum<vi>)
                      n1042 = property class="Bool (严格)"(reference=w1358) -> ("Label.Text"=w1357:string)  [unwired: 1 in, 2 out]
                    }
                    frame 6 {
                      n1043 = control-ref of="比电导率"() -> (w1360:refnum<vi>)
                      n1044 = property class="Bool (严格)"(reference=w1360) -> ("Label.Text"=w1359:string)  [unwired: 1 in, 2 out]
                    }
                    frame 7 {
                      n1045 = control-ref of="水温"() -> (w1362:refnum<vi>)
                      n1046 = property class="Bool (严格)"(reference=w1362) -> ("Label.Text"=w1361:string)  [unwired: 1 in, 2 out]
                    }
                    frame 8 {
                      n1047 = control-ref of="盐度(海水)"() -> (w1364:refnum<vi>)
                      n1048 = property class="Bool (严格)"(reference=w1364) -> ("Label.Text"=w1363:string)  [unwired: 1 in, 2 out]
                    }
                    frame 9 {
                      n1049 = control-ref of="浊度"() -> (w1366:refnum<vi>)
                      n1050 = property class="Bool (严格)"(reference=w1366) -> ("Label.Text"=w1365:string)  [unwired: 1 in, 2 out]
                    }
                    frame 10 {
                      n1051 = control-ref of="总氮"() -> (w1368:refnum<vi>)
                      n1052 = property class="Bool (严格)"(reference=w1368) -> ("Label.Text"=w1367:string)  [unwired: 1 in, 2 out]
                    }
                    frame 11 {
                      n1053 = control-ref of="总磷"() -> (w1370:refnum<vi>)
                      n1054 = property class="Bool (严格)"(reference=w1370) -> ("Label.Text"=w1369:string)  [unwired: 1 in, 2 out]
                    }
                    frame 12 {
                      n1055 = control-ref of="叶绿素a"() -> (w1372:refnum<vi>)
                      n1056 = property class="Bool (严格)"(reference=w1372) -> ("Label.Text"=w1371:string)  [unwired: 1 in, 2 out]
                    }
                    frame 13 {
                      n1057 = control-ref of="藻密度"() -> (w1374:refnum<vi>)
                      n1058 = property class="Bool (严格)"(reference=w1374) -> ("Label.Text"=w1373:string)  [unwired: 1 in, 2 out]
                    }
                    frame 14 {
                      n1059 = control-ref of="水位"() -> (w1376:refnum<vi>)
                      n1060 = property class="Bool (严格)"(reference=w1376) -> ("Label.Text"=w1375:string)  [unwired: 1 in, 2 out]
                    }
                    frame 15 {
                      n1061 = control-ref of="流速"() -> (w1378:refnum<vi>)
                      n1062 = property class="Bool (严格)"(reference=w1378) -> ("Label.Text"=w1377:string)  [unwired: 1 in, 2 out]
                    }
                    frame 16 {
                      n1063 = control-ref of="瞬时流量"() -> (w1380:refnum<vi>)
                      n1064 = property class="Bool (严格)"(reference=w1380) -> ("Label.Text"=w1379:string)  [unwired: 1 in, 2 out]
                    }
                    frame 17 {
                      n1065 = control-ref of="累积流量"() -> (w1382:refnum<vi>)
                      n1066 = property class="Bool (严格)"(reference=w1382) -> ("Label.Text"=w1381:string)  [unwired: 1 in, 2 out]
                    }
                  }
                  n1067 = case shown="12" w1161 {
                    tunnel: [w1329 w1330 w1331 w1332 w1333 w1334 w1335 w1336 w1337 w1338 w1339 w1340 w1341 w1342 w1343 w1344 w1345 w1346] -> w1158
                    frame 0, Default {
                      n1068 = global read "全局 水样时间.vi" "time1"() -> (w1329:string)
                    }
                    frame 1 {
                      n1069 = global read "全局 水样时间.vi" "time2"() -> (w1330:string)
                    }
                    frame 2 {
                      n1070 = global read "全局 水样时间.vi" "time3"() -> (w1331:string)
                    }
                    frame 3 {
                      n1071 = global read "全局 水样时间.vi" "time4"() -> (w1332:string)
                    }
                    frame 4 {
                      n1072 = global read "全局 水样时间.vi" "time5"() -> (w1333:string)
                    }
                    frame 5 {
                      n1073 = global read "全局 水样时间.vi" "time6"() -> (w1334:string)
                    }
                    frame 6 {
                      n1074 = global read "全局 水样时间.vi" "time7"() -> (w1335:string)
                    }
                    frame 7 {
                      n1075 = global read "全局 水样时间.vi" "time8"() -> (w1336:string)
                    }
                    frame 8 {
                      n1076 = global read "全局 水样时间.vi" "time9"() -> (w1337:string)
                    }
                    frame 9 {
                      n1077 = global read "全局 水样时间.vi" "time10"() -> (w1338:string)
                    }
                    frame 10 {
                      n1078 = global read "全局 水样时间.vi" "time11"() -> (w1339:string)
                    }
                    frame 11 {
                      n1079 = global read "全局 水样时间.vi" "time12"() -> (w1340:string)
                    }
                    frame 12 {
                      n1080 = global read "全局 水样时间.vi" "time13"() -> (w1341:string)
                    }
                    frame 13 {
                      n1081 = global read "全局 水样时间.vi" "time14"() -> (w1342:string)
                    }
                    frame 14 {
                      n1082 = global read "全局 水样时间.vi" "time15"() -> (w1343:string)
                    }
                    frame 15 {
                      n1083 = global read "全局 水样时间.vi" "time16"() -> (w1344:string)
                    }
                    frame 16 {
                      n1084 = global read "全局 水样时间.vi" "time17"() -> (w1345:string)
                    }
                    frame 17 {
                      n1085 = global read "全局 水样时间.vi" "time18"() -> (w1346:string)
                    }
                  }
                  n1086 = Get Date/Time In Seconds() -> (seconds since 1Jan1904=w1182:timestamp)
                  n1087 = Format Date/Time String(time format string (%c)="%Y/%m/%d %H:%M:%S" ("时间格式字符串(%c)"), seconds (now)=w1182) -> (date/time string=w1157:string)  [unwired: 1 in]
                  n1088 = Format Into String(format string="#%s#" ("初始字符串"), w1158) -> (resulting string=w1180:string)  [unwired: 2 in, 1 out]
                  n1089 = Format Into String(format string="#%s#" ("初始字符串"), w1157) -> (resulting string=w1162:string)  [unwired: 2 in, 1 out]
                  n1090 = case shown="0, 默认" w1161 {
                    selector: w1161 -> [_ w1196]
                    tunnel: w1180 -> [w1191 w1201]
                    tunnel: [w1190 w1202] -> w1179
                    tunnel: w1162 -> [w1187 w1200]
                    tunnel: w1160 -> [_ w1199]
                    tunnel: w1159 -> [_ w1198]
                    tunnel: w1158 -> [_ w1193]
                    tunnel: w1157 -> [_ w1195]
                    frame 0, Default {
                      n1091 = Concatenate Strings("where 测量模式 ='水样测试" ("condition"), "'and 时间 between ", w1191, "and" ("字符串"), w1187, " order by 时间 desc" ("字符串")) -> (w1190:string)
                    }
                    frame 14..17 {
                      n1092 = call "流量数据规范小时时间戳.vi"("字符串"=w1193) -> ("result string"=w1192:string)  [unwired: 10 in]
                      n1093 = call "database1查询.vi"("时间2"=w1195, "table"=w1198, "时间1"=w1192, "database"=w1199) -> ("error out"=w1194:errorcluster, "data"=w1197:string[][])  [unwired: 4 in, 1 out]
                      n1094 = call <vilib>:"Clear Errors.vi"("error in (no error)"=w1194) -> ()  [unwired: 5 in, 2 out]
                      n1095 = case shown="14" w1196 {
                        tunnel: w1197 -> [_ w1206 w1207 w1208 w1209]
                        frame 0, Default {
                        }
                        frame 14 {
                          n1096 = global write "全局流量数据小时.vi" "水位"(w1206) -> ()
                        }
                        frame 15 {
                          n1097 = global write "全局流量数据小时.vi" "流速"(w1207) -> ()
                        }
                        frame 16 {
                          n1098 = global write "全局流量数据小时.vi" "瞬时流量"(w1208) -> ()
                        }
                        frame 17 {
                          n1099 = global write "全局流量数据小时.vi" "累积流量"(w1209) -> ()
                        }
                      }
                      n1100 = Concatenate Strings(" where 时间 between ", w1201, "and" ("字符串"), w1200, " order by 时间 desc" ("字符串")) -> (w1202:string)
                    }
                  }
                  n1101 = call "SQL查询.vi"("condition"=w1179, "table输入"=w1159, "database"=w1160) -> ("error out"=w1163:errorcluster, "data"=w1175:string[][])  [unwired: 7 in]
                  n1102 = Empty Array?(array=w1175) -> (empty?=w1178:bool)
                  n1103 = call "短日期时间转长日期格式.vi"("data"=w1175) -> ("输出数组"=w1176:string[][])  [unwired: 10 in]
                  n1104 = Not(x=w1178) -> (.not. x?=w1172:bool)
                  n1105 = Index Array(array=w1176, index (row)=w1177, index (col)=w1177) -> (element=w1169:string)
                  n1106 = global write "全局 水样时间.vi" "选择发送的参数"(w1159) -> ()
                  n1107 = flat-sequence {
                    tunnel: [w1217] -> w1174
                    tunnel: [w1216] -> w1173
                    tunnel: w1172 -> [w1217]
                    tunnel: w1175 -> [w1216]
                    tunnel: w1161 -> [w1211]
                    tunnel: w1159 -> [w1213]
                    tunnel: [w1213] -> w1170
                    tunnel: w1169 -> [w1212]
                    tunnel: [w1212] -> w1167
                    tunnel: [w1211] -> w1164
                    tunnel: w1174 -> [w1237]
                    tunnel: w1173 -> [w1240]
                    tunnel: [w1239] -> w1171
                    tunnel: w1170 -> [w1239]
                    tunnel: [w1238] -> w1168
                    tunnel: w1167 -> [w1238]
                    tunnel: [w1237] -> w1166
                    tunnel: [w1236] -> w1165
                    tunnel: w1164 -> [w1236]
                    tunnel: w1171 -> [w1297]
                    tunnel: w1168 -> [w1296]
                    tunnel: w1166 -> [w1294]
                    tunnel: w1165 -> [w1295]
                    frame #0 {
                      n1108 = case shown="3" w1211 {
                        tunnel: w1216 -> [w1218 w1219 w1220 w1221 w1222 w1223 w1224 w1225 w1226 w1227 w1228 w1229 w1230 w1231 w1232 w1233 w1234 w1235]
                        frame 0, Default {
                          n1109 = global write "全局 所有参数.vi" "CODMn"(w1218) -> ()
                        }
                        frame 1 {
                          n1110 = global write "全局 所有参数.vi" "CODCr"(w1219) -> ()
                        }
                        frame 2 {
                          n1111 = global write "全局 所有参数.vi" "DO"(w1220) -> ()
                        }
                        frame 3 {
                          n1112 = global write "全局 所有参数.vi" "铜"(w1221) -> ()
                        }
                        frame 4 {
                          n1113 = global write "全局 所有参数.vi" "PH"(w1222) -> ()
                        }
                        frame 5 {
                          n1114 = global write "全局 所有参数.vi" "氨氮"(w1223) -> ()
                        }
                        frame 6 {
                          n1115 = global write "全局 所有参数.vi" "电导率"(w1224) -> ()
                        }
                        frame 7 {
                          n1116 = global write "全局 所有参数.vi" "水温"(w1225) -> ()
                        }
                        frame 8 {
                          n1117 = global write "全局 所有参数.vi" "盐度"(w1226) -> ()
                        }
                        frame 9 {
                          n1118 = global write "全局 所有参数.vi" "浊度"(w1227) -> ()
                        }
                        frame 10 {
                          n1119 = global write "全局 所有参数.vi" "总氮"(w1228) -> ()
                        }
                        frame 11 {
                          n1120 = global write "全局 所有参数.vi" "总磷"(w1229) -> ()
                        }
                        frame 12 {
                          n1121 = global write "全局 所有参数.vi" "叶绿素"(w1230) -> ()
                        }
                        frame 13 {
                          n1122 = global write "全局 所有参数.vi" "藻密度"(w1231) -> ()
                        }
                        frame 14 {
                          n1123 = global write "全局 所有参数.vi" "水位"(w1232) -> ()
                        }
                        frame 15 {
                          n1124 = global write "全局 所有参数.vi" "流速"(w1233) -> ()
                        }
                        frame 16 {
                          n1125 = global write "全局 所有参数.vi" "瞬时流量"(w1234) -> ()
                        }
                        frame 17 {
                          n1126 = global write "全局 所有参数.vi" "累积流量"(w1235) -> ()
                        }
                      }
                      n1127 = global write "全局 小时数据发送次数.vi" "小时数据发送次数"(0 ("小时数据发送次数")) -> ()
                      n1128 = global write "全局 数据发送重叠.vi" "数据接收超时指示灯"(FALSE ("数据接收超时指示灯")) -> ()
                      n1129 = global write "全局1.vi" "枚举"(enum16{"返回请求应答", "上传数据", "返回执行结果"}."上传数据" ("枚举")) -> ()
                    }
                    frame #1 {
                      n1130 = case shown="真" w1237 {
                        tunnel: w1240 -> [_ w1243]
                        tunnel: w1236 -> [_ w1242]
                        tunnel: w1236 -> [_ w1241]
                        frame False {
                        }
                        frame True {
                          n1131 = for {
                            tunnel: w1243 -> [_] mode=indexing
                            tunnel: w1242 -> [w1261]
                            tunnel: w1241 -> [w1260]
                            # "实时数据的大小"
                            n1132 = Wait (ms)(milliseconds to wait=u32 500 ("等待时间（毫秒）")) -> ()  [unwired: 1 out]
                            n1133 = global write "全局 实时数据参数.vi" "实时数据参数"("水样测试" ("实时数据参数")) -> ()
                            n1134 = Get Date/Time In Seconds() -> (seconds since 1Jan1904=w1254:timestamp)
                            n1135 = Format Date/Time String(time format string (%c)="%Y%m%d%H%M%S%3u" ("时间格式字符串(%c)"), seconds (now)=w1254) -> (date/time string=w1255:string)  [unwired: 1 in]
                            n1136 = Search and Replace String(input string=w1255, search string="." ("搜索字符串")) -> (result string=w1257:string)  [unwired: 6 in, 3 out]
                            n1137 = local read "MN"() -> (w1249:string)
                            n1138 = local read "PW"() -> (w1248:string)
                            n1139 = local read "数据发送通道"() -> (w1247:enum16{"TCP", "VISA"})
                            n1140 = call "数据编码.vi"("table输入"="小时数据" ("新元素/子数组"), "QN"=w1257, "MN"=w1249, "PW"=w1248) -> ("通讯包字符串"=w1259:string)  [unwired: 10 in, 1 out]
                            n1141 = Build Array(w1259) -> (w1251:string[])
                            n1142 = local write "发送报文显示"(w1259) -> ()
                            n1143 = call "VISATCP组合选择发送.vi"("数据发送通道"=w1247, "命令"="write", "写入缓冲区"=w1259) -> ()  [unwired: 9 in, 4 out]
                            n1144 = call "发送数据记录到文档(子VI).vi"("数组"=w1251) -> ()  [unwired: 9 in, 1 out]
                            n1145 = local read "判断数据反馈"() -> (w1245:bool)
                            n1146 = case shown="真" w1245 {
                              tunnel: [_ w1284] -> w1258
                              tunnel: w1259 -> [_ w1283]
                              tunnel: w1261 -> [_ w1282]
                              frame False {
                              }
                              frame True {
                                n1147 = case shown="0, 默认" w1282 {
                                tunnel: [w1286 _] -> w1284
                                tunnel: w1283 -> [w1285 _]
                                frame 0, Default {
                                n1148 = Empty String/Path?(string/path=w1285) -> (empty?=w1287:bool)
                                n1149 = case shown="假" w1287 {
                                tunnel: [w1290 _] -> w1286
                                tunnel: w1285 -> [w1289 _]
                                frame False {
                                n1150 = local read "数据发送通道"() -> (w1288:enum16{"TCP", "VISA"})
                                n1151 = call "数据补发判定有限循环.vi"("数据输入"=w1289, "数据发送通道"=w1288) -> ("error out"=w1290:errorcluster)  [unwired: 9 in]
                                }
                                frame True {
                                }
                                }
                                }
                                frame 14..17 {
                                }
                                }
                              }
                            }
                            n1152 = local read "2011发送"() -> (w1244:bool)
                            n1153 = case shown="真" w1244 {
                              tunnel: w1260 -> [_ w1274]
                              tunnel: w1258 -> [_ w1273]
                              frame False {
                              }
                              frame True {
                                n1154 = local read "MN"() -> (w1268:string)
                                n1155 = local read "PW"() -> (w1267:string)
                                n1156 = global write "全局 实时数据参数.vi" "实时数据参数"("水样测试" ("实时数据参数")) -> ()
                                n1157 = call "数据编码.vi"("table输入"="实时数据" ("新元素/子数组"), "错误常量 2"=w1273, "MN"=w1268, "PW"=w1267) -> ("通讯包字符串"=w1272:string)  [unwired: 10 in, 1 out]
                                n1158 = Build Array(w1272) -> (w1270:string[])
                                n1159 = local read "数据发送通道"() -> (w1266:enum16{"TCP", "VISA"})
                                n1160 = local write "发送报文显示"(w1272) -> ()
                                n1161 = call "发送数据记录到文档(子VI).vi"("数组"=w1270) -> ()  [unwired: 9 in, 1 out]
                                n1162 = call "VISATCP组合选择发送.vi"("数据发送通道"=w1266, "命令"="write", "写入缓冲区"=w1272) -> ("错误输出"=w1271:errorcluster)  [unwired: 9 in, 3 out]
                                n1163 = local read "判断数据反馈"() -> (w1263:bool)
                                n1164 = case shown="真" w1263 {
                                tunnel: w1272 -> [_ w1277]
                                tunnel: w1271 -> [_ w1276]
                                tunnel: w1274 -> [_ w1275]
                                frame False {
                                }
                                frame True {
                                n1165 = case shown="0, 默认" w1275 {
                                tunnel: w1277 -> [w1281 _]
                                tunnel: w1276 -> [w1280 _]
                                frame 0, Default {
                                n1166 = local read "数据发送通道"() -> (w1278:enum16{"TCP", "VISA"})
                                n1167 = call "数据补发判定有限循环.vi"("错误输入（无错误）"=w1280, "数据输入"=w1281, "数据发送通道"=w1278) -> ("error out"=w1279:errorcluster)  [unwired: 8 in]
                                n1168 = local write "错误输出"(w1279) -> ()
                                }
                                frame 14..17 {
                                }
                                }
                                }
                                }
                              }
                            }
                          }
                        }
                      }
                    }
                    frame #2 {
                      n1169 = global read "全局 数据发送重叠.vi" "数据接收超时指示灯"() -> (w1291:bool)
                      n1170 = Not(x=w1291) -> (.not. x?=w1292:bool)
                      n1171 = Compound Arithmetic op=AND ("复合运算")(w1292, w1294) -> (w1293:bool)
                      n1172 = case shown="真" w1293 {
                        tunnel: w1296 -> [_ w1300]
                        tunnel: w1295 -> [_ w1310]
                        tunnel: w1297 -> [_ w1301]
                        frame False {
                        }
                        frame True {
                          n1173 = call "日期时间字符串转换分钟数加一.vi"("data[0]"=w1300) -> ("日期/时间字符串"=w1298:string)  [unwired: 10 in]
                          n1174 = call "时间日期字符串至时间标识转换.vi"("时间日期字符串"=w1298) -> ("时间标识"=w1299:timestamp)  [unwired: 10 in]
                          n1175 = call <vilib>:"Application Directory.vi"() -> ("Application Directory"=w1302:path)
                          n1176 = case shown="3" w1310 {
                            tunnel: w1298 -> [w1311 w1312 w1313 w1314 w1315 w1316 w1317 w1318 w1319 w1320 w1321 w1322 w1323 w1324 w1325 w1326 w1327 w1328]
                            frame 0, Default {
                              n1177 = global write "全局 水样时间.vi" "time1"(w1311) -> ()
                            }
                            frame 1 {
                              n1178 = global write "全局 水样时间.vi" "time2"(w1312) -> ()
                            }
                            frame 2 {
                              n1179 = global write "全局 水样时间.vi" "time3"(w1313) -> ()
                            }
                            frame 3 {
                              n1180 = global write "全局 水样时间.vi" "time4"(w1314) -> ()
                            }
                            frame 4 {
                              n1181 = global write "全局 水样时间.vi" "time5"(w1315) -> ()
                            }
                            frame 5 {
                              n1182 = global write "全局 水样时间.vi" "time6"(w1316) -> ()
                            }
                            frame 6 {
                              n1183 = global write "全局 水样时间.vi" "time7"(w1317) -> ()
                            }
                            frame 7 {
                              n1184 = global write "全局 水样时间.vi" "time8"(w1318) -> ()
                            }
                            frame 8 {
                              n1185 = global write "全局 水样时间.vi" "time9"(w1319) -> ()
                            }
                            frame 9 {
                              n1186 = global write "全局 水样时间.vi" "time10"(w1320) -> ()
                            }
                            frame 10 {
                              n1187 = global write "全局 水样时间.vi" "time11"(w1321) -> ()
                            }
                            frame 11 {
                              n1188 = global write "全局 水样时间.vi" "time12"(w1322) -> ()
                            }
                            frame 12 {
                              n1189 = global write "全局 水样时间.vi" "time13"(w1323) -> ()
                            }
                            frame 13 {
                              n1190 = global write "全局 水样时间.vi" "time14"(w1324) -> ()
                            }
                            frame 14 {
                              n1191 = global write "全局 水样时间.vi" "time15"(w1325) -> ()
                            }
                            frame 15 {
                              n1192 = global write "全局 水样时间.vi" "time16"(w1326) -> ()
                            }
                            frame 16 {
                              n1193 = global write "全局 水样时间.vi" "time17"(w1327) -> ()
                            }
                            frame 17 {
                              n1194 = global write "全局 水样时间.vi" "time18"(w1328) -> ()
                            }
                          }
                          n1195 = Build Path(base path=w1302, name or relative path="data\\Set.ini" ("名称或相对路径")) -> (appended path=w1304:path)
                          n1196 = call <vilib>:"Open Config Data.vi"("configuration file path"=w1304) -> ("error out"=w1306:errorcluster, "refnum"=w1305:T8)  [unwired: 8 in, 1 out]
                          n1197 = local write "数据发送起始时间"(w1299) -> ()
                          n1198 = call-poly <vilib>:"Write Key.vi"("section"="线程一数据搜索起始时间", "error in (no error)"=w1306, "value"=w1298, "key"=w1301, "refnum"=w1305) -> ("error out"=w1308:errorcluster, "refnum out"=w1307:T8)  [unwired: 4 in, 1 out]
                          n1199 = call <vilib>:"Close Config Data.vi"("error in (no error)"=w1308, "refnum"=w1307) -> ()  [unwired: 8 in, 2 out]
                        }
                      }
                    }
                  }
                }
              }
            }
          }
          frame #2 {
            w1383 = FALSE ("小时数据上传")
            n1200 = local write "实时小时数据上传"(w1383) -> ()
            n1201 = global write "全局 数据发送重叠.vi" "主动上报数据中"(w1383) -> ()
          }
        }
      }
    }
  }
  n1202 = while {
    stop <- FALSE stop-if-true
    # "定期释放缓存"
    n1203 = Wait (ms)(milliseconds to wait=u32 600000 ("等待时间（毫秒）")) -> ()  [unwired: 1 out]
    n1204 = dll-call lib="PTH2gabs F\tgitkrakenCC<平台数采程序 - 通用（小时数据单参数传）XINdataFreeMem.dll" fn="FreeMem"() -> ()  [unwired: 4 in, 2 out]
  }
  n1205 = while {
    stop <- FALSE stop-if-true
    n1206 = event shown="[8] \"判断数据反馈\", \"2011发送\", \"日志、参数发送\": 值改变" {
      selector: _ -> [_ _ _ _ _ _ _ _ _ _ _ _ _ _ _ _ _ _]
      dyn-events: _ -> [_ _ _ _ _ _ _ _ _ _ _ _ _ _ _ _ _ _]
      timeout: _ -> [_ _ _ _ _ _ _ _ _ _ _ _ _ _ _ _ _ _]
      event Timeout {
        n1207 = event-data() -> ()  [unwired: 1 in, 2 out]
      }
      event "站点名称", "站点设备", "IP", "PORT", "MN", "PW", "VISA resource name", "baud rate": Value Change {
        w1390 = "线程一自主部署站点保存"
        # "TCP服务器端口掉线"
        n1208 = event-data() -> ()  [unwired: 1 in, 6 out]
        n1209 = call <vilib>:"Application Directory.vi"() -> ("Application Directory"=w1432:path)
        n1210 = local read "站点名称"() -> (w1411:string)
        n1211 = Build Path(base path=w1432, name or relative path="data\\Set.ini" ("名称或相对路径")) -> (appended path=w1430:path)
        n1212 = call <vilib>:"Open Config Data.vi"("configuration file path"=w1430) -> ("error out"=w1428:errorcluster, "refnum"=w1429:T8)  [unwired: 8 in, 1 out]
        n1213 = local read "站点设备"() -> (w1410:string)
        n1214 = call-poly <vilib>:"Write Key.vi"("section"=w1390, "error in (no error)"=w1428, "value"=w1411, "key"="站点名称", "refnum"=w1429) -> ("error out"=w1425:errorcluster, "refnum out"=w1426:T8)  [unwired: 4 in, 1 out]
        n1215 = call-poly <vilib>:"Write Key.vi"("section"=w1390, "error in (no error)"=w1425, "value"=w1410, "key"="站点设备", "refnum"=w1426) -> ("error out"=w1422:errorcluster, "refnum out"=w1423:T8)  [unwired: 4 in, 1 out]
        n1216 = local read "IP"() -> (w1409:string)
        n1217 = call-poly <vilib>:"Write Key.vi"("section"=w1390, "error in (no error)"=w1422, "value"=w1409, "key"="IP", "refnum"=w1423) -> ("error out"=w1420:errorcluster, "refnum out"=w1421:T8)  [unwired: 4 in, 1 out]
        n1218 = local read "PORT"() -> (w1408:string)
        n1219 = call-poly <vilib>:"Write Key.vi"("section"=w1390, "error in (no error)"=w1420, "value"=w1408, "key"="PORT", "refnum"=w1421) -> ("error out"=w1418:errorcluster, "refnum out"=w1419:T8)  [unwired: 4 in, 1 out]
        n1220 = local read "MN"() -> (w1402:string)
        n1221 = call-poly <vilib>:"Write Key.vi"("section"=w1390, "error in (no error)"=w1418, "value"=w1402, "key"="MN", "refnum"=w1419) -> ("error out"=w1403:errorcluster, "refnum out"=w1406:T8)  [unwired: 4 in, 1 out]
        n1222 = local read "PW"() -> (w1404:string)
        n1223 = call-poly <vilib>:"Write Key.vi"("section"=w1390, "error in (no error)"=w1403, "value"=w1404, "key"="PW", "refnum"=w1406) -> ("error out"=w1391:errorcluster, "refnum out"=w1392:T8)  [unwired: 4 in, 1 out]
        n1224 = local read "VISA resource name"() -> (w1398:refnum<visa-resource-name>)
        n1225 = local read "主队列输出"() -> (w1417:refnum<queue>)
        n1226 = call-poly <vilib>:"Write Key.vi"("section"=w1390, "error in (no error)"=w1391, "value"=w1398, "key"="VISA", "refnum"=w1392) -> ("error out"=w1397:errorcluster, "refnum out"=w1394:T8)  [unwired: 4 in, 1 out]
        n1227 = local read "baud rate"() -> (w1396:u32)
        n1228 = Flush Queue(queue=w1417) -> (queue out=w1416:refnum<queue>)  [unwired: 1 in, 2 out]
        n1229 = call-poly <vilib>:"Write Key.vi"("section"=w1390, "error in (no error)"=w1397, "value"=w1396, "key"="BAUDRATE", "refnum"=w1394) -> ("error out"=w1388:errorcluster, "refnum out"=w1389:T8)  [unwired: 4 in, 1 out]
        n1230 = local read "数据发送通道"() -> (w1401:enum16{"TCP", "VISA"})
        n1231 = call <vilib>:"Close Config Data.vi"("error in (no error)"=w1388, "refnum"=w1389) -> ()  [unwired: 8 in, 2 out]
        n1232 = call "VISATCP组合选择发送.vi"("数据发送通道"=w1401, "命令"="close") -> ("错误输出"=w1399:errorcluster)  [unwired: 10 in, 3 out]
        n1233 = Enqueue Element(queue=w1416, element=T6."初始化" ("元素"), timeout in ms (-1)=1000 ("超时毫秒(-1)")) -> ()  [unwired: 1 in, 3 out]
        n1234 = call <vilib>:"Clear Errors.vi"("error in (no error)"=w1399) -> ()  [unwired: 5 in, 2 out]
      }
      event "确定": Value Change {
        w1437 = "线程一自主部署站点保存"
        # "TCP服务器端口掉线"
        n1235 = event-data() -> ()  [unwired: 1 in, 6 out]
        n1236 = call <vilib>:"Application Directory.vi"() -> ("Application Directory"=w1470:path)
        n1237 = local read "站点名称"() -> (w1465:string)
        n1238 = Build Path(base path=w1470, name or relative path="data\\Set.ini" ("名称或相对路径")) -> (appended path=w1468:path)
        n1239 = call <vilib>:"Open Config Data.vi"("configuration file path"=w1468) -> ("error out"=w1466:errorcluster, "refnum"=w1467:T8)  [unwired: 8 in, 1 out]
        n1240 = local read "站点设备"() -> (w1460:string)
        n1241 = call-poly <vilib>:"Write Key.vi"("section"=w1437, "error in (no error)"=w1466, "value"=w1465, "key"="站点名称", "refnum"=w1467) -> ("error out"=w1462:errorcluster, "refnum out"=w1463:T8)  [unwired: 4 in, 1 out]
        n1242 = call-poly <vilib>:"Write Key.vi"("section"=w1437, "error in (no error)"=w1462, "value"=w1460, "key"="站点设备", "refnum"=w1463) -> ("error out"=w1458:errorcluster, "refnum out"=w1459:T8)  [unwired: 4 in, 1 out]
        n1243 = local read "IP"() -> (w1453:string)
        n1244 = local read "PORT"() -> (w1452:string)
        n1245 = call-poly <vilib>:"Write Key.vi"("section"=w1437, "error in (no error)"=w1458, "value"=w1453, "key"="IP", "refnum"=w1459) -> ("error out"=w1456:errorcluster, "refnum out"=w1457:T8)  [unwired: 4 in, 1 out]
        n1246 = call-poly <vilib>:"Write Key.vi"("section"=w1437, "error in (no error)"=w1456, "value"=w1452, "key"="PORT", "refnum"=w1457) -> ("error out"=w1448:errorcluster, "refnum out"=w1449:T8)  [unwired: 4 in, 1 out]
        n1247 = local read "MN"() -> (w1445:string)
        n1248 = call-poly <vilib>:"Write Key.vi"("section"=w1437, "error in (no error)"=w1448, "value"=w1445, "key"="MN", "refnum"=w1449) -> ("error out"=w1446:errorcluster, "refnum out"=w1447:T8)  [unwired: 4 in, 1 out]
        n1249 = local read "PW"() -> (w1444:string)
        n1250 = call-poly <vilib>:"Write Key.vi"("section"=w1437, "error in (no error)"=w1446, "value"=w1444, "key"="PW", "refnum"=w1447) -> ("error out"=w1442:errorcluster, "refnum out"=w1443:T8)  [unwired: 4 in, 1 out]
        n1251 = call <vilib>:"Close Config Data.vi"("error in (no error)"=w1442, "refnum"=w1443) -> ("error out"=w1436:errorcluster)  [unwired: 8 in, 1 out]
        n1252 = local read "主队列输出"() -> (w1441:refnum<queue>)
        n1253 = local read "数据发送通道"() -> (w1435:enum16{"TCP", "VISA"})
        n1254 = call "VISATCP组合选择发送.vi"("数据发送通道"=w1435, "命令"="close") -> ("错误输出"=w1433:errorcluster)  [unwired: 10 in, 3 out]
        n1255 = Flush Queue(queue=w1441) -> (queue out=w1440:refnum<queue>)  [unwired: 1 in, 2 out]
        n1256 = case shown="错误" w1436 {
          frame No Error {
            n1257 = One Button Dialog(message="保存成功" ("消息"), button name ("OK")="确定" ("按钮名称（“确定”）")) -> ()  [unwired: 1 out]
          }
          frame Error {
            n1258 = One Button Dialog(message="保存失败" ("消息"), button name ("OK")="确定" ("按钮名称（“确定”）")) -> ()  [unwired: 1 out]
          }
        }
        n1259 = call <vilib>:"Clear Errors.vi"("error in (no error)"=w1433) -> ()  [unwired: 5 in, 2 out]
        n1260 = Enqueue Element(queue=w1440, element=T6."初始化" ("元素"), timeout in ms (-1)=1000 ("超时毫秒(-1)")) -> ()  [unwired: 1 in, 3 out]
      }
      event "参数配置": Value Change {
        n1261 = event-data() -> ()  [unwired: 1 in, 6 out]
        n1262 = property on="窗格" class="Pane"("Origin"=T11 {"Horizontal"=0, "Vertical"=1000} ("原点")) -> ()  [unwired: 2 in, 2 out]
      }
      event "返回": Value Change {
        n1263 = event-data() -> ()  [unwired: 1 in, 6 out]
        n1264 = property on="窗格" class="Pane"("Origin"=T11 {"Horizontal"=0, "Vertical"=0} ("原点")) -> ()  [unwired: 2 in, 2 out]
      }
      event "系统编码选择框": Value Change {
        n1265 = event-data() -> ()  [unwired: 1 in, 6 out]
        n1266 = call <vilib>:"Application Directory.vi"() -> ("Application Directory"=w1485:path)
        n1267 = Build Path(base path=w1485, name or relative path="data\\Set.ini" ("名称或相对路径")) -> (appended path=w1486:path)
        n1268 = call <vilib>:"Open Config Data.vi"("configuration file path"=w1486) -> ("error out"=w1482:errorcluster, "refnum"=w1483:T8)  [unwired: 8 in, 1 out]
        n1269 = call-poly <vilib>:"Write Key.vi"("section"="系统编码选择", "error in (no error)"=w1482, "value"="系统编码选择框", "key"="系统编码", "refnum"=w1483) -> ("error out"=w1480:errorcluster, "refnum out"=w1481:T8)  [unwired: 4 in, 1 out]
        n1270 = call <vilib>:"Close Config Data.vi"("error in (no error)"=w1480, "refnum"=w1481) -> ()  [unwired: 8 in, 2 out]
      }
      event "数据发送通道": Value Change {
        w1487 = "数据发送通道"
        n1271 = event-data() -> ()  [unwired: 1 in, 6 out]
        n1272 = local read "数据发送通道"() -> (w1488:enum16{"TCP", "VISA"})
        n1273 = call <vilib>:"Application Directory.vi"() -> ("Application Directory"=w1494:path)
        n1274 = Build Path(base path=w1494, name or relative path="data\\Set.ini" ("名称或相对路径")) -> (appended path=w1495:path)
        n1275 = call <vilib>:"Open Config Data.vi"("configuration file path"=w1495) -> ("error out"=w1491:errorcluster, "refnum"=w1492:T8)  [unwired: 8 in, 1 out]
        n1276 = call-poly <vilib>:"Write Key.vi"("section"=w1487, "error in (no error)"=w1491, "value"=w1488, "key"=w1487, "refnum"=w1492) -> ("error out"=w1489:errorcluster, "refnum out"=w1490:T8)  [unwired: 4 in, 1 out]
        n1277 = call <vilib>:"Close Config Data.vi"("error in (no error)"=w1489, "refnum"=w1490) -> ()  [unwired: 8 in, 2 out]
      }
      event "数据发送协议": Value Change {
        w1497 = "数据发送协议"
        n1278 = event-data() -> ()  [unwired: 1 in, 6 out]
        n1279 = call <vilib>:"Application Directory.vi"() -> ("Application Directory"=w1503:path)
        n1280 = Build Path(base path=w1503, name or relative path="data\\Set.ini" ("名称或相对路径")) -> (appended path=w1504:path)
        n1281 = call <vilib>:"Open Config Data.vi"("configuration file path"=w1504) -> ("error out"=w1500:errorcluster, "refnum"=w1501:T8)  [unwired: 8 in, 1 out]
        n1282 = call-poly <vilib>:"Write Key.vi"("section"=w1497, "error in (no error)"=w1500, "value"="数据发送协议", "key"=w1497, "refnum"=w1501) -> ("error out"=w1498:errorcluster, "refnum out"=w1499:T8)  [unwired: 4 in, 1 out]
        n1283 = call <vilib>:"Close Config Data.vi"("error in (no error)"=w1498, "refnum"=w1499) -> ()  [unwired: 8 in, 2 out]
      }
      event "判断数据反馈", "2011发送", "日志、参数发送": Value Change {
        n1284 = event-data() -> ()  [unwired: 1 in, 6 out]
        n1285 = flat-sequence {
          frame #0 {
            n1286 = global write "断电保存全局.vi" "日志、参数发送"("日志、参数发送") -> ()
            n1287 = global write "断电保存全局.vi" "判断数据反馈"("判断数据反馈") -> ()
            n1288 = global write "断电保存全局.vi" "2011发送"("2011发送") -> ()
          }
          frame #1 {
            n1289 = call <vilib>:"Application Directory.vi"() -> ("Application Directory"=w1508:path)
            n1290 = Build Path(base path=w1508, name or relative path="data\\sys.ini" ("名称或相对路径")) -> (appended path=w1510:path)
            n1291 = call <vilib>:"Open Config Data.vi"("configuration file path"=w1510) -> ("error out"=w1514:errorcluster, "refnum"=w1511:T8)  [unwired: 8 in, 1 out]
            n1292 = vi-ref "断电保存全局.vi"() -> (w1512:refnum<vi>)
            n1293 = call <userlib>:"Write Panel to INI__ogtk.vi"("error in (no error)"=w1514, "VI ref"=w1512, "refnum"=w1511) -> ("error out"=w1515:errorcluster, "refnum out"=w1513:T8)  [unwired: 7 in]
            n1294 = call <vilib>:"Close Config Data.vi"("error in (no error)"=w1515, "refnum"=w1513) -> ("error out"=w1520:errorcluster, "file path"=w1521:path)  [unwired: 8 in]
            n1295 = Open/Create/Replace File(file path (use dialog)=w1521, error in=w1520) -> (refnum out=w1517:refnum<file>, error out=w1516:errorcluster)  [unwired: 4 in, 1 out]
            n1296 = Flush File(refnum=w1517, error in=w1516) -> (refnum out=w1518:refnum<file>, error out=w1519:errorcluster)
            n1297 = Close File(refnum=w1518, error in=w1519) -> ()  [unwired: 2 out]
          }
        }
      }
      event "每周自动重发": Value Change {
        n1298 = event-data() -> ()  [unwired: 1 in, 6 out]
        n1299 = call <vilib>:"Application Directory.vi"() -> ("Application Directory"=w1530:path)
        n1300 = Build Path(base path=w1530, name or relative path="data\\Set.ini" ("名称或相对路径")) -> (appended path=w1531:path)
        n1301 = local read "每周自动重发"() -> (w1522:bool)
        n1302 = call <vilib>:"Open Config Data.vi"("configuration file path"=w1531) -> ("error out"=w1527:errorcluster, "refnum"=w1528:T8)  [unwired: 8 in, 1 out]
        n1303 = call-poly <vilib>:"Write Key.vi"("section"="线程一数据重发功能", "error in (no error)"=w1527, "value"=w1522, "key"="重发功能", "refnum"=w1528) -> ("error out"=w1525:errorcluster, "refnum out"=w1526:T8)  [unwired: 4 in, 1 out]
        n1304 = call <vilib>:"Close Config Data.vi"("error in (no error)"=w1525, "refnum"=w1526) -> ()  [unwired: 8 in, 2 out]
      }
      event "重发日期": Value Change {
        n1305 = event-data() -> ()  [unwired: 1 in, 6 out]
        n1306 = call <vilib>:"Application Directory.vi"() -> ("Application Directory"=w1540:path)
        n1307 = Build Path(base path=w1540, name or relative path="data\\Set.ini" ("名称或相对路径")) -> (appended path=w1541:path)
        n1308 = local read "重发日期"() -> (w1532:T2)
        n1309 = call <vilib>:"Open Config Data.vi"("configuration file path"=w1541) -> ("error out"=w1537:errorcluster, "refnum"=w1538:T8)  [unwired: 8 in, 1 out]
        n1310 = call-poly <vilib>:"Write Key.vi"("section"="线程一数据重发功能", "error in (no error)"=w1537, "value"=w1532, "key"="重发日期", "refnum"=w1538) -> ("error out"=w1535:errorcluster, "refnum out"=w1536:T8)  [unwired: 4 in, 1 out]
        n1311 = call <vilib>:"Close Config Data.vi"("error in (no error)"=w1535, "refnum"=w1536) -> ()  [unwired: 8 in, 2 out]
      }
      event "重发时间": Value Change {
        n1312 = event-data() -> ()  [unwired: 1 in, 6 out]
        n1313 = call <vilib>:"Application Directory.vi"() -> ("Application Directory"=w1550:path)
        n1314 = Build Path(base path=w1550, name or relative path="data\\Set.ini" ("名称或相对路径")) -> (appended path=w1551:path)
        n1315 = local read "重发时间"() -> (w1542:T1)
        n1316 = call <vilib>:"Open Config Data.vi"("configuration file path"=w1551) -> ("error out"=w1547:errorcluster, "refnum"=w1548:T8)  [unwired: 8 in, 1 out]
        n1317 = call-poly <vilib>:"Write Key.vi"("section"="线程一数据重发功能", "error in (no error)"=w1547, "value"=w1542, "key"="重发时间", "refnum"=w1548) -> ("error out"=w1545:errorcluster, "refnum out"=w1546:T8)  [unwired: 4 in, 1 out]
        n1318 = call <vilib>:"Close Config Data.vi"("error in (no error)"=w1545, "refnum"=w1546) -> ()  [unwired: 8 in, 2 out]
      }
      event "确定更改起始时间": Value Change {
        n1319 = event-data() -> ()  [unwired: 1 in, 6 out]
        n1320 = local write "更改起始时间"(FALSE ("更改起始时间")) -> ()
        n1321 = Two Button Dialog(message="确定以当前设置时间作为数据索引起始时间？" ("消息")) -> (T button?=w1553:bool)  [unwired: 2 in]
        n1322 = case shown="真" w1553 {
          frame False {
          }
          frame True {
            n1323 = local read "参数数值"() -> (w1557:T5)
            n1324 = Cluster To Array(cluster=w1557) -> (array=w1558:bool[])
            n1325 = for {
              tunnel: w1558 -> [_] mode=indexing
              tunnel: [w1566] -> w1555
              i -> [w1567]
              n1326 = Format Date/Time String(time format string (%c)="%Y/%m/%d %H:%M:%S" ("时间格式字符串(%c)"), seconds (now)="数据发送起始时间") -> (date/time string=w1566:string)  [unwired: 1 in]
              n1327 = case shown="0, 默认" w1567 {
                tunnel: w1566 -> [w1570 w1571 w1572 w1573 w1574 w1575 w1576 w1577 w1578 w1579 w1580 w1581 w1582 w1583 w1584 w1585 w1586 w1587]
                frame 0, Default {
                  n1328 = global write "全局 水样时间.vi" "time1"(w1570) -> ()
                }
                frame 1 {
                  n1329 = global write "全局 水样时间.vi" "time2"(w1571) -> ()
                }
                frame 2 {
                  n1330 = global write "全局 水样时间.vi" "time3"(w1572) -> ()
                }
                frame 3 {
                  n1331 = global write "全局 水样时间.vi" "time4"(w1573) -> ()
                }
                frame 4 {
                  n1332 = global write "全局 水样时间.vi" "time5"(w1574) -> ()
                }
                frame 5 {
                  n1333 = global write "全局 水样时间.vi" "time6"(w1575) -> ()
                }
                frame 6 {
                  n1334 = global write "全局 水样时间.vi" "time7"(w1576) -> ()
                }
                frame 7 {
                  n1335 = global write "全局 水样时间.vi" "time8"(w1577) -> ()
                }
                frame 8 {
                  n1336 = global write "全局 水样时间.vi" "time9"(w1578) -> ()
                }
                frame 9 {
                  n1337 = global write "全局 水样时间.vi" "time10"(w1579) -> ()
                }
                frame 10 {
                  n1338 = global write "全局 水样时间.vi" "time11"(w1580) -> ()
                }
                frame 11 {
                  n1339 = global write "全局 水样时间.vi" "time12"(w1581) -> ()
                }
                frame 12 {
                  n1340 = global write "全局 水样时间.vi" "time13"(w1582) -> ()
                }
                frame 13 {
                  n1341 = global write "全局 水样时间.vi" "time14"(w1583) -> ()
                }
                frame 14 {
                  n1342 = global write "全局 水样时间.vi" "time15"(w1584) -> ()
                }
                frame 15 {
                  n1343 = global write "全局 水样时间.vi" "time16"(w1585) -> ()
                }
                frame 16 {
                  n1344 = global write "全局 水样时间.vi" "time17"(w1586) -> ()
                }
                frame 17 {
                  n1345 = global write "全局 水样时间.vi" "time18"(w1587) -> ()
                }
              }
            }
            n1346 = global write "全局 时间2.vi" "跨度核查索引起始时间"(w1555) -> ()
            n1347 = global write "全局 时间2.vi" "标样核查索引起始时间"(w1555) -> ()
            n1348 = global write "全局 时间2.vi" "零点核查索引起始时间"(w1555) -> ()
            n1349 = global write "全局 时间2.vi" "加标回收索引起始时间"(w1555) -> ()
            n1350 = for {
              N: 5 -> [_]
              tunnel: w1555 -> [w1559]
              i -> [w1560]
              n1351 = case shown="4" w1560 {
                tunnel: w1559 -> [w1561 w1562 w1563 w1564 w1565]
                frame 0, Default {
                  n1352 = global write "全局 时间2.vi" "氨氮跨度核查索引起始时间"(w1561) -> ()
                  n1353 = global write "全局 时间2.vi" "氨氮零点核查索引起始时间"(w1561) -> ()
                }
                frame 1 {
                  n1354 = global write "全局 时间2.vi" "总氮跨度核查索引起始时间"(w1562) -> ()
                  n1355 = global write "全局 时间2.vi" "总氮零点核查索引起始时间"(w1562) -> ()
                }
                frame 2 {
                  n1356 = global write "全局 时间2.vi" "总磷跨度核查索引起始时间"(w1563) -> ()
                  n1357 = global write "全局 时间2.vi" "总磷零点核查索引起始时间"(w1563) -> ()
                }
                frame 3 {
                  n1358 = global write "全局 时间2.vi" "CODMn跨度核查索引起始时间"(w1564) -> ()
                  n1359 = global write "全局 时间2.vi" "CODMn零点核查索引起始时间"(w1564) -> ()
                }
                frame 4 {
                  n1360 = global write "全局 时间2.vi" "CODCr跨度核查索引起始时间"(w1565) -> ()
                  n1361 = global write "全局 时间2.vi" "CODCr零点核查索引起始时间"(w1565) -> ()
                }
              }
            }
          }
        }
      }
      event "开机启动": Value Change {
        n1362 = event-data() -> ("NewVal"=w1588:bool)  [unwired: 1 in, 5 out]
        n1363 = case shown="假" w1588 {
          frame False {
            n1364 = Two Button Dialog(message="是否删除开机启动" ("消息"), 1:"否" ("F按钮名称（“取消”）"), 2:"是" ("T按钮名称（“确定”）")) -> (T button?=w1589:bool)
            n1365 = case shown="真" w1589 {
              frame False {
              }
              frame True {
                n1366 = call <vilib>:"Application Directory.vi"() -> ("Application Directory"=w1594:path)
                n1367 = call "删除启动项.vi"("启动文件路径"=w1594) -> ("删除标记"=w1593:bool)  [unwired: 9 in, 1 out]
                n1368 = case shown="假" w1593 {
                  tunnel: ["删除开机启动失败" ("T按钮名称（“确定”）") "删除开机启动成功" ("T按钮名称（“确定”）")] -> w1595
                  frame False {
                  }
                  frame True {
                  }
                }
                n1369 = One Button Dialog(message=w1595) -> ()  [unwired: 1 in, 1 out]
              }
            }
          }
          frame True {
            n1370 = Two Button Dialog(message="是否添加开机启动" ("消息"), 1:"否" ("F按钮名称（“取消”）"), 2:"是" ("T按钮名称（“确定”）")) -> (T button?=w1598:bool)
            n1371 = case shown="真" w1598 {
              frame False {
              }
              frame True {
                n1372 = call <vilib>:"Application Directory.vi"() -> ("Application Directory"=w1604:path)
                n1373 = call "添加启动项.vi"("启动文件路径"=w1604) -> ("添加成功标记"=w1603:bool)  [unwired: 9 in, 1 out]
                n1374 = case shown="真" w1603 {
                  tunnel: ["添加开机启动失败" ("T按钮名称（“确定”）") "添加开机启动成功" ("T按钮名称（“确定”）")] -> w1602
                  frame False {
                  }
                  frame True {
                  }
                }
                n1375 = One Button Dialog(message=w1602) -> ()  [unwired: 1 in, 1 out]
              }
            }
          }
        }
      }
      event "IP": Mouse Down {
        n1376 = event-data() -> ("CtlRef"=w1607:refnum<vi>)  [unwired: 1 in, 5 out]
        n1377 = property class="Str" props=["Value"](reference=w1607) -> ()  [unwired: 1 in, 3 out]
        n1378 = local read "IP"() -> (w1609:string)
        n1379 = call "IP键盘.vi"("OldNumber"=w1609) -> ("NewNumber"=w1608:string)
        n1380 = local write "IP"(w1608) -> ()
      }
      event "PORT": Mouse Down {
        n1381 = event-data() -> ()  [unwired: 1 in, 6 out]
        n1382 = local read "PORT"() -> (w1611:string)
        n1383 = call "IP键盘.vi"("OldNumber"=w1611) -> ("NewNumber"=w1610:string)
        n1384 = local write "PORT"(w1610) -> ()
      }
      event "查询质控数据起始时间": Value Change {
        n1385 = event-data() -> ()  [unwired: 1 in, 6 out]
        n1386 = property on="窗格" class="Pane"("Origin"=T11 {"Horizontal"=1000, "Vertical"=0} ("原点")) -> ()  [unwired: 2 in, 2 out]
      }
      event "返回主界面": Value Change {
        n1387 = event-data() -> ()  [unwired: 1 in, 6 out]
        n1388 = property on="窗格" class="Pane"("Origin"=T11 {"Horizontal"=0, "Vertical"=0} ("原点")) -> ()  [unwired: 2 in, 2 out]
      }
    }
  }
  n1389 = while {
    stop <- FALSE stop-if-true
    # "心跳包"
    n1390 = local read "实时小时数据上传"() -> (w1660:bool)
    n1391 = global read "全局 数据发送重叠.vi" "掉线指示灯"() -> (→"掉线指示":bool)
    n1392 = Get Date/Time In Seconds() -> (seconds since 1Jan1904=w1651:timestamp)
    n1393 = local read "数据发送通道"() -> (w1625:enum16{"TCP", "VISA"})
    n1394 = local read "空闲时间"() -> (w1643:dbl)
    n1395 = case shown="\"VISA\"" "数据发送通道" {
      tunnel: [w1683 w1686] -> w1629
      tunnel: [w1682 w1684] -> w1628
      frame "TCP", Default {
        n1396 = local read "PORT"() -> (w1682:string)
        n1397 = local read "IP"() -> (w1683:string)
      }
      frame "VISA" {
        n1398 = local read "baud rate"() -> (w1685:u32)
        n1399 = local read "VISA resource name"() -> (w1686:refnum<visa-resource-name>)
        n1400 = Number To Decimal String(number=w1685) -> (decimal integer string=w1684:string)  [unwired: 1 in]
      }
    }
    n1401 = Wait (ms)(milliseconds to wait=u32 1000 ("等待时间（毫秒）")) -> ()  [unwired: 1 out]
    n1402 = local read "实时小时数据上传"() -> (w1640:bool)
    n1403 = local read "核查数据上传"() -> (w1637:bool)
    n1404 = local read "空闲时间"() -> (w1675:dbl)
    n1405 = local read "查询数据发送"() -> (w1641:bool)
    n1406 = Number To Decimal String(number=w1643) -> (decimal integer string=→"空闲时间/s":string)  [unwired: 1 in]
    n1407 = local read "站点设备"() -> (w1630:string)
    n1408 = local read "站点名称"() -> (w1631:string)
    n1409 = global read "全局 数据发送重叠.vi" "数据接收超时指示灯"() -> (→"数据接收超时指示灯":bool)
    n1410 = global write "全局 数据发送重叠.vi" "主动上报数据中"(w1660) -> ()
    n1411 = local read "MN"() -> (w1627:string)
    n1412 = Format Date/Time String(time format string (%c)="%Y/%m/%d %H:%M:%S" ("时间格式字符串(%c)"), seconds (now)=w1651) -> (date/time string=→"系统时间":string)  [unwired: 1 in]
    n1413 = local read "PW"() -> (w1626:string)
    n1414 = local read "步骤"() -> (w1669:T6)
    n1415 = case shown="\"TCP\", 默认" w1625 {
      frame "TCP", Default {
        w1687 = TRUE ("可见")
        w1688 = FALSE ("可见")
        n1416 = property on="VISA resource name" class="VISAName"("Visible"=w1688) -> ()  [unwired: 2 in, 2 out]
        n1417 = property on="baud rate" class="DigNum (严格)"("Visible"=w1688) -> ()  [unwired: 2 in, 2 out]
        n1418 = property on="IP" class="Str"("Visible"=w1687) -> ()  [unwired: 2 in, 2 out]
        n1419 = property on="PORT" class="Str"("Visible"=w1687) -> ()  [unwired: 2 in, 2 out]
      }
      frame "VISA" {
        w1689 = TRUE ("可见")
        w1690 = FALSE ("可见")
        n1420 = property on="baud rate" class="DigNum (严格)"("Visible"=w1689) -> ()  [unwired: 2 in, 2 out]
        n1421 = property on="VISA resource name" class="VISAName"("Visible"=w1689) -> ()  [unwired: 2 in, 2 out]
        n1422 = property on="IP" class="Str"("Visible"=w1690) -> ()  [unwired: 2 in, 2 out]
        n1423 = property on="PORT" class="Str"("Visible"=w1690) -> ()  [unwired: 2 in, 2 out]
      }
    }
    n1424 = local read "数据发送协议"() -> (w1622:enum16{"2005-212协议", "2017-212协议"})
    n1425 = Not(x=w1637) -> (.not. x?=w1638:bool)
    n1426 = Greater?(x=w1675, y=30.0) -> (0:w1673:bool)
    n1427 = Not(x=w1640) -> (.not. x?=w1639:bool)
    n1428 = property on="数据发送通道" class="Enum (严格)"("Visible"="锁") -> ()  [unwired: 2 in, 2 out]
    n1429 = Not(x=w1641) -> (.not. x?=w1663:bool)
    n1430 = Equal?(x=w1669, y=T6."读取数据" ("步骤")) -> (x = y?=w1667:bool)
    n1431 = Bundle By Name(cluster=T4 {"站点"="", "设备"="", "IP"="", "PORT"="", "MN"="", "PW"=""} ("配置信息"), "站点"=w1631, "设备"=w1630, "IP"=w1629, "PORT"=w1628, "MN"=w1627, "PW"=w1626) -> (→"配置信息":T4)
    n1432 = Select(t=T12."Enabled" ("禁用"), s="更改起始时间", f=T12."Disabled and Grayed Out" ("禁用")) -> (s? t:f=w1654:T12)
    n1433 = case shown="真" w1673 {
      tunnel: w1673 -> [_ w1700]
      tunnel: [FALSE w1700] -> w1670
      frame False {
      }
      frame True {
        n1434 = local read "QN"() -> (w1698:string)
        n1435 = local write "空闲时间"(0.0 ("空闲时间")) -> ()
        n1436 = local read "MN"() -> (w1697:string)
        n1437 = local read "PW"() -> (w1696:string)
        n1438 = local read "数据发送通道"() -> (w1695:enum16{"TCP", "VISA"})
        n1439 = call "数据编码.vi"("table输入"="心跳包", "QN"=w1698, "MN"=w1697, "PW"=w1696) -> ("通讯包字符串"=w1693:string)  [unwired: 10 in, 1 out]
        n1440 = local write "发送报文显示"(w1693) -> ()
        n1441 = call "VISATCP组合选择发送.vi"("数据发送通道"=w1695, "命令"="write", "写入缓冲区"=w1693) -> ("错误输出"=w1692:errorcluster)  [unwired: 9 in, 3 out]
        n1442 = call <vilib>:"Clear Errors.vi"("error in (no error)"=w1692) -> ()  [unwired: 5 in, 2 out]
      }
    }
    "心跳包" <- w1670
    n1443 = Select(t=T12."Enabled" ("禁用"), s="锁", f=T12."Disabled and Grayed Out" ("禁用")) -> (s? t:f=w1614:T12)
    n1444 = property on="数据发送起始时间" class="AbsTime (严格)"("DisabledEnum"=w1654) -> ()  [unwired: 2 in, 2 out]
    n1445 = global read "全局 时间2.vi" "跨度核查索引起始时间"() -> (→"跨度核查索引起始时间":string)
    n1446 = case shown="\"2005-212协议\"" w1622 {
      tunnel: ["32" ("设备编码MN") w1677] -> w1661
      frame "2005-212协议" {
      }
      frame "2017-212协议", Default {
        n1447 = local read "系统编码选择框"() -> (w1678:string)
        n1448 = case shown="\"地表水体污染源\"" w1678 {
          tunnel: ["52" ("设备编码MN") "32" ("设备编码MN") "21" ("设备编码MN")] -> w1677
          frame "污水排放过程监测" {
          }
          frame "地表水体污染源" {
          }
          frame "地表水质量监测", Default {
          }
        }
      }
    }
    n1449 = global read "全局 时间2.vi" "标样核查索引起始时间"() -> (→"标样核查索引起始时间":string)
    n1450 = global read "全局 时间2.vi" "零点核查索引起始时间"() -> (→"零点核查索引起始时间":string)
    n1451 = global read "全局 时间2.vi" "加标回收索引起始时间"() -> (→"加标回收索引起始时间":string)
    n1452 = property on="设置超时时间/min" class="DigNum (严格)"("DisabledEnum"=w1614) -> ()  [unwired: 2 in, 2 out]
    n1453 = property on="IP" class="Str"("DisabledEnum"=w1614) -> ()  [unwired: 2 in, 2 out]
    n1454 = property on="每周自动重发" class="Bool (严格)"("DisabledEnum"=w1614) -> ()  [unwired: 2 in, 2 out]
    n1455 = property on="PORT" class="Str"("DisabledEnum"=w1614) -> ()  [unwired: 2 in, 2 out]
    n1456 = local read "数据发送协议"() -> (w1621:enum16{"2005-212协议", "2017-212协议"})
    n1457 = local read "TCP服务端掉线计数"() -> (w1646:i32)
    n1458 = local read "1st Error to Convert"() -> (w1649:i32)
    n1459 = local read "TCP掉线时间节点"() -> (w1645:string)
    n1460 = property on="确定更改起始时间" class="Bool"("DisabledEnum"=w1654) -> ()  [unwired: 2 in, 2 out]
    n1461 = property on="MN" class="Str"("DisabledEnum"=w1614) -> ()  [unwired: 2 in, 2 out]
    n1462 = property on="PW" class="Str"("DisabledEnum"=w1614) -> ()  [unwired: 2 in, 2 out]
    n1463 = property on="实时数据发送时间间隔/min" class="DigNum (严格)"("DisabledEnum"=w1614) -> ()  [unwired: 2 in, 2 out]
    n1464 = local read "元素"() -> (w1647:string)
    n1465 = local read "步骤"() -> (w1648:T6)
    n1466 = Equal?(x=w1621, y=enum16{"2005-212协议", "2017-212协议"}."2017-212协议" ("数据发送协议")) -> (x = y?=w1619:bool)
    n1467 = Compound Arithmetic op=AND ("复合运算")(w1619, w1667, w1663, w1639, w1638) -> (w1664:bool)
    n1468 = case shown="真" w1664 {
      frame False {
      }
      frame True {
        n1469 = local read "空闲时间"() -> (w1703:dbl)
        n1470 = Increment(x=w1703) -> (x+1=→"空闲时间":dbl)
      }
    }
    n1471 = property on="数据发送通道" class="Enum (严格)"("DisabledEnum"=w1614) -> ()  [unwired: 2 in, 2 out]
    n1472 = Bundle By Name(cluster=T3 {"1st Error to Convert "=54, "步骤 "=enum."打开连接", "元素"="实时数据", "TCP服务端掉线计数"=4, "TCP掉线时间节点"="2019/05/08 15:24:17"} ("状态信息"), "1st Error to Convert"=w1649, "步骤"=w1648, "元素"=w1647, "TCP服务端掉线计数"=w1646, "TCP掉线时间节点"=w1645) -> (→"状态信息":T3)
    n1473 = property on="重发时间" class="Enum (严格)"("DisabledEnum"=w1614) -> ()  [unwired: 2 in, 2 out]
    n1474 = property on="重发日期" class="Enum (严格)"("DisabledEnum"=w1614) -> ()  [unwired: 2 in, 2 out]
    n1475 = property on="VISA resource name" class="VISAName"("DisabledEnum"=w1614) -> ()  [unwired: 2 in, 2 out]
    n1476 = property on="判断数据反馈" class="Bool (严格)"("DisabledEnum"=w1614) -> ()  [unwired: 2 in, 2 out]
    n1477 = property on="baud rate" class="DigNum (严格)"("DisabledEnum"=w1614) -> ()  [unwired: 2 in, 2 out]
    n1478 = property on="数据发送协议" class="Enum (严格)"("DisabledEnum"=w1614) -> ()  [unwired: 2 in, 2 out]
    n1479 = property on="2011发送" class="Bool (严格)"("DisabledEnum"=w1614) -> ()  [unwired: 2 in, 2 out]
    n1480 = global write "全局1.vi" "系统编码ST"(w1661) -> ()
    n1481 = property on="日志、参数发送" class="Bool (严格)"("DisabledEnum"=w1614) -> ()  [unwired: 2 in, 2 out]
    n1482 = global read "断电保存全局.vi" "日志、参数发送"() -> (w1615:bool)
    n1483 = global read "断电保存全局.vi" "判断数据反馈"() -> (w1617:bool)
    n1484 = local read "数据发送协议"() -> (w1618:enum16{"2005-212协议", "2017-212协议"})
    n1485 = global read "断电保存全局.vi" "2011发送"() -> (w1616:bool)
    n1486 = local write "日志、参数发送"(w1615) -> ()
    n1487 = local write "判断数据反馈"(w1617) -> ()
    n1488 = global write "全局1.vi" "数据发送版本"(w1618) -> ()
    n1489 = local write "2011发送"(w1616) -> ()
  }
  n1490 = for {
    N: 1 -> [_]
    w1717 = "数据发送协议"
    w1724 = "线程一自主部署站点保存"
    w1740 = "数据发送通道" ("section")
    (unwired) path "C:/LabVIEW Project/builds/平台数据发送系统" ("Application Directory")
    w1791 = "" ("参数")
    w1752 = FALSE ("数据发送中断")
    w1762 = 0 ("数值")
    # "版本改动:增加了远程反控命令，和仪器端双向通讯，modbus TCP读写"
    # "ST参数选择"
    # "初始化"
    n1491 = property class="VI"() -> ("Panel"=w1795:refnum<vi>)  [unwired: 2 in, 2 out]
    n1492 = local write "核查数据上传"(w1752) -> ()
    n1493 = global write "全局 实时数据参数.vi" "参数"(w1791) -> ()
    n1494 = local write "心跳包"(w1752) -> ()
    n1495 = local write "查询数据发送"(w1752) -> ()
    n1496 = local write "实时小时数据上传"(w1752) -> ()
    n1497 = local write "系统状态改变"(w1752) -> ()
    n1498 = global write "全局 小时数据发送次数.vi" "小时数据发送次数"(w1762) -> ()
    n1499 = local write "重发数据"(w1752) -> ()
    n1500 = property class="Pnl"(reference=w1795) -> ("Panes[]"=w1794:refnum<vi>[])  [unwired: 1 in, 2 out]
    n1501 = global write "全局 实时数据参数.vi" "data"(string[][] [] ("data")) -> ()
    n1502 = property on="窗格" class="Pane"("Origin"=T11 {"Horizontal"=0, "Vertical"=0} ("原点")) -> ()  [unwired: 2 in, 2 out]
    n1503 = local write "空闲时间"(0.0 ("try")) -> ()
    n1504 = global write "全局1.vi" "枚举"(enum16{"返回请求应答", "上传数据", "返回执行结果"}."返回请求应答" ("枚举")) -> ()
    n1505 = global write "全局 实时数据参数.vi" "连接的字符串"(w1791) -> ()
    n1506 = call <vilib>:"Application Directory.vi"() -> ("Application Directory"=w1789:path)
    n1507 = for {
      tunnel: w1794 -> [w1806] mode=indexing
      tunnel: u32 15592941 ("窗格颜色") -> [w1807]
      n1508 = property class="Pane"(reference=w1806, "PaneColor"=w1807) -> ()  [unwired: 1 in, 2 out]
    }
    n1509 = Build Path(base path=w1789, name or relative path="data\\Set.ini" ("名称或相对路径")) -> (appended path=w1787:path)
    n1510 = call <vilib>:"Open Config Data.vi"("configuration file path"=w1787) -> ("error out"=w1785:errorcluster, "refnum"=w1786:T8)  [unwired: 8 in, 1 out]
    n1511 = call <vilib>:"Application Directory.vi"() -> ("Application Directory"=w1751:path)
    n1512 = call-poly <vilib>:"Read Key.vi"("section"=w1724, "error in (no error)"=w1785, "key"="站点名称", "refnum"=w1786) -> ("error out"=w1782:errorcluster, "value"=w1738:string, "refnum out"=w1783:T8)  [unwired: 4 in, 1 out]
    n1513 = call <vilib>:"Application Directory.vi"() -> ("Application Directory"=w1707:path)
    n1514 = call <vilib>:"Application Directory.vi"() -> ("Application Directory"=w1747:path)
    n1515 = call <vilib>:"Recursive File List.vi"("pattern"="*.exe", "Folder Path"=w1751) -> ("All Files in Dir"=w1760:path[])  [unwired: 5 in, 4 out]
    n1516 = Build Path(base path=w1707, name or relative path="data\\sys.ini" ("名称或相对路径")) -> (appended path=w1705:path)
    n1517 = local write "站点名称"(w1738) -> ()
    n1518 = Build Path(base path=w1747, name or relative path="data\\background.jpg" ("名称或相对路径")) -> (appended path=w1746:path)
    n1519 = call <vilib>:"Open Config Data.vi"("configuration file path"=w1705) -> ("error out"=w1711:errorcluster, "refnum"=w1710:T8)  [unwired: 8 in, 1 out]
    n1520 = Index Array(array=w1760) -> (element=w1759:path)  [unwired: 1 in]
    n1521 = Get Date/Time In Seconds() -> (seconds since 1Jan1904=w1799:timestamp)
    n1522 = call <vilib>:"Read JPEG File.vi"("path to JPEG file"=w1746) -> ("error out"=w1744:errorcluster, "image data"=w1745:T13)  [unwired: 8 in, 1 out]
    n1523 = vi-ref "断电保存全局.vi"() -> (w1709:refnum<vi>)
    n1524 = Format Date/Time String(time format string (%c)="%Y%m%d%H%M%S%3u" ("时间格式字符串(%c)"), seconds (now)=w1799) -> (date/time string=w1798:string)  [unwired: 1 in]
    n1525 = call-poly <vilib>:"Read Key.vi"("section"=w1724, "error in (no error)"=w1782, "key"="站点设备", "refnum"=w1783) -> ("error out"=w1779:errorcluster, "value"=w1737:string, "refnum out"=w1780:T8)  [unwired: 4 in, 1 out]
    n1526 = File/Directory Info(path=w1759) -> (last mod=w1758:timestamp)  [unwired: 1 in, 6 out]
    n1527 = call <vilib>:"FileVersionInfo.vi"("Application Path in"=w1759) -> ("error out"=w1743:errorcluster, "File Version Info"=w1755:string)  [unwired: 7 in, 2 out]
    n1528 = call <userlib>:"Read Panel from INI__ogtk.vi"("error in (no error)"=w1711, "VI ref"=w1709, "refnum"=w1710) -> ("error out"=w1704:errorcluster, "refnum out"=w1708:T8)  [unwired: 7 in]
    n1529 = property on="窗格" class="Pane"("BackgroundImage"=w1745) -> ()  [unwired: 2 in, 2 out]
    n1530 = Format Date/Time String(time format string (%c)="\n%Y%m%d%H%M" ("时间格式字符串(%c)"), seconds (now)=w1758) -> (date/time string=w1754:string)  [unwired: 1 in]
    n1531 = local write "站点设备"(w1737) -> ()
    n1532 = case shown="错误" w1704 {
      frame No Error {
      }
      frame Error {
        n1533 = global write "断电保存全局.vi" "判断数据反馈"(TRUE ("判断数据反馈")) -> ()
      }
    }
    n1534 = Search and Replace String(input string=w1798, search string="." ("搜索字符串")) -> (result string=w1796:string)  [unwired: 6 in, 3 out]
    n1535 = call <vilib>:"Close Config Data.vi"("error in (no error)"=w1704, "refnum"=w1708) -> ()  [unwired: 8 in, 2 out]
    n1536 = call-poly <vilib>:"Read Key.vi"("section"=w1724, "error in (no error)"=w1779, "key"="IP", "refnum"=w1780) -> ("error out"=w1776:errorcluster, "value"=w1736:string, "refnum out"=w1777:T8)  [unwired: 4 in, 1 out]
    n1537 = Concatenate Strings("V" ("字符串"), w1755, w1754) -> (→"软件版本":string)
    n1538 = local write "QN"(w1796) -> ()
    n1539 = call <vilib>:"Simple Error Handler.vi"("error in (no error)"=w1743) -> ()  [unwired: 4 in, 5 out]
    n1540 = call <vilib>:"Simple Error Handler.vi"("error in (no error)"=w1744) -> ()  [unwired: 4 in, 5 out]
    n1541 = local write "IP"(w1736) -> ()
    n1542 = call-poly <vilib>:"Read Key.vi"("section"=w1724, "error in (no error)"=w1776, "key"="PORT", "refnum"=w1777) -> ("error out"=w1772:errorcluster, "value"=w1735:string, "refnum out"=w1773:T8)  [unwired: 4 in, 1 out]
    n1543 = call <vilib>:"Application Directory.vi"() -> ("Application Directory"=w1750:path)
    n1544 = local write "PORT"(w1735) -> ()
    n1545 = call "查询启动项.vi"("启动文件路径"=w1750) -> ("包含启动项"=w1749:bool)  [unwired: 9 in, 1 out]
    n1546 = call-poly <vilib>:"Read Key.vi"("section"=w1724, "error in (no error)"=w1772, "key"="MN", "refnum"=w1773) -> ("error out"=w1731:errorcluster, "value"=w1734:string, "refnum out"=w1732:T8)  [unwired: 4 in, 1 out]
    n1547 = local write "MN"(w1734) -> ()
    n1548 = local write "开机启动"(w1749) -> ()
    n1549 = call-poly <vilib>:"Read Key.vi"("section"=w1724, "error in (no error)"=w1731, "key"="PW", "refnum"=w1732) -> ("error out"=w1729:errorcluster, "value"=w1733:string, "refnum out"=w1730:T8)  [unwired: 4 in, 1 out]
    n1550 = local write "PW"(w1733) -> ()
    n1551 = call-poly <vilib>:"Read Key.vi"("section"=w1724, "error in (no error)"=w1729, "key"="VISA", "refnum"=w1730) -> ("error out"=w1725:errorcluster, "value"=w1727:string, "refnum out"=w1726:T8)  [unwired: 4 in, 1 out]
    n1552 = local write "VISA resource name"(w1727) -> ()
    n1553 = call-poly <vilib>:"Read Key.vi"("section"=w1724, "error in (no error)"=w1725, "key"="BAUDRATE", "refnum"=w1726) -> ("error out"=w1720:errorcluster, "value"=w1722:i32, "refnum out"=w1721:T8)  [unwired: 4 in, 1 out]
    n1554 = local write "baud rate"(w1722) -> ()
    n1555 = call-poly <vilib>:"Read Key.vi"("section"="系统编码选择", "error in (no error)"=w1720, "key"="系统编码", "refnum"=w1721) -> ("error out"=w1766:errorcluster, "value"=w1768:string, "refnum out"=w1767:T8)  [unwired: 4 in, 1 out]
    n1556 = local write "系统编码选择框"(w1768) -> ()
    n1557 = call-poly <vilib>:"Read Key.vi"("section"="掉线时间存储", "error in (no error)"=w1766, "key"="掉线时间", "refnum"=w1767) -> ("error out"=w1741:errorcluster, "value"=w1763:string, "refnum out"=w1742:T8)  [unwired: 4 in, 1 out]
    n1558 = global write "全局 数据发送重叠.vi" "TCP掉线时间节点"(w1763) -> ()
    n1559 = local write "TCP掉线时间节点"(w1763) -> ()
    n1560 = call-poly <vilib>:"Read Key.vi"("section"=w1740, "error in (no error)"=w1741, "key"=w1740, "refnum"=w1742) -> ("error out"=w1718:errorcluster, "value"=w1739:i32, "refnum out"=w1719:T8)  [unwired: 4 in, 1 out]
    n1561 = local write "数据发送通道"(w1739) -> ()
    n1562 = call-poly <vilib>:"Read Key.vi"("section"=w1717, "error in (no error)"=w1718, "key"=w1717, "refnum"=w1719) -> ("error out"=w1715:errorcluster, "value"=w1713:i32, "found?"=w1714:bool, "refnum out"=w1716:T8)  [unwired: 4 in]
    n1563 = case shown="假" w1714 {
      tunnel: w1713 -> [_ w1805]
      tunnel: [1 ("value") w1805] -> w1712
      frame False {
      }
      frame True {
      }
    }
    n1564 = local write "数据发送协议"(w1712) -> ()
    n1565 = call <vilib>:"Close Config Data.vi"("error in (no error)"=w1715, "refnum"=w1716) -> ()  [unwired: 8 in, 2 out]
    "TCP服务端掉线计数" <- w1762
  }
  n1566 = property class="App"() -> ("App.Kind"=w31:T14)  [unwired: 2 in, 2 out]
  n1567 = case shown="\"Development System\", 默认" w31 {
    tunnel: [T15."Standard" ("状态") T15."Hidden" ("状态")] -> w3
    frame "Development System", Default {
    }
    frame "Run Time System" {
    }
  }
  n1568 = call "获取需发送的数据表.vi"() -> ("error out"=w42:errorcluster, "tables"=w51:string[])  [unwired: 10 in]
  n1569 = call <vilib>:"Clear Errors.vi"("error in (no error)"=w42) -> ()  [unwired: 5 in, 2 out]
  n1570 = call <vilib>:"Application Directory.vi"() -> ("Application Directory"=w25:path)
  n1571 = Build Path(base path=w25, name or relative path="data\\tubiao.ico" ("名称或相对路径")) -> (appended path=w15:path)
  n1572 = Insert Into Array(array=w51, index=0 ("索引"), new element="实时数据" ("新元素/子数组")) -> (w52:string[])
  n1573 = Current VI's Path() -> (path=w28:path)
  n1574 = Build Array(w15) -> (w20:path[])
  n1575 = Open VI Reference(vi path=w28) -> (vi reference=w29:refnum<vi>)  [unwired: 5 in, 1 out]
  n1576 = Array Size(array=w52) -> (size(s)=w49:i32)
  n1577 = invoke class="VI" method="FP.Open"(reference=w29, "Activate"=TRUE ("激活？"), "State"=w3) -> (error out=w30:errorcluster)  [unwired: 2 in, 4 out]
  n1578 = call <vilib>:"Constructor.vi"("error in"=w30, "IconFilePathList"=w20) -> ("error out"=w16:errorcluster, "NotifyIcon"=w24:refnum<class "NotifyIcon.lvclass">)  [unwired: 8 in]
  n1579 = Obtain Queue(name (unnamed)="STEP" ("名称（未命名）"), element data type=T6."初始化" ("枚举")) -> (queue out=w47:refnum<queue>)  [unwired: 3 in, 2 out]
  n1580 = for {
    shift-right: [w1814] -> w1
    shift-left: w16 -> [w1815]
    tunnel: string[] ["Open线程一", "-", "Exit线程一"] -> [w1813] mode=indexing
    tunnel: w23 -> [w1812] mode=indexing
    shift-right: [w1810] -> w2
    shift-left: w24 -> [w1811]
    # "2."
    n1581 = call <vilib>:"InsertMenuItem.vi"("error in"=w1815, "ItemTag"=w1812, "ItemName"=w1813, "NotifyIcon in"=w1811) -> ("error out"=w1814:errorcluster, "NotifyIcon out"=w1810:refnum<class "NotifyIcon.lvclass">)  [unwired: 6 in]
  }
  n1582 = Index Array(array=w23) -> (element=w22:string)  [unwired: 1 in]
  n1583 = Enqueue Element(queue=w47, element=T6."初始化" ("元素")) -> (queue out=w55:refnum<queue>)  [unwired: 2 in, 2 out]
  "主队列输出" <- w55
  n1584 = property class="NotifyIcon"(reference=w2, error in=w1, "Public:Visible"=TRUE ("Visible"), "Public:DefaultMenuItem"=w22, "Public:TipText"="平台发送系统线程一" ("TipText")) -> (reference out=w7:refnum<class "NotifyIcon.lvclass">, error out=w17:errorcluster, "Public:SelectedItemEvent"=w18:refnum<user-event>)
  n1585 = while {
    shift-right: [w1816] -> _
    shift-left: errorcluster {"status"=FALSE, "code"=0, "source"=""} ("error out") -> [w1828]
    shift-right: [w1825] -> _
    shift-left: _ -> [w1824]
    tunnel: w55 -> [w1827]
    tunnel: w52 -> [w1823]
    shift-right: [w1821] -> _
    shift-left: 0 ("索引") -> [w1822]
    tunnel: w49 -> [w1820]
    shift-right: [w1818] -> _
    shift-left: 0 ("索引") -> [w1819]
    stop <- FALSE stop-if-true
    n1586 = Wait (ms)(milliseconds to wait=u32 300 ("等待时间（毫秒）")) -> ()  [unwired: 1 out]
    n1587 = case shown="无错误" w1828 {
      selector: w1828 -> [w1846 w2600]
      tunnel: [w1829 w2603] -> w1816
      tunnel: w1827 -> [w1845 w2598]
      tunnel: [w1830 w2602] -> w1825
      tunnel: w1824 -> [w1842 w2602]
      tunnel: w1823 -> [w1841 _]
      tunnel: w1822 -> [w1836 w2601]
      tunnel: [w1839 w2601] -> w1821
      tunnel: w1820 -> [w1838 _]
      tunnel: w1819 -> [w1833 w2597]
      tunnel: [w1832 w2597] -> w1818
      frame No Error {
        n1588 = Less?(x=w1836, y=w1838) -> (x < y?=w1837:bool)
        n1589 = Dequeue Element(queue=w1845) -> (queue out=w1843:refnum<queue>, element=w1844:T6)  [unwired: 2 in, 2 out]
        "步骤" <- w1844
        n1590 = Select(t=w1836, s=w1837, f=0) -> (s? t:f=w1835:i32)
        n1591 = local read "元素"() -> (w1831:string)
        n1592 = Index Array(array=w1841, index=w1835) -> (element=→"元素":string)
        n1593 = case shown="\"读取数据\"" w1844 {
          tunnel: w1846 -> [w1853 _ w1878 w2018 w2512 w2594]
          tunnel: w1843 -> [w1849 w1867 w1873 w2033 w2510 w2592]
          tunnel: [w1853 w1855 w1878 w2016 w2509 w2594] -> w1829
          tunnel: [string[] [] ("待发送第一条数据") w1869 w1872 w2054 w2513 _] -> w1830
          tunnel: w1842 -> [_ w1869 _ w2054 w2513 w2593]
          tunnel: w1831 -> [_ _ _ _ _ w2587]
          tunnel: w1835 -> [w1850 w1866 w1877 w2055 w2514 w2583]
          tunnel: [w1850 w1866 w1876 w2055 w2514 w2584] -> w1839
          tunnel: w1833 -> [w1847 w1864 w1875 _ w2505 w2581]
          tunnel: [w1847 w1864 w1875 0 ("索引") w2508 w2581] -> w1832
          frame "初始化", Default {
            n1594 = Enqueue Element(queue=w1849, element=T6."打开连接" ("元素"), timeout in ms (-1)=1000 ("超时毫秒(-1)")) -> ()  [unwired: 1 in, 3 out]
          }
          frame "打开连接" {
            (unwired) "47.98.43.76"
            # "和时通数据接入平台端接收IP端口号，61.191.22.195:10003。"
            # "47.98.43.76:6666"
            n1595 = Enqueue Element(queue=w1867, element=T6."表格比对" ("元素"), timeout in ms (-1)=1000 ("超时毫秒(-1)")) -> ()  [unwired: 1 in, 3 out]
            n1596 = local read "数据发送通道"() -> (w1854:enum16{"TCP", "VISA"})
            n1597 = call "VISATCP组合选择发送.vi"("IP"="IP", "数据发送通道"=w1854, "命令"="open", "PORT"="PORT", "VISA resource name"="VISA resource name", "baud rate"="baud rate") -> ("错误输出"=w1855:errorcluster)  [unwired: 6 in, 3 out]
            n1598 = Unbundle By Name(w1855) -> ("status"=w1863:bool, "code"=→"1st Error to Convert":i32)
            n1599 = Not(x=w1863) -> (.not. x?=→"通信状态":bool)
          }
          frame "表格比对" {
            # "在发送数据完之后通过TCP掉线计数仍然大于1且列队中还有元素判定再次回到表格对比\n再在表格对比这里加上出列队（前提先一次把水样测试、核查等5个元素入列队）...........LOOP直到5种测量数据全部发送完毕"
            n1600 = disable-structure shown="禁用" {
              disable-tunnel: [w1880 _] -> _
              frame Disabled {
                n1601 = local read "TCP服务端掉线计数"() -> (w1882:i32)
                n1602 = Greater Or Equal?(x=w1882, y=1) -> (x >= y?=w1879:bool)
                n1603 = case shown="真" w1879 {
                  tunnel: [T6."读取数据" ("元素") w1884] -> w1880
                  frame False {
                  }
                  frame True {
                    n1604 = local read "重发数据"() -> (w1885:bool)
                    n1605 = Obtain Queue(name (unnamed)="重发掉线数据" ("名称（未命名）"), element data type=T16."水样测试") -> (queue out=w1891:refnum<queue>, error out=w1888:errorcluster)  [unwired: 3 in, 1 out]
                    n1606 = case shown="假" w1885 {
                      tunnel: w1891 -> [w1897 w1904]
                      tunnel: [w1895 w1904] -> w1889
                      tunnel: w1888 -> [w1894 w1903]
                      tunnel: [w1893 w1903] -> w1887
                      frame False {
                        n1607 = for {
                          N: 8 -> [_]
                          tunnel: w1897 -> [w1902]
                          tunnel: [w1900] -> w1895
                          tunnel: w1894 -> [w1899]
                          tunnel: [w1898] -> w1893
                          i -> [w1901]
                          n1608 = Enqueue Element(queue=w1902, element=w1901, error in (no error)=w1899) -> (queue out=w1900:refnum<queue>, error out=w1898:errorcluster)  [unwired: 1 in, 1 out]
                        }
                      }
                      frame True {
                      }
                    }
                    n1609 = Dequeue Element(queue=w1889, error in (no error)=w1887) -> (element=w1886:T16)  [unwired: 1 in, 3 out]
                    n1610 = case shown="\"加标回收\"" w1886 {
                      tunnel: [w1905 w1920 w1934 w1944 w1954 w1967 w1980 w1993] -> w1884
                      frame "水样测试", Default {
                        n1611 = flat-sequence {
                          tunnel: [w1913] -> w1905
                          frame #0 {
                            n1612 = global write "全局 小时数据发送次数.vi" "小时数据发送次数"(0 ("数值")) -> ()
                            n1613 = global write "全局 实时数据参数.vi" "实时数据参数"("水样测试") -> ()
                            n1614 = local write "table元素"("提取实时数据" ("新元素/子数组")) -> ()
                            n1615 = global write "全局1.vi" "枚举"(enum16{"返回请求应答", "上传数据", "返回执行结果"}."上传数据" ("枚举")) -> ()
                          }
                          frame #1 {
                            n1616 = call "从数据库获取数据通用可配置(子VI).vi"("table输入"="实时数据" ("新元素/子数组"), "列队名（唯一）"="adiao") -> ()  [unwired: 8 in, 2 out]
                          }
                          frame #2 {
                            # "数据处理整合"
                            n1617 = call "数据处理整合 (子VI).vi"("枚举"=enum16{"实时数据排序", "小时数据排序"}."实时数据排序") -> ("已排序的数组"=w1917:string[])  [unwired: 10 in]
                            n1618 = Array Size(array=w1917) -> (size(s)=w1916:i32)
                            n1619 = global write "全局 数据数组大小.vi" "数据数组大小"(w1916) -> ()
                            n1620 = Greater Than 0?(x=w1916) -> (x > 0?=w1915:bool)
                            n1621 = case shown="真" w1915 {
                              tunnel: [T6."表格比对" ("元素") T6."发送数据" ("元素")] -> w1913
                              frame False {
                              }
                              frame True {
                              }
                            }
                            "重发数据" <- TRUE ("重发数据中")
                          }
                        }
                      }
                      frame "小时数据" {
                        n1622 = flat-sequence {
                          tunnel: [w1928] -> w1920
                          frame #0 {
                            n1623 = local read "TCP掉线时间节点"() -> (w1922:string)
                            n1624 = call "当前时间格式显示 (子VI).vi"() -> ("当前时间格式显示"=w1921:string)  [unwired: 11 in]
                            n1625 = global write "全局 时间2.vi" "小时数据时间2"(w1921) -> ()
                            n1626 = global write "全局 水样时间.vi" "小时数据时间"(w1922) -> ()
                            n1627 = global write "全局 小时数据发送次数.vi" "小时数据发送次数"(0 ("数值")) -> ()
                            n1628 = local write "table元素"("小时数据" ("新元素/子数组")) -> ()
                            n1629 = global write "全局1.vi" "枚举"(enum16{"返回请求应答", "上传数据", "返回执行结果"}."返回请求应答" ("枚举")) -> ()
                          }
                          frame #1 {
                            n1630 = call "从数据库获取数据通用可配置(子VI).vi"("table输入"="小时数据" ("新元素/子数组"), "列队名（唯一）"="XS" ("名称（未命名）")) -> ()  [unwired: 8 in, 2 out]
                          }
                          frame #2 {
                            # "数据处理整合"
                            n1631 = call "数据处理整合 (子VI).vi"() -> ("已排序的数组"=w1931:string[])  [unwired: 11 in]
                            n1632 = Array Size(array=w1931) -> (size(s)=w1930:i32)
                            n1633 = global write "全局 数据数组大小.vi" "数据数组大小"(w1930) -> ()
                            n1634 = Greater Than 0?(x=w1930) -> (x > 0?=w1929:bool)
                            n1635 = case shown="真" w1929 {
                              tunnel: [T6."表格比对" ("元素") T6."发送数据" ("元素")] -> w1928
                              frame False {
                              }
                              frame True {
                              }
                            }
                          }
                        }
                      }
                      frame "日志信息" {
                        n1636 = flat-sequence {
                          tunnel: [w1938] -> w1934
                          frame #0 {
                            n1637 = global write "全局 小时数据发送次数.vi" "小时数据发送次数"(0 ("数值")) -> ()
                            n1638 = global write "全局1.vi" "枚举"(enum16{"返回请求应答", "上传数据", "返回执行结果"}."上传数据" ("枚举")) -> ()
                            n1639 = local write "table元素"("操作日志" ("新元素/子数组")) -> ()
                          }
                          frame #1 {
                            n1640 = call "获取操作日志 (子VI).vi"() -> ()  [unwired: 12 in]
                          }
                          frame #2 {
                            # "数据处理整合"
                            n1641 = call "数据处理整合 (子VI).vi"() -> ("已排序的数组"=w1941:string[])  [unwired: 11 in]
                            n1642 = Array Size(array=w1941) -> (size(s)=w1940:i32)
                            n1643 = global write "全局 数据数组大小.vi" "数据数组大小"(w1940) -> ()
                            n1644 = Greater Than 0?(x=w1940) -> (x > 0?=w1939:bool)
                            n1645 = case shown="假" w1939 {
                              tunnel: [T6."表格比对" ("元素") T6."发送数据" ("元素")] -> w1938
                              frame False {
                              }
                              frame True {
                              }
                            }
                          }
                        }
                      }
                      frame "报警信息" {
                        n1646 = flat-sequence {
                          tunnel: [w1948] -> w1944
                          frame #0 {
                            n1647 = global write "全局 小时数据发送次数.vi" "小时数据发送次数"(0 ("数值")) -> ()
                            n1648 = global write "全局1.vi" "枚举"(enum16{"返回请求应答", "上传数据", "返回执行结果"}."上传数据" ("枚举")) -> ()
                            n1649 = local write "table元素"("报警信息" ("新元素/子数组")) -> ()
                          }
                          frame #1 {
                            n1650 = call "获取报警信息 (子VI).vi"() -> ()  [unwired: 12 in]
                          }
                          frame #2 {
                            # "数据处理整合"
                            n1651 = call "数据处理整合 (子VI).vi"() -> ("已排序的数组"=w1951:string[])  [unwired: 11 in]
                            n1652 = Array Size(array=w1951) -> (size(s)=w1950:i32)
                            n1653 = Greater Than 0?(x=w1950) -> (x > 0?=w1949:bool)
                            n1654 = global write "全局 数据数组大小.vi" "数据数组大小"(w1950) -> ()
                            n1655 = case shown="假" w1949 {
                              tunnel: [T6."表格比对" ("元素") T6."发送数据" ("元素")] -> w1948
                              frame False {
                              }
                              frame True {
                              }
                            }
                          }
                        }
                      }
                      frame "零点核查" {
                        n1656 = flat-sequence {
                          tunnel: [w1961] -> w1954
                          frame #0 {
                            n1657 = global write "全局 小时数据发送次数.vi" "小时数据发送次数"(0 ("数值")) -> ()
                            n1658 = global write "全局 实时数据参数.vi" "实时数据参数"("空白测试") -> ()
                            n1659 = local write "table元素"("实时数据" ("新元素/子数组")) -> ()
                            n1660 = global write "全局1.vi" "枚举"(enum16{"返回请求应答", "上传数据", "返回执行结果"}."返回请求应答" ("枚举")) -> ()
                          }
                          frame #1 {
                            n1661 = call "从数据库获取数据通用可配置(子VI).vi"("table输入"="实时数据" ("新元素/子数组"), "列队名（唯一）"="bdiao") -> ()  [unwired: 8 in, 2 out]
                          }
                          frame #2 {
                            # "数据处理整合"
                            n1662 = call "数据处理整合 (子VI).vi"() -> ("已排序的数组"=w1964:string[])  [unwired: 11 in]
                            n1663 = Array Size(array=w1964) -> (size(s)=w1963:i32)
                            n1664 = global write "全局 数据数组大小.vi" "数据数组大小"(w1963) -> ()
                            n1665 = Greater Than 0?(x=w1963) -> (x > 0?=w1962:bool)
                            n1666 = case shown="假" w1962 {
                              tunnel: [T6."表格比对" ("元素") T6."发送数据" ("元素")] -> w1961
                              frame False {
                              }
                              frame True {
                              }
                            }
                          }
                        }
                      }
                      frame "标样核查" {
                        n1667 = flat-sequence {
                          tunnel: [w1974] -> w1967
                          frame #0 {
                            n1668 = global write "全局 小时数据发送次数.vi" "小时数据发送次数"(0 ("数值")) -> ()
                            n1669 = global write "全局 实时数据参数.vi" "实时数据参数"("跨度核查") -> ()
                            n1670 = global write "全局1.vi" "枚举"(enum16{"返回请求应答", "上传数据", "返回执行结果"}."返回请求应答" ("枚举")) -> ()
                            n1671 = local write "table元素"("实时数据" ("新元素/子数组")) -> ()
                          }
                          frame #1 {
                            n1672 = call "从数据库获取数据通用可配置(子VI).vi"("table输入"="实时数据" ("新元素/子数组"), "列队名（唯一）"="cdiao") -> ()  [unwired: 8 in, 2 out]
                          }
                          frame #2 {
                            # "数据处理整合"
                            n1673 = call "数据处理整合 (子VI).vi"() -> ("已排序的数组"=w1977:string[])  [unwired: 11 in]
                            n1674 = Array Size(array=w1977) -> (size(s)=w1976:i32)
                            n1675 = global write "全局 数据数组大小.vi" "数据数组大小"(w1976) -> ()
                            n1676 = Greater Than 0?(x=w1976) -> (x > 0?=w1975:bool)
                            n1677 = case shown="假" w1975 {
                              tunnel: [T6."表格比对" ("元素") T6."发送数据" ("元素")] -> w1974
                              frame False {
                              }
                              frame True {
                              }
                            }
                          }
                        }
                      }
                      frame "平行样" {
                        n1678 = flat-sequence {
                          tunnel: [w1987] -> w1980
                          frame #0 {
                            n1679 = global write "全局 小时数据发送次数.vi" "小时数据发送次数"(0 ("数值")) -> ()
                            n1680 = global write "全局 实时数据参数.vi" "实时数据参数"("平行样测试") -> ()
                            n1681 = local write "table元素"("提取实时数据" ("新元素/子数组")) -> ()
                            n1682 = global write "全局1.vi" "枚举"(enum16{"返回请求应答", "上传数据", "返回执行结果"}."上传数据" ("枚举")) -> ()
                          }
                          frame #1 {
                            n1683 = call "从数据库获取数据通用可配置(子VI).vi"("table输入"="实时数据" ("新元素/子数组"), "列队名（唯一）"="ddiao") -> ()  [unwired: 8 in, 2 out]
                          }
                          frame #2 {
                            # "数据处理整合"
                            n1684 = call "数据处理整合 (子VI).vi"() -> ("已排序的数组"=w1990:string[])  [unwired: 11 in]
                            n1685 = Array Size(array=w1990) -> (size(s)=w1989:i32)
                            n1686 = global write "全局 数据数组大小.vi" "数据数组大小"(w1989) -> ()
                            n1687 = Greater Than 0?(x=w1989) -> (x > 0?=w1988:bool)
                            n1688 = case shown="假" w1988 {
                              tunnel: [T6."表格比对" ("元素") T6."发送数据" ("元素")] -> w1987
                              frame False {
                              }
                              frame True {
                              }
                            }
                          }
                        }
                      }
                      frame "加标回收" {
                        n1689 = flat-sequence {
                          tunnel: [w2001] -> w1993
                          frame #0 {
                            n1690 = global write "全局 小时数据发送次数.vi" "小时数据发送次数"(0 ("数值")) -> ()
                            n1691 = global write "全局 实时数据参数.vi" "实时数据参数"("加标回收测试") -> ()
                            n1692 = global write "全局1.vi" "枚举"(enum16{"返回请求应答", "上传数据", "返回执行结果"}."上传数据" ("枚举")) -> ()
                            n1693 = local write "table元素"("实时数据" ("新元素/子数组")) -> ()
                          }
                          frame #1 {
                            n1694 = call "从数据库获取数据通用可配置(子VI).vi"("table输入"="加标回收" ("新元素/子数组"), "列队名（唯一）"="ediao") -> ()  [unwired: 8 in, 2 out]
                          }
                          frame #2 {
                            # "数据处理整合"
                            n1695 = call "加标回收数据处理整合 (子VI).vi"() -> ("已排序的数组"=w2000:string[])  [unwired: 11 in]
                            n1696 = Array Size(array=w2000) -> (size(s)=w2003:i32)
                            n1697 = global write "全局 数据数组大小.vi" "数据数组大小"(w2003) -> ()
                            n1698 = Greater Than 0?(x=w2003) -> (x > 0?=w2002:bool)
                            n1699 = case shown="假" w2002 {
                              tunnel: [T6."读取数据" ("元素") T6."发送数据" ("元素")] -> w2001
                              frame False {
                              }
                              frame True {
                              }
                            }
                          }
                        }
                      }
                    }
                  }
                }
              }
              frame Enabled {
              }
            }
            n1700 = disable-structure shown="启用" {
              disable-tunnel: [w2012 _] -> w1872
              frame Disabled {
                n1701 = call "数据表比对.vi"("查询元素输入"="氨氮" ("table输入 2"), "table输入"="实时数据") -> ("待发送第一条数据"=w2012:string[], "待发送数据"=w2006:string[][])  [unwired: 6 in, 2 out]
                n1702 = Empty Array?(array=w2006) -> (empty?=w2011:bool)
                n1703 = local read "心跳包"() -> (w2009:bool)
                n1704 = Not(x=w2011) -> (.not. x?=w2010:bool)
                n1705 = Or(x=w2010, y=w2009) -> ()  [unwired: 1 out]
              }
              frame Enabled {
              }
            }
            n1706 = case shown="假" FALSE {
              tunnel: w1877 -> [w2014 w2015]
              tunnel: [w2013 w2015] -> w1876
              frame False {
                n1707 = Increment(x=w2014) -> (x+1=w2013:i32)
              }
              frame True {
              }
            }
            n1708 = Enqueue Element(queue=w1873, element=T6."读取数据" ("元素"), timeout in ms (-1)=1000 ("超时毫秒(-1)")) -> ()  [unwired: 1 in, 3 out]
          }
          frame "读取数据" {
            w2029 = FALSE ("数据正在发送")
            # "设置测量时间间隔"
            # "1000设置超时时间和重发次数\n1011提取监测仪表时间\n1012设置监测仪表时间\n1014提取数采仪时间\n1015设置数采仪时间\n1061提取实时数据间隔\n1062设置实时数据间隔\n1072设置数采仪访问密码"
            # "6分钟掉线重连"
            n1709 = property on="TCP服务端掉线计数" class="DigNum (严格)"("Value"=0 ("TCP服务端掉线计数")) -> ()  [unwired: 2 in, 2 out]
            n1710 = global write "全局 数据发送重叠.vi" "掉线指示灯"(FALSE ("数据发送重叠")) -> ()
            n1711 = local write "重发数据"(w2029) -> ()
            n1712 = local write "查询数据发送"(w2029) -> ()
            n1713 = property on="实时数据发送时间间隔/min" class="DigNum (严格)"() -> ("Value"=w2041:u32)  [unwired: 2 in, 2 out]
            n1714 = global write "实时数据发送间隔全局.vi" "实时数据发送间隔"(w2041) -> ()
            n1715 = property on="设置超时时间/min" class="DigNum (严格)"() -> ("Value"=w2043:i32)  [unwired: 2 in, 2 out]
            n1716 = Multiply(x=w2043, y=10000) -> ()  [unwired: 1 out]
            n1717 = local read "数据发送通道"() -> (w2020:enum16{"TCP", "VISA"})
            n1718 = call "VISATCP组合选择发送.vi"("数据发送通道"=w2020, "命令"="read", "error in (no error)"=w2018) -> ("读取缓冲区"=w2017:string, "错误输出"=w2016:errorcluster)  [unwired: 9 in, 2 out]
            n1719 = Empty String/Path?(string/path=w2017) -> (empty?=w2026:bool)
            n1720 = case shown="假" w2026 {
              tunnel: w2017 -> [w2062 _]
              frame False {
                n1721 = call "数据记录.vi"("写入字段"=w2062) -> ("连接的字符串"=→"读取报文显示":string)  [unwired: 10 in]
                n1722 = global write "全局1.vi" "数据输出"(w2062) -> ()
                "数据输出" <- w2062
              }
              frame True {
              }
            }
            n1723 = control-ref of="数组 2"() -> (w2045:refnum<vi>)
            n1724 = control-ref of="数组"() -> (w2044:refnum<vi>)
            n1725 = call "读取数据处理 (子VI).vi"("Array输入"=w2045, "data out"=w2017, "reference"=w2044) -> ("数组"=→"数组":string[], "系统编码ST"=→"系统编码ST":string, "数组 2"=→"数组 2":string[], "命令编码CN"=w2034:string, "设备编码MN"=→"设备编码MN":string, "密码PW"=→"密码PW":string, "数据"=→"数据":string, "拆分包及应答Flag"=→"拆分包及应答Flag":string, "时间QN"=w2037:string)  [unwired: 4 in]
            "命令编码CN" <- w2034
            "时间QN" <- w2037
            n1726 = Search/Split String(string=w2037, search string/char (-)="QN=" ("搜索字符串/字符(-)")) -> (match + rest of string=w2035:string)  [unwired: 1 in, 2 out]
            n1727 = String Subset(string=w2035, offset (0)=3 ("偏移量(0)")) -> (substring=→"QN":string)  [unwired: 1 in]
            n1728 = local read "核查数据上传"() -> (w2024:bool)
            n1729 = local read "实时小时数据上传"() -> (w2025:bool)
            n1730 = Not(x=w2024) -> (.not. x?=w2022:bool)
            n1731 = Not(x=w2025) -> (.not. x?=w2023:bool)
            n1732 = And(x=w2023, y=w2022) -> (x .and. y?=w2021:bool)
            n1733 = case shown="真" w2021 {
              tunnel: w2034 -> [_ w2060]
              tunnel: ["" ("命令编码CN") w2057] -> w2027
              frame False {
              }
              frame True {
                n1734 = Search/Split String(string=w2060, search string/char (-)="CN=" ("搜索字符串/字符(-)")) -> (match + rest of string=w2058:string)  [unwired: 1 in, 2 out]
                n1735 = String Subset(string=w2058, offset (0)=3 ("偏移量(0)")) -> (substring=w2057:string)  [unwired: 1 in]
              }
            }
            n1736 = case shown="\"2082\"" w2027 {
              tunnel: w2033 -> [w2065 w2067 w2081 w2084 w2087 w2090 w2093 w2096 w2103 w2106 w2125 w2143 w2162 w2180 w2198 w2217 w2236 w2254 w2269 w2391 w2394 w2398 w2404 w2422 w2425 w2437 w2460 w2466]
              tunnel: [w2065 w2067 w2081 w2084 w2087 w2090 w2093 w2096 w2103 w2106 w2125 w2143 w2162 w2180 w2198 w2217 w2236 w2254 w2269 w2391 w2394 w2398 w2404 w2422 w2425 w2437 w2460 w2466] -> w2031
              tunnel: [T6."读取数据" ("元素") T6."发送数据" ("元素") T6."发送数据" ("元素") T6."发送数据" ("元素") T6."发送数据" ("元素") T6."发送数据" ("元素") T6."发送数据" ("元素") T6."发送数据" ("元素") T6."发送数据" ("元素") w2105 w2124 w2142 w2161 w2179 w2197 w2216 w2235 w2253 w2268 T6."发送数据" ("元素") w2393 w2397 T6."发送数据" ("元素") T6."发送数据" ("元素") T6."发送数据" ("元素") T6."发送数据" ("元素") T6."发送数据" ("元素") T6."发送数据" ("元素")] -> w2030
              tunnel: w2027 -> [_ _ _ _ _ _ _ _ _ _ _ _ _ _ _ _ _ _ _ _ _ _ _ _ _ _ _ w2464]
              frame "", Default {
              }
              frame "1000" {
                # "发回给平台"
                # "反控指令"
                # "3042~3086"
                # "1000"
                n1737 = property on="数据" class="Str"() -> ("Value"=w2073:string)  [unwired: 2 in, 2 out]
                n1738 = String Subset(string=w2073, offset (0)=9 ("偏移量(0)"), length (rest)=1 ("长度（剩余）")) -> (substring=w2070:string)
                n1739 = Decimal String To Number(string=w2070) -> (number=→"设置超时时间/min":i32)  [unwired: 2 in, 1 out]
                n1740 = local write "table元素"("反控命令" ("新元素/子数组")) -> ()
              }
              frame "1011" {
                # "1011"
                n1741 = local read "数据"() -> (w2079:string)
                n1742 = Search/Split String(string=w2079, search string/char (-)="PolId=" ("搜索字符串/字符(-)")) -> (match + rest of string=w2077:string)  [unwired: 1 in, 2 out]
                n1743 = String Subset(string=w2077, offset (0)=6 ("偏移量(0)"), length (rest)=6 ("长度（剩余）")) -> (substring=w2074:string)
                n1744 = global write "全局 提取仪器参数.vi" "仪器编码"(w2074) -> ()
                n1745 = local write "table元素"("提取监测仪表时间") -> ()
              }
              frame "1012" {
                # "设置监测仪表时间"
                n1746 = local write "table元素"("反控命令" ("新元素/子数组")) -> ()
              }
              frame "1014" {
                # "1014"
                n1747 = local write "table元素"("提取数采仪时间") -> ()
              }
              frame "1015" {
                # "设置数采仪时间"
                n1748 = local write "table元素"("反控命令" ("新元素/子数组")) -> ()
              }
              frame "1061" {
                # "1061"
                n1749 = local write "table元素"("提取实时数据间隔") -> ()
              }
              frame "1062" {
                # "发回给平台"
                # "反控指令"
                # "3042~3086"
                # "设置数据发送时间间隔"
                # "1062"
                n1750 = property on="数据" class="Str"() -> ("Value"=w2101:string)  [unwired: 2 in, 2 out]
                n1751 = String Subset(string=w2101, offset (0)=12 ("偏移量(0)")) -> (substring=w2099:string)  [unwired: 1 in]
                n1752 = Decimal String To Number(string=w2099) -> (number=w2098:i32)  [unwired: 2 in, 1 out]
                n1753 = property on="实时数据发送时间间隔/min" class="DigNum (严格)"("Value"=w2098) -> ()  [unwired: 2 in, 2 out]
                n1754 = local write "table元素"("反控命令" ("新元素/子数组")) -> ()
              }
              frame "1072" {
                # "设置数采仪密码"
                n1755 = local write "table元素"("反控命令" ("新元素/子数组")) -> ()
              }
              frame "2011" {
                w2111 = 0 ("数值")
                # "2011提取实时数据"
                n1756 = local read "数据"() -> (w2112:string)
                n1757 = String Subset(string=w2112, offset (0)=10 ("偏移量(0)"), length (rest)=14 ("长度（剩余）")) -> (substring=w2108:string)
                n1758 = String Subset(string=w2112, offset (0)=33 ("偏移量(0)"), length (rest)=14 ("长度（剩余）")) -> (substring=w2110:string)
                n1759 = call "格式时间字符串.vi"("字符串"=w2108) -> ("连接的字符串"=w2107:string)  [unwired: 10 in]
                n1760 = call "格式时间字符串.vi"("字符串"=w2110) -> ("连接的字符串"=w2109:string)  [unwired: 10 in]
                n1761 = global write "全局 小时数据发送次数.vi" "小时数据发送次数"(w2111) -> ()
                n1762 = global write "全局1.vi" "枚举"(w2111) -> ()
                n1763 = global write "起始时间.vi" "结束时间"(w2109) -> ()
                n1764 = global write "起始时间.vi" "起始时间"(w2107) -> ()
                n1765 = flat-sequence {
                  tunnel: [T6."发送数据" ("元素")] -> w2105
                  frame #0 {
                    w2117 = "提取实时数据" ("新元素/子数组")
                    n1766 = global write "全局 实时数据参数.vi" "实时数据参数"("水样测试") -> ()
                    n1767 = call "从数据库获取数据通用可配置(子VI).vi"("table输入"=w2117, "列队名（唯一）"=w2117) -> ()  [unwired: 8 in, 2 out]
                  }
                  frame #1 {
                    # "数据处理整合"
                    n1768 = local write "table元素"("提取实时数据" ("新元素/子数组")) -> ()
                    n1769 = call "数据处理整合 (子VI).vi"("枚举"=enum16{"实时数据排序", "小时数据排序"}."实时数据排序") -> ("已排序的数组"=w2120:string[])  [unwired: 10 in]
                    n1770 = Array Size(array=w2120) -> (size(s)=w2121:i32)
                    n1771 = global write "全局 数据数组大小.vi" "数据数组大小"(w2121) -> ()
                  }
                  frame #2 {
                  }
                }
              }
              frame "2061" {
                w2126 = 0 ("数值")
                n1772 = flat-sequence {
                  tunnel: [T6."发送数据" ("元素")] -> w2124
                  frame #0 {
                    # "格式时间"
                    # "2061、提取小时数据"
                    n1773 = local read "数据"() -> (w2133:string)
                    n1774 = String Subset(string=w2133, offset (0)=33 ("偏移量(0)"), length (rest)=14 ("长度（剩余）")) -> (substring=w2128:string)
                    n1775 = String Subset(string=w2133, offset (0)=10 ("偏移量(0)"), length (rest)=14 ("长度（剩余）")) -> (substring=w2129:string)
                    n1776 = call "格式时间字符串.vi"("字符串"=w2129) -> ("连接的字符串"=w2130:string)  [unwired: 10 in]
                    n1777 = call "格式时间字符串.vi"("字符串"=w2128) -> ("连接的字符串"=w2127:string)  [unwired: 10 in]
                    n1778 = global write "全局 水样时间.vi" "小时数据时间"(w2130) -> ()
                    n1779 = global write "全局 时间2.vi" "小时数据时间2"(w2127) -> ()
                  }
                  frame #1 {
                    w2136 = "小时数据" ("名称（未命名）")
                    # "提取COD、氨氮、多参数、总磷、总氮数据"
                    n1780 = call "从数据库获取数据通用可配置(子VI).vi"("table输入"=w2136, "列队名（唯一）"=w2136) -> ()  [unwired: 8 in, 2 out]
                  }
                  frame #2 {
                    # "数据处理整合"
                    n1781 = call "数据处理整合 (子VI).vi"("枚举"=enum16{"实时数据排序", "小时数据排序"}."小时数据排序") -> ("已排序的数组"=w2139:string[])  [unwired: 10 in]
                    n1782 = local write "table元素"("提取小时数据" ("新元素/子数组")) -> ()
                    n1783 = Array Size(array=w2139) -> (size(s)=w2138:i32)
                    n1784 = global write "全局 数据数组大小.vi" "数据数组大小"(w2138) -> ()
                  }
                  frame #3 {
                  }
                }
                n1785 = global write "全局 小时数据发送次数.vi" "小时数据发送次数"(w2126) -> ()
                n1786 = global write "全局1.vi" "枚举"(w2126) -> ()
              }
              frame "2062" {
                w2144 = 0 ("数值")
                n1787 = flat-sequence {
                  tunnel: [T6."发送数据" ("元素")] -> w2142
                  frame #0 {
                    # "格式时间"
                    # "2062、提取标样核查数据"
                    n1788 = local read "数据"() -> (w2151:string)
                    n1789 = String Subset(string=w2151, offset (0)=33 ("偏移量(0)"), length (rest)=14 ("长度（剩余）")) -> (substring=w2146:string)
                    n1790 = String Subset(string=w2151, offset (0)=10 ("偏移量(0)"), length (rest)=14 ("长度（剩余）")) -> (substring=w2147:string)
                    n1791 = call "格式时间字符串.vi"("字符串"=w2147) -> ("连接的字符串"=w2148:string)  [unwired: 10 in]
                    n1792 = call "格式时间字符串.vi"("字符串"=w2146) -> ("连接的字符串"=w2145:string)  [unwired: 10 in]
                    n1793 = global write "全局 水样时间.vi" "时间"(w2148) -> ()
                    n1794 = global write "全局 时间2.vi" "时间2"(w2145) -> ()
                  }
                  frame #1 {
                    # "提取COD、氨氮、多参数、总磷、总氮数据"
                    n1795 = call "从数据库获取数据通用可配置(子VI).vi"("table输入"="标样核查" ("新元素/子数组"), "列队名（唯一）"="核查数据" ("新元素/子数组")) -> ()  [unwired: 8 in, 2 out]
                  }
                  frame #2 {
                    # "数据处理整合"
                    n1796 = local write "table元素"("核查数据" ("新元素/子数组")) -> ()
                    n1797 = call "数据处理整合 (子VI).vi"("枚举"=enum16{"实时数据排序", "小时数据排序"}."实时数据排序") -> ("已排序的数组"=w2157:string[])  [unwired: 10 in]
                    n1798 = Array Size(array=w2157) -> (size(s)=w2158:i32)
                    n1799 = global write "全局 数据数组大小.vi" "数据数组大小"(w2158) -> ()
                  }
                  frame #3 {
                  }
                }
                n1800 = global write "全局 小时数据发送次数.vi" "小时数据发送次数"(w2144) -> ()
                n1801 = global write "全局1.vi" "枚举"(w2144) -> ()
              }
              frame "2063" {
                w2167 = 0 ("数值")
                # "2063提取加标回收数据"
                n1802 = local read "数据"() -> (w2168:string)
                n1803 = String Subset(string=w2168, offset (0)=10 ("偏移量(0)"), length (rest)=14 ("长度（剩余）")) -> (substring=w2164:string)
                n1804 = String Subset(string=w2168, offset (0)=33 ("偏移量(0)"), length (rest)=14 ("长度（剩余）")) -> (substring=w2166:string)
                n1805 = call "格式时间字符串.vi"("字符串"=w2164) -> ("连接的字符串"=w2163:string)  [unwired: 10 in]
                n1806 = call "格式时间字符串.vi"("字符串"=w2166) -> ("连接的字符串"=w2165:string)  [unwired: 10 in]
                n1807 = global write "全局 小时数据发送次数.vi" "小时数据发送次数"(w2167) -> ()
                n1808 = global write "全局1.vi" "枚举"(w2167) -> ()
                n1809 = global write "起始时间.vi" "结束时间"(w2165) -> ()
                n1810 = global write "起始时间.vi" "起始时间"(w2163) -> ()
                n1811 = flat-sequence {
                  tunnel: [T6."发送数据" ("元素")] -> w2161
                  frame #0 {
                    w2173 = "提取加标回收" ("新元素/子数组")
                    n1812 = call "从数据库获取数据通用可配置(子VI).vi"("table输入"=w2173, "列队名（唯一）"=w2173) -> ()  [unwired: 8 in, 2 out]
                  }
                  frame #1 {
                    n1813 = local write "table元素"("提取加标回收" ("新元素/子数组")) -> ()
                    n1814 = call "加标回收数据处理整合 (子VI).vi"("枚举"=enum16{"实时数据排序", "小时数据排序"}."实时数据排序") -> ("已排序的数组"=w2174:string[])  [unwired: 10 in]
                    n1815 = Array Size(array=w2174) -> (size(s)=w2176:i32)
                    n1816 = global write "全局 数据数组大小.vi" "数据数组大小"(w2176) -> ()
                  }
                  frame #2 {
                  }
                }
              }
              frame "2064" {
                w2185 = 0 ("数值")
                # "2064提取平行样数据"
                n1817 = local read "数据"() -> (w2186:string)
                n1818 = String Subset(string=w2186, offset (0)=10 ("偏移量(0)"), length (rest)=14 ("长度（剩余）")) -> (substring=w2182:string)
                n1819 = String Subset(string=w2186, offset (0)=33 ("偏移量(0)"), length (rest)=14 ("长度（剩余）")) -> (substring=w2184:string)
                n1820 = call "格式时间字符串.vi"("字符串"=w2182) -> ("连接的字符串"=w2181:string)  [unwired: 10 in]
                n1821 = call "格式时间字符串.vi"("字符串"=w2184) -> ("连接的字符串"=w2183:string)  [unwired: 10 in]
                n1822 = global write "全局 小时数据发送次数.vi" "小时数据发送次数"(w2185) -> ()
                n1823 = global write "全局1.vi" "枚举"(w2185) -> ()
                n1824 = global write "起始时间.vi" "结束时间"(w2183) -> ()
                n1825 = global write "起始时间.vi" "起始时间"(w2181) -> ()
                n1826 = flat-sequence {
                  tunnel: [T6."发送数据" ("元素")] -> w2179
                  frame #0 {
                    w2191 = "提取平行样" ("新元素/子数组")
                    n1827 = call "从数据库获取数据通用可配置(子VI).vi"("table输入"=w2191, "列队名（唯一）"=w2191) -> ()  [unwired: 8 in, 2 out]
                  }
                  frame #1 {
                    n1828 = call "数据处理整合 (子VI).vi"("枚举"=enum16{"实时数据排序", "小时数据排序"}."实时数据排序") -> ("已排序的数组"=w2194:string[])  [unwired: 10 in]
                    n1829 = Array Size(array=w2194) -> (size(s)=w2193:i32)
                    n1830 = local write "table元素"("提取平行样" ("新元素/子数组")) -> ()
                    n1831 = global write "全局 数据数组大小.vi" "数据数组大小"(w2193) -> ()
                  }
                  frame #2 {
                  }
                }
              }
              frame "2065" {
                w2199 = 0 ("数值")
                n1832 = flat-sequence {
                  tunnel: [T6."发送数据" ("元素")] -> w2197
                  frame #0 {
                    # "格式时间"
                    # "2065、提取零点核查数据"
                    n1833 = local read "数据"() -> (w2208:string)
                    n1834 = global write "全局 实时数据参数.vi" "实时数据参数"("空白测试" ("新元素/子数组")) -> ()
                    n1835 = local write "table元素"("空白测试" ("新元素/子数组")) -> ()
                    n1836 = String Subset(string=w2208, offset (0)=33 ("偏移量(0)"), length (rest)=14 ("长度（剩余）")) -> (substring=w2203:string)
                    n1837 = String Subset(string=w2208, offset (0)=10 ("偏移量(0)"), length (rest)=14 ("长度（剩余）")) -> (substring=w2204:string)
                    n1838 = call "格式时间字符串.vi"("字符串"=w2204) -> ("连接的字符串"=w2205:string)  [unwired: 10 in]
                    n1839 = call "格式时间字符串.vi"("字符串"=w2203) -> ("连接的字符串"=w2202:string)  [unwired: 10 in]
                    n1840 = global write "全局 水样时间.vi" "时间"(w2205) -> ()
                    n1841 = global write "全局 时间2.vi" "时间2"(w2202) -> ()
                  }
                  frame #1 {
                    w2211 = "空白测试" ("新元素/子数组")
                    n1842 = call "从数据库获取数据通用可配置(子VI).vi"("table输入"=w2211, "列队名（唯一）"=w2211) -> ()  [unwired: 8 in, 2 out]
                  }
                  frame #2 {
                    # "数据处理整合"
                    n1843 = call "数据处理整合 (子VI).vi"("枚举"=enum16{"实时数据排序", "小时数据排序"}."实时数据排序") -> ("已排序的数组"=w2213:string[])  [unwired: 10 in]
                    n1844 = Array Size(array=w2213) -> (size(s)=w2214:i32)
                    n1845 = global write "全局 数据数组大小.vi" "数据数组大小"(w2214) -> ()
                  }
                  frame #3 {
                  }
                }
                n1846 = global write "全局 小时数据发送次数.vi" "小时数据发送次数"(w2199) -> ()
                n1847 = global write "全局1.vi" "枚举"(w2199) -> ()
              }
              frame "2066" {
                w2218 = 0 ("数值")
                n1848 = flat-sequence {
                  tunnel: [T6."发送数据" ("元素")] -> w2216
                  frame #0 {
                    # "格式时间"
                    # "2066、提取跨度核查数据"
                    n1849 = local read "数据"() -> (w2227:string)
                    n1850 = String Subset(string=w2227, offset (0)=33 ("偏移量(0)"), length (rest)=14 ("长度（剩余）")) -> (substring=w2222:string)
                    n1851 = String Subset(string=w2227, offset (0)=10 ("偏移量(0)"), length (rest)=14 ("长度（剩余）")) -> (substring=w2223:string)
                    n1852 = global write "全局 实时数据参数.vi" "实时数据参数"("跨度核查" ("新元素/子数组")) -> ()
                    n1853 = local write "table元素"("跨度核查" ("新元素/子数组")) -> ()
                    n1854 = call "格式时间字符串.vi"("字符串"=w2223) -> ("连接的字符串"=w2224:string)  [unwired: 10 in]
                    n1855 = call "格式时间字符串.vi"("字符串"=w2222) -> ("连接的字符串"=w2221:string)  [unwired: 10 in]
                    n1856 = global write "全局 水样时间.vi" "时间"(w2224) -> ()
                    n1857 = global write "全局 时间2.vi" "时间2"(w2221) -> ()
                  }
                  frame #1 {
                    w2230 = "跨度核查" ("新元素/子数组")
                    (unwired) "跨度核查" ("名称（未命名）")
                    # "提取COD、氨氮、多参数、总磷、总氮数据"
                    n1858 = call "从数据库获取数据通用可配置(子VI).vi"("table输入"=w2230, "列队名（唯一）"=w2230) -> ()  [unwired: 8 in, 2 out]
                  }
                  frame #2 {
                    # "数据处理整合"
                    n1859 = call "数据处理整合 (子VI).vi"("枚举"=enum16{"实时数据排序", "小时数据排序"}."实时数据排序") -> ("已排序的数组"=w2233:string[])  [unwired: 10 in]
                    n1860 = Array Size(array=w2233) -> (size(s)=w2232:i32)
                    n1861 = global write "全局 数据数组大小.vi" "数据数组大小"(w2232) -> ()
                  }
                  frame #3 {
                  }
                }
                n1862 = global write "全局 小时数据发送次数.vi" "小时数据发送次数"(w2218) -> ()
                n1863 = global write "全局1.vi" "枚举"(w2218) -> ()
              }
              frame "2082" {
                w2241 = 0 ("数值")
                # "2082提取集成干预"
                n1864 = local read "数据"() -> (w2242:string)
                n1865 = String Subset(string=w2242, offset (0)=10 ("偏移量(0)"), length (rest)=14 ("长度（剩余）")) -> (substring=w2238:string)
                n1866 = String Subset(string=w2242, offset (0)=33 ("偏移量(0)"), length (rest)=14 ("长度（剩余）")) -> (substring=w2240:string)
                n1867 = call "格式时间字符串.vi"("字符串"=w2238) -> ("连接的字符串"=w2237:string)  [unwired: 10 in]
                n1868 = call "格式时间字符串.vi"("字符串"=w2240) -> ("连接的字符串"=w2239:string)  [unwired: 10 in]
                n1869 = global write "全局 小时数据发送次数.vi" "小时数据发送次数"(w2241) -> ()
                n1870 = global write "全局1.vi" "枚举"(w2241) -> ()
                n1871 = global write "起始时间.vi" "结束时间"(w2239) -> ()
                n1872 = global write "起始时间.vi" "起始时间"(w2237) -> ()
                n1873 = flat-sequence {
                  tunnel: [T6."发送数据" ("元素")] -> w2235
                  frame #0 {
                    w2247 = "提取集成干预" ("新元素/子数组")
                    n1874 = call "从数据库获取数据通用可配置(子VI).vi"("table输入"=w2247, "列队名（唯一）"=w2247) -> ()  [unwired: 8 in, 2 out]
                  }
                  frame #1 {
                    n1875 = call "数据处理整合 (子VI).vi"("枚举"=enum16{"实时数据排序", "小时数据排序"}."实时数据排序") -> ("已排序的数组"=w2250:string[])  [unwired: 10 in]
                    n1876 = Array Size(array=w2250) -> (size(s)=w2249:i32)
                    n1877 = local write "table元素"("提取集成干预" ("新元素/子数组")) -> ()
                    n1878 = global write "全局 数据数组大小.vi" "数据数组大小"(w2249) -> ()
                  }
                  frame #2 {
                  }
                }
              }
              frame "3015" {
                n1879 = flat-sequence {
                  tunnel: [T6."发送数据" ("元素")] -> w2253
                  frame #0 {
                    # "发命令给中控"
                    # "发回给平台"
                    # "3015、手动远程留样"
                    n1880 = local write "table元素"("超标留样返回" ("新元素/子数组")) -> ()
                    n1881 = Insert Into Array(array=u16[] [] ("holding register values"), index=0 ("索引"), new element=u16 1 ("新元素/子数组")) -> (w2257:u16[])
                    n1882 = call "Modbus Master.vi"("Unit ID"=u8 1, "读取写入选择"="写入", "holding register values"=w2257, "starting address"=u16 10) -> ()  [unwired: 6 in, 2 out]
                  }
                  frame #1 {
                  }
                }
              }
              frame "3020" {
                n1883 = flat-sequence {
                  tunnel: [w2273] -> w2267
                  tunnel: [w2274] -> w2266
                  tunnel: [w2272] -> w2265
                  tunnel: [w2270] -> w2264
                  tunnel: w2267 -> [w2323]
                  tunnel: w2266 -> [w2322]
                  tunnel: w2265 -> [w2321]
                  tunnel: w2264 -> [w2320]
                  tunnel: [T6."发送数据" ("元素")] -> w2268
                  frame #0 {
                    w2293 = 0 ("数值")
                    # "3020、提取日志、报警，仪器参数"
                    n1884 = local read "数据"() -> (w2294:string)
                    n1885 = Search/Split String(string=w2294, search string/char (-)="BeginTime=" ("搜索字符串")) -> (match + rest of string=w2292:string)  [unwired: 1 in, 2 out]
                    n1886 = local read "数据"() -> (w2278:string)
                    n1887 = case shown="\"\"" w2292 {
                      tunnel: ["1904/01/01 00:00:00" w2317] -> w2296
                      tunnel: w2292 -> [_ w2311]
                      tunnel: [w2304 w2312] -> w2291
                      frame "" {
                        # "时间"
                        n1888 = Get Date/Time In Seconds() -> (seconds since 1Jan1904=w2305:timestamp)
                        n1889 = Format Date/Time String(time format string (%c)="%Y%m%d%H%M%S%3u" ("时间格式字符串(%c)"), seconds (now)=w2305) -> (date/time string=w2309:string)  [unwired: 1 in]
                        n1890 = Search and Replace String(input string=w2309, search string="." ("搜索字符串")) -> (result string=w2308:string)  [unwired: 6 in, 3 out]
                        n1891 = call "格式时间字符串.vi"("字符串"=w2308) -> ("连接的字符串"=w2304:string)  [unwired: 10 in]
                      }
                      frame "真", Default {
                        # "格式时间"
                        n1892 = String Subset(string=w2311, offset (0)=33 ("偏移量(0)"), length (rest)=14 ("长度（剩余）")) -> (substring=w2315:string)
                        n1893 = String Subset(string=w2311, offset (0)=10 ("偏移量(0)"), length (rest)=14 ("长度（剩余）")) -> (substring=w2316:string)
                        n1894 = call "格式时间字符串.vi"("字符串"=w2315) -> ("连接的字符串"=w2312:string)  [unwired: 10 in]
                        n1895 = call "格式时间字符串.vi"("字符串"=w2316) -> ("连接的字符串"=w2317:string)  [unwired: 10 in]
                      }
                    }
                    n1896 = call "日志报警参数选择 (子VI).vi"("String输入"=w2278) -> ("输出簇"=w2277:T18)  [unwired: 9 in, 1 out]
                    n1897 = Unbundle By Name(w2277) -> ("高锰酸盐"=w2285:string, "化学需氧量"=w2286:string, "氨氮"=w2287:string, "总磷"=w2288:string, "总氮"=w2289:string, "数采仪"=w2290:string, "高锰酸盐"=w2279:bool, "化学需氧量"=w2280:bool, "氨氮"=w2281:bool, "总磷"=w2282:bool, "总氮"=w2283:bool, "数采仪"=w2284:bool)
                    n1898 = Build Array(w2285, w2286, w2287, w2288, w2289, w2290) -> (w2272:string[])
                    n1899 = global write "全局 时间2.vi" "时间2"(w2291) -> ()
                    n1900 = Build Array(w2279, w2280, w2281, w2282, w2283, w2284) -> (w2271:bool[])
                    n1901 = global write "全局 水样时间.vi" "时间"(w2296) -> ()
                    n1902 = Or Array Elements(Boolean array=w2271) -> (logical OR=w2270:bool)
                    n1903 = global write "全局 小时数据发送次数.vi" "小时数据发送次数"(w2293) -> ()
                    n1904 = Obtain Queue(name (unnamed)="操作日志报警信息" ("名称（未命名）"), element data type=T17."CODMn") -> (queue out=w2273:refnum<queue>, error out=w2274:errorcluster)  [unwired: 3 in, 1 out]
                    n1905 = case shown="假" w2270 {
                      tunnel: w2273 -> [_ w2298]
                      tunnel: w2271 -> [_ w2297]
                      frame False {
                      }
                      frame True {
                        n1906 = for {
                          tunnel: w2297 -> [w2300] mode=indexing
                          tunnel: w2298 -> [w2299]
                          i -> [w2301]
                          n1907 = case shown="真" w2300 {
                            tunnel: w2301 -> [_ w2303]
                            tunnel: w2299 -> [_ w2302]
                            frame False {
                            }
                            frame True {
                              n1908 = call "提取日志报警参数入列队 (子VI).vi"("枚举"=w2303, "queue in"=w2302) -> ()  [unwired: 10 in]
                            }
                          }
                        }
                      }
                    }
                    n1909 = global write "全局1.vi" "枚举"(w2293) -> ()
                  }
                  frame #1 {
                    # "按需求提取COD、氨氮、总磷、总氮日志"
                    # "按需求提取COD、氨氮、总磷、总氮日志"
                    n1910 = case shown="真" w2320 {
                      tunnel: w2322 -> [_ w2326]
                      tunnel: w2323 -> [_ w2325]
                      tunnel: w2321 -> [_ w2324]
                      frame False {
                      }
                      frame True {
                        n1911 = while {
                          shift-right: [w2340] -> _
                          shift-left: w2325 -> [w2341]
                          tunnel: w2326 -> [w2339]
                          tunnel: w2324 -> [w2334]
                          stop <- w2336 stop-if-true
                          n1912 = Dequeue Element(queue=w2341, error in (no error)=w2339) -> (queue out=w2338:refnum<queue>, element=w2333:T17)  [unwired: 1 in, 2 out]
                          n1913 = Index Array(array=w2334) -> (element #1=w2332:string, element #2=w2331:string, element #3=w2330:string, element #4=w2329:string, element #5=w2328:string, element #6=w2327:string)  [unwired: 6 in]
                          n1914 = case shown="\"CODCr\"" w2333 {
                            tunnel: w2338 -> [w2346 _ w2355 w2360 w2364 w2369]
                            tunnel: [w2346 _ w2355 w2360 w2364 w2369] -> w2340
                            tunnel: w2332 -> [w2343 _ _ _ _ _]
                            tunnel: w2331 -> [_ w2348 _ _ _ _]
                            tunnel: w2330 -> [_ _ w2352 _ _ _]
                            tunnel: w2329 -> [_ _ _ w2357 _ _]
                            tunnel: w2328 -> [_ _ _ _ w2362 _]
                            tunnel: w2327 -> [_ _ _ _ _ w2366]
                            frame "CODMn" {
                              w2342 = string[][] [] ("氨氮")
                              n1915 = call "数据表比对.vi"("仪器日志参数"="CODMn" ("元素"), "table输入"=w2343) -> ("待发送数据"=w2344:string[][])  [unwired: 6 in, 3 out]
                              n1916 = global write "全局 所有参数.vi" "CODMn"(w2344) -> ()
                              n1917 = global write "全局 所有参数.vi" "总氮"(w2342) -> ()
                              n1918 = global write "全局 所有参数.vi" "CODCr"(w2342) -> ()
                              n1919 = global write "全局 所有参数.vi" "总磷"(w2342) -> ()
                              n1920 = global write "全局 所有参数.vi" "氨氮"(w2342) -> ()
                            }
                            frame "CODCr" {
                              w2347 = string[][] [] ("氨氮")
                              n1921 = call "数据表比对.vi"("仪器日志参数"="CODCr" ("元素"), "table输入"=w2348) -> ("待发送数据"=w2349:string[][])  [unwired: 6 in, 3 out]
                              n1922 = global write "全局 所有参数.vi" "CODCr"(w2349) -> ()
                              n1923 = global write "全局 所有参数.vi" "CODMn"(w2347) -> ()
                              n1924 = global write "全局 所有参数.vi" "总氮"(w2347) -> ()
                              n1925 = global write "全局 所有参数.vi" "总磷"(w2347) -> ()
                              n1926 = global write "全局 所有参数.vi" "氨氮"(w2347) -> ()
                            }
                            frame "氨氮" {
                              w2351 = string[][] [] ("氨氮")
                              n1927 = call "数据表比对.vi"("仪器日志参数"="氨氮" ("元素"), "table输入"=w2352) -> ("待发送数据"=w2353:string[][])  [unwired: 6 in, 3 out]
                              n1928 = global write "全局 所有参数.vi" "氨氮"(w2353) -> ()
                              n1929 = global write "全局 所有参数.vi" "CODMn"(w2351) -> ()
                              n1930 = global write "全局 所有参数.vi" "总氮"(w2351) -> ()
                              n1931 = global write "全局 所有参数.vi" "CODCr"(w2351) -> ()
                              n1932 = global write "全局 所有参数.vi" "总磷"(w2351) -> ()
                            }
                            frame "总磷" {
                              w2356 = string[][] [] ("氨氮")
                              n1933 = call "数据表比对.vi"("仪器日志参数"="总磷" ("元素"), "table输入"=w2357) -> ("待发送数据"=w2358:string[][])  [unwired: 6 in, 3 out]
                              n1934 = global write "全局 所有参数.vi" "总磷"(w2358) -> ()
                              n1935 = global write "全局 所有参数.vi" "CODMn"(w2356) -> ()
                              n1936 = global write "全局 所有参数.vi" "总氮"(w2356) -> ()
                              n1937 = global write "全局 所有参数.vi" "CODCr"(w2356) -> ()
                              n1938 = global write "全局 所有参数.vi" "氨氮"(w2356) -> ()
                            }
                            frame "总氮" {
                              w2361 = string[][] [] ("氨氮")
                              n1939 = call "数据表比对.vi"("仪器日志参数"="总氮" ("元素"), "table输入"=w2362) -> ("待发送数据"=w2363:string[][])  [unwired: 6 in, 3 out]
                              n1940 = global write "全局 所有参数.vi" "总氮"(w2363) -> ()
                              n1941 = global write "全局 所有参数.vi" "CODMn"(w2361) -> ()
                              n1942 = global write "全局 所有参数.vi" "氨氮"(w2361) -> ()
                              n1943 = global write "全局 所有参数.vi" "CODCr"(w2361) -> ()
                              n1944 = global write "全局 所有参数.vi" "总磷"(w2361) -> ()
                            }
                            frame "数采仪" {
                              n1945 = call "数据表比对.vi"("仪器日志参数"="系统" ("元素"), "table输入"=w2366) -> ("待发送数据"=w2367:string[][])  [unwired: 6 in, 3 out]
                              n1946 = global write "全局 所有参数.vi" "DO"(w2367) -> ()
                            }
                          }
                          n1947 = Get Queue Status(queue=w2338) -> (# elements in queue=w2337:i32)  [unwired: 2 in, 7 out]
                          n1948 = Wait (ms)(milliseconds to wait=u32 300 ("等待时间（毫秒）")) -> ()  [unwired: 1 out]
                          n1949 = Equal To 0?(x=w2337) -> (x = 0?=w2336:bool)
                        }
                      }
                    }
                  }
                  frame #2 {
                    n1950 = local read "数据"() -> (w2378:string)
                    n1951 = Search/Split String(string=w2378, search string/char (-)="InfoId=" ("搜索字符串/字符(-)")) -> (match + rest of string=w2376:string)  [unwired: 1 in, 2 out]
                    n1952 = String Subset(string=w2376, offset (0)=7 ("偏移量(0)"), length (rest)=6 ("长度（剩余）")) -> (substring=w2372:string)
                    n1953 = case shown="\"i13001\", \"i13002\", \"i13003\", \"i13004\", \"i13005\", \"i13006\", \"i13007\", \"i13008\", \"i13009\", \"i13010\", \"i13011\", \"i13012\", \"i13013\"" w2372 {
                      selector: w2372 -> [_ w2383 _]
                      tunnel: ["操作日志" ("名称（未命名）") "提取仪器参数" ("名称（未命名）") "报警信息" ("名称（未命名）")] -> w2371
                      tunnel: [w2379 1 ("数据数组大小") w2386] -> w2370
                      frame "i11001", "i21001" {
                        # "数据处理整合"
                        # "i11001日志"
                        n1954 = call "数据处理整合 (子VI).vi"("枚举"=enum16{"实时数据排序", "小时数据排序"}."实时数据排序") -> ("已排序的数组"=w2380:string[])  [unwired: 10 in]
                        n1955 = Array Size(array=w2380) -> (size(s)=w2379:i32)
                      }
                      frame "i13001", "i13002", "i13003", "i13004", "i13005", "i13006", "i13007", "i13008", "i13009", "i13010", "i13011", "i13012", "i13013" {
                        n1956 = global write "全局 提取仪器参数.vi" "参数编码"(w2383) -> ()
                        n1957 = call "数据处理直接插入整合 (子VI).vi"() -> ()  [unwired: 12 in]
                      }
                      frame "i12001", Default {
                        # "数据处理整合"
                        # "i12001状态"
                        n1958 = call "数据处理整合 (子VI).vi"("枚举"=enum16{"实时数据排序", "小时数据排序"}."实时数据排序") -> ("已排序的数组"=w2387:string[])  [unwired: 10 in]
                        n1959 = Array Size(array=w2387) -> (size(s)=w2386:i32)
                      }
                    }
                    n1960 = global write "全局 数据数组大小.vi" "数据数组大小"(w2370) -> ()
                    n1961 = local write "table元素"(w2371) -> ()
                  }
                }
              }
              frame "3021" {
                # "设置仪表参数"
                n1962 = local write "table元素"("反控命令" ("新元素/子数组")) -> ()
              }
              frame "3040" {
                # "提取现场系统信息（3040）"
                n1963 = flat-sequence {
                  tunnel: [T6."发送数据" ("元素")] -> w2393
                  frame #0 {
                    n1964 = local write "table元素"("提取现场系统信息" ("新元素/子数组")) -> ()
                  }
                  frame #1 {
                  }
                }
              }
              frame "3041" {
                # "提取现场经纬度及环境信息（3041）"
                n1965 = flat-sequence {
                  tunnel: [T6."发送数据" ("元素")] -> w2397
                  frame #0 {
                    n1966 = call "获取环境参数 (子VI).vi"() -> ()  [unwired: 12 in]
                    n1967 = local write "table元素"("提取经纬度环境信息" ("新元素/子数组")) -> ()
                  }
                  frame #1 {
                  }
                }
              }
              frame "3042" {
                # "发命令给中控"
                # "反控指令"
                # "0维护，1常规，2应急，3质控"
                # "反控指令\n切换运行模式"
                n1968 = local write "table元素"("反控命令" ("新元素/子数组")) -> ()
                n1969 = property on="数据" class="Str"() -> ("Value"=w2416:string)  [unwired: 2 in, 2 out]
                n1970 = Search/Split String(string=w2416, search string/char (-)="RunMode" ("搜索字符串/字符(-)")) -> (match + rest of string=w2414:string)  [unwired: 1 in, 2 out]
                n1971 = String Subset(string=w2414, offset (0)=8 ("偏移量(0)"), length (rest)=1 ("长度（剩余）")) -> (substring=w2411:string)
                n1972 = case shown="\"2\"" w2411 {
                  tunnel: [u16 0 ("新元素/子数组") u16 1 ("新元素/子数组") u16 2 ("新元素/子数组") u16 3 ("新元素/子数组")] -> w2405
                  frame "0", Default {
                  }
                  frame "1" {
                  }
                  frame "2" {
                  }
                  frame "3" {
                  }
                }
                n1973 = Insert Into Array(array=u16[] [] ("holding register values"), index=0 ("索引"), new element=w2405) -> (w2406:u16[])
                n1974 = call "Modbus Master.vi"("Unit ID"=u8 1, "读取写入选择"="写入", "holding register values"=w2406, "starting address"=u16 0) -> ()  [unwired: 6 in, 2 out]
              }
              frame "3043" {
                # "远程重启数采仪"
                n1975 = local write "table元素"("反控命令" ("新元素/子数组")) -> ()
              }
              frame "3044" {
                # "发回给平台"
                # "反控指令"
                # "3042~3086"
                # "反控指令\n单次测量"
                # "3044"
                n1976 = local write "table元素"("反控命令" ("新元素/子数组")) -> ()
                n1977 = flat-sequence {
                  frame #0 {
                    # "发命令给中控"
                    n1978 = call "Modbus Master.vi"("Unit ID"=u8 1, "读取写入选择"="写入", "holding register values"=u16[] [1], "starting address"=u16 2) -> ()  [unwired: 6 in, 2 out]
                  }
                  frame #1 {
                    n1979 = Wait (ms)(milliseconds to wait=u32 500 ("等待时间（毫秒）")) -> ()  [unwired: 1 out]
                  }
                  frame #2 {
                    n1980 = call "Modbus Master.vi"("Unit ID"=u8 1, "读取写入选择"="写入", "holding register values"=u16[] [0], "starting address"=u16 2) -> ()  [unwired: 6 in, 2 out]
                  }
                }
              }
              frame "3045", "3046" {
                # "发回给平台"
                # "反控指令"
                # "3042~3086"
                # "反控指令\n急停"
                # "3045"
                n1981 = flat-sequence {
                  frame #0 {
                    # "发命令给中控"
                    n1982 = call "Modbus Master.vi"("Unit ID"=u8 1, "读取写入选择"="写入", "holding register values"=u16[] [1], "starting address"=u16 3) -> ()  [unwired: 6 in, 2 out]
                  }
                  frame #1 {
                    n1983 = Wait (ms)(milliseconds to wait=u32 500 ("等待时间（毫秒）")) -> ()  [unwired: 1 out]
                  }
                  frame #2 {
                    n1984 = call "Modbus Master.vi"("Unit ID"=u8 1, "读取写入选择"="写入", "holding register values"=u16[] [0], "starting address"=u16 3) -> ()  [unwired: 6 in, 2 out]
                  }
                }
                n1985 = local write "table元素"("反控命令" ("新元素/子数组")) -> ()
              }
              frame "3056" {
                # "发命令给中控"
                # "设置测量时间间隔"
                # "发回给平台"
                n1986 = property on="数据" class="Str"() -> ("Value"=w2454:string)  [unwired: 2 in, 2 out]
                n1987 = local write "table元素"("反控命令" ("新元素/子数组")) -> ()
                n1988 = Search/Split String(string=w2454, search string/char (-)="RunInterval" ("搜索字符串/字符(-)")) -> (match + rest of string=w2455:string)  [unwired: 1 in, 2 out]
                n1989 = Decimal String To Number(string=w2455, offset=12 ("偏移量(0)")) -> (number=w2450:i32)  [unwired: 1 in, 1 out]
                n1990 = Insert Into Array(array=u16[] [] ("holding register values"), index=0 ("索引"), new element=w2450) -> (w2449:u16[])
                n1991 = call "Modbus Master.vi"("Unit ID"=u8 1, "读取写入选择"="写入", "holding register values"=w2449, "starting address"=u16 14) -> ()  [unwired: 6 in, 2 out]
              }
              frame "3080", "3081", "3082", "3083", "3084", "3085", "3086" {
                # "30 启动标液核查  1CODmn  2 氨氮  3总磷  4总氮  5CODCr\n31 加标回收\n32 平行样测试\n33 零点核查\n34 跨度核查\n35 校零\n36 校标"
                # "发回给平台"
                n1992 = flat-sequence {
                  tunnel: w2464 -> [w2470]
                  tunnel: [w2468] -> w2463
                  tunnel: w2463 -> [w2496]
                  tunnel: [w2496] -> w2462
                  tunnel: w2462 -> [w2499]
                  frame #0 {
                    # "1CODmn  2 氨氮  3总磷  4总氮  5CODCr"
                    # "启动单台仪器标液核查"
                    # "发命令给中控"
                    n1993 = property on="数据" class="Str"() -> ("Value"=w2480:string)  [unwired: 2 in, 2 out]
                    n1994 = Search/Split String(string=w2480, search string/char (-)="PolId" ("搜索字符串/字符(-)")) -> (match + rest of string=w2475:string)  [unwired: 1 in, 2 out]
                    n1995 = String Subset(string=w2475, offset (0)=6 ("偏移量(0)"), length (rest)=6 ("长度（剩余）")) -> (substring=w2472:string)
                    n1996 = case shown="\"w01019\"" w2472 {
                      tunnel: [0 ("长度（剩余）") 1 ("长度（剩余）") 2 ("长度（剩余）") 3 ("长度（剩余）") 4 ("长度（剩余）") 5 ("长度（剩余）")] -> w2471
                      frame "", Default {
                      }
                      frame "w01019" {
                      }
                      frame "w21003" {
                      }
                      frame "w21011" {
                      }
                      frame "w21001" {
                      }
                      frame "w01018" {
                      }
                    }
                    n1997 = Insert Into Array(array=u16[] [] ("holding register values"), index=0 ("索引"), new element=w2471) -> (w2476:u16[])
                    n1998 = case shown="\"3086\"" w2470 {
                      tunnel: [u16 99 ("starting address") u16 30 ("starting address") u16 31 ("starting address") u16 32 ("starting address") u16 33 ("starting address") u16 34 ("starting address") u16 35 ("starting address") u16 36 ("starting address")] -> w2468
                      frame "", Default {
                      }
                      frame "3080" {
                      }
                      frame "3081" {
                      }
                      frame "3082" {
                      }
                      frame "3083" {
                      }
                      frame "3084" {
                      }
                      frame "3085" {
                      }
                      frame "3086" {
                      }
                    }
                    n1999 = call "Modbus Master.vi"("Unit ID"=u8 1, "读取写入选择"="写入", "holding register values"=w2476, "starting address"=w2468) -> ()  [unwired: 6 in, 2 out]
                  }
                  frame #1 {
                    n2000 = Wait (ms)(milliseconds to wait=u32 500 ("等待时间（毫秒）")) -> ()  [unwired: 1 out]
                  }
                  frame #2 {
                    n2001 = call "Modbus Master.vi"("Unit ID"=u8 1, "读取写入选择"="写入", "holding register values"=u16[] [0], "starting address"=w2499) -> ()  [unwired: 6 in, 2 out]
                  }
                }
                n2002 = local write "table元素"("反控命令" ("新元素/子数组")) -> ()
              }
            }
            n2003 = Enqueue Element(queue=w2031, element=w2030, timeout in ms (-1)=1000 ("超时毫秒(-1)")) -> ()  [unwired: 1 in, 3 out]
          }
          frame "发送数据" {
            # "table输入，选择命令编码、发送哪些数据"
            n2004 = local read "table元素"() -> (w2506:string)
            n2005 = case shown="\"报警信息\", \"操作日志\", \"核查数据\", \"空白测试\", \"跨度核查\", \"零点核查\", \"实时数据\", \"提取集成干预\", \"提取加标回收\", \"提取平行样\", \"提取实时数据\", \"提取小时数据\", \"提取仪器参数\", \"仪器参数\"" w2506 {
              tunnel: w2505 -> [w2517 w2521 w2523 w2530]
              tunnel: [w2515 w2520 w2524 w2528] -> w2503
              tunnel: [w2516 w2519 w2525 w2529] -> w2504
              frame "", Default {
                n2006 = Increment(x=w2517) -> (x+1=w2516:i32)
                n2007 = global write "全局1.vi" "枚举"(w2517) -> ()
                n2008 = Greater Or Equal?(x=w2516, y=3) -> (x >= y?=w2515:bool)
              }
              frame "反控命令" {
                n2009 = Increment(x=w2521) -> (x+1=w2519:i32)
                n2010 = global write "全局 反控命令枚举.vi" "反控命令枚举"(w2521) -> ()
                n2011 = Greater Or Equal?(x=w2519, y=2) -> (x >= y?=w2520:bool)
              }
              frame "超标留样返回", "提取监测仪表时间", "提取经纬度环境信息", "提取现场系统信息" {
                n2012 = Increment(x=w2523) -> (x+1=w2525:i32)
                n2013 = global write "全局1.vi" "枚举"(w2523) -> ()
                n2014 = Greater Or Equal?(x=w2525, y=3) -> (x >= y?=w2524:bool)
              }
              frame "报警信息", "操作日志", "核查数据", "空白测试", "跨度核查", "零点核查", "实时数据", "提取集成干预", "提取加标回收", "提取平行样", "提取实时数据", "提取小时数据", "提取仪器参数", "仪器参数" {
                n2015 = global read "全局 小时数据发送次数.vi" "小时数据发送次数"() -> (w2532:i32)
                n2016 = global read "全局 数据数组大小.vi" "数据数组大小"() -> (w2527:i32)
                n2017 = Greater Or Equal?(x=w2532, y=w2527) -> (x >= y?=w2533:bool)
                n2018 = case shown="真" w2533 {
                  tunnel: w2530 -> [w2538 w2545]
                  tunnel: [w2538 w2539] -> w2534
                  frame False {
                  }
                  frame True {
                    n2019 = global read "全局 小时数据发送次数.vi" "小时数据发送次数"() -> (w2544:i32)
                    n2020 = global read "全局 数据数组大小.vi" "数据数组大小"() -> (w2541:i32)
                    n2021 = Equal To 0?(x=w2541) -> (x = 0?=w2542:bool)
                    n2022 = Equal To 0?(x=w2544) -> (x = 0?=w2543:bool)
                    n2023 = And(x=w2543, y=w2542) -> (x .and. y?=w2540:bool)
                    n2024 = case shown="真" w2540 {
                      tunnel: w2545 -> [w2547 _]
                      tunnel: [w2546 0 ("索引")] -> w2539
                      frame False {
                        n2025 = Increment(x=w2547) -> (x+1=w2546:i32)
                      }
                      frame True {
                      }
                    }
                  }
                }
                n2026 = Equal To 0?(x=w2534) -> (x = 0?=w2535:bool)
                n2027 = global write "全局1.vi" "枚举"(w2534) -> ()
                n2028 = case shown="真" w2535 {
                  tunnel: w2534 -> [w2536 _]
                  tunnel: [w2536 1] -> w2529
                  frame False {
                  }
                  frame True {
                  }
                }
                n2029 = Greater Or Equal?(x=w2529, y=2) -> (x >= y?=w2528:bool)
              }
            }
            n2030 = case shown="假" w2503 {
              tunnel: w2504 -> [w2549 _]
              tunnel: [w2549 1 ("索引")] -> w2508
              frame False {
              }
              frame True {
              }
            }
            n2031 = flat-sequence {
              tunnel: "table元素" -> [w2560]
              tunnel: w2512 -> [w2559]
              tunnel: [w2555] -> w2511
              tunnel: [w2564] -> w2509
              tunnel: w2511 -> [w2564]
              tunnel: w2510 -> [w2563]
              tunnel: w2503 -> [w2562]
              frame #0 {
                # "数据记录"
                # "数据编码"
                n2032 = local read "QN"() -> (w2558:string)
                n2033 = local read "MN"() -> (w2552:string)
                n2034 = local read "PW"() -> (w2551:string)
                n2035 = call "数据编码.vi"("table输入"=w2560, "错误常量 2"=w2559, "QN"=w2558, "MN"=w2552, "PW"=w2551) -> ("错误常量"=w2557:errorcluster, "通讯包字符串"=w2556:string)  [unwired: 9 in]
                n2036 = local read "数据发送通道"() -> (w2554:enum16{"TCP", "VISA"})
                n2037 = call "数据记录.vi"("写入字段"=w2556) -> ("连接的字符串"=→"发送报文显示":string)  [unwired: 10 in]
                n2038 = call "VISATCP组合选择发送.vi"("数据发送通道"=w2554, "命令"="write", "error in (no error)"=w2557, "写入缓冲区"=w2556) -> ("错误输出"=w2555:errorcluster)  [unwired: 8 in, 3 out]
              }
              frame #1 {
                n2039 = case shown="真" w2562 {
                  tunnel: w2563 -> [w2565 w2577]
                  frame False {
                    n2040 = Enqueue Element(queue=w2565, element=T6."发送数据" ("元素")) -> ()  [unwired: 2 in, 3 out]
                  }
                  frame True {
                    n2041 = local read "TCP服务端掉线计数"() -> (w2572:i32)
                    n2042 = Obtain Queue(name (unnamed)="重发掉线数据" ("名称（未命名）"), element data type=T16."水样测试") -> (queue out=w2570:refnum<queue>, error out=w2571:errorcluster)  [unwired: 3 in, 1 out]
                    n2043 = Get Queue Status(queue=w2570, error in (no error)=w2571) -> (# elements in queue=w2574:i32)  [unwired: 1 in, 7 out]
                    n2044 = Not Equal To 0?(x=w2574) -> (x != 0?=w2575:bool)
                    n2045 = Greater Or Equal?(x=w2572, y=1) -> (x >= y?=w2576:bool)
                    n2046 = And(x=w2575, y=w2576) -> (x .and. y?=w2568:bool)
                    n2047 = case shown="真" w2568 {
                      tunnel: [T6."读取数据" ("元素") T6."表格比对" ("元素")] -> w2578
                      frame False {
                      }
                      frame True {
                      }
                    }
                    n2048 = Enqueue Element(queue=w2577, element=w2578) -> ()  [unwired: 2 in, 3 out]
                  }
                }
              }
            }
            "查询数据发送" <- TRUE
          }
          frame "数据处理" {
            n2049 = local write "空闲时间"(0.0 ("空闲时间")) -> ()
            n2050 = local read "心跳包"() -> (w2589:bool)
            n2051 = Equal?(x=w2587, y="实时数据") -> (x = y?=w2585:bool)
            n2052 = case shown="假" w2589 {
              tunnel: w2593 -> [w2596 _]
              tunnel: w2587 -> [w2595 _]
              frame False {
                n2053 = call "插入单条数据.vi"("table输入"=w2595, "插入数据"=w2596) -> ()  [unwired: 8 in, 2 out]
              }
              frame True {
              }
            }
            n2054 = Select(t=0, s=w2585, f=w2583) -> (s? t:f=w2584:i32)
            n2055 = Enqueue Element(queue=w2592, element=T6."表格比对" ("元素"), timeout in ms (-1)=1000 ("超时毫秒(-1)")) -> ()  [unwired: 1 in, 3 out]
          }
        }
      }
      frame Error {
        n2056 = Unbundle By Name(w2600) -> ("code"=w2599:i32)
        n2057 = case shown="63" w2599 {
          tunnel: w2600 -> [w2605 w2615 w2648 w2676]
          tunnel: [w2611 w2631 w2664 w2676] -> w2604
          tunnel: w2598 -> [w2612 w2626 w2659 w2673]
          frame 0, Default {
            n2058 = Flush Queue(queue=w2612) -> (queue out=w2610:refnum<queue>)  [unwired: 1 in, 2 out]
            n2059 = Enqueue Element(queue=w2610, element=T6."初始化" ("元素"), timeout in ms (-1)=1000 ("超时毫秒(-1)")) -> ()  [unwired: 1 in, 3 out]
            n2060 = local read "数据发送通道"() -> (w2607:enum16{"TCP", "VISA"})
            n2061 = call "VISATCP组合选择发送.vi"("数据发送通道"=w2607, "命令"="close", "error in (no error)"=w2605) -> ("错误输出"=w2606:errorcluster)  [unwired: 9 in, 3 out]
            n2062 = call <vilib>:"Clear Errors.vi"("error in (no error)"=w2606) -> ("error out"=w2611:errorcluster)  [unwired: 5 in, 1 out]
            n2063 = global write "全局 数据发送重叠.vi" "掉线指示灯"(TRUE ("掉线指示灯")) -> ()
          }
          frame 63 {
            # "TCP服务器端口掉线"
            n2064 = Flush Queue(queue=w2626) -> (queue out=w2627:refnum<queue>)  [unwired: 1 in, 2 out]
            n2065 = local read "查询数据发送"() -> (w2623:bool)
            n2066 = property on="TCP服务端掉线计数" class="DigNum (严格)"() -> ("Value"=w2622:i32)  [unwired: 2 in, 2 out]
            n2067 = call <vilib>:"Boolean Crossing PtByPt.vi"("direction"=enum16{"either", "false-true", "true-false"}."false-true", "input"=w2623) -> ("crossing"=w2624:bool)  [unwired: 1 in]
            n2068 = Less Or Equal?(x=w2622, y=1) -> (x <= y?=w2620:bool)
            n2069 = Enqueue Element(queue=w2627, element=T6."初始化" ("元素"), timeout in ms (-1)=1000 ("超时毫秒(-1)")) -> ()  [unwired: 1 in, 3 out]
            n2070 = case shown="真" w2624 {
              frame False {
              }
              frame True {
                n2071 = disable-structure shown="禁用" {
                  frame Disabled {
                    # "判定数据为空时不写入临时表格"
                    n2072 = call "每个元素都写入临时表格 (子VI).vi"("组合框"="小时数据存储") -> ()  [unwired: 10 in, 1 out]
                  }
                  frame Enabled {
                  }
                }
              }
            }
            n2073 = case shown="真" w2620 {
              frame False {
                n2074 = global write "全局 数据发送重叠.vi" "TCP掉线时间节点"("TCP掉线时间节点") -> ()
                n2075 = local write "TCP掉线时间节点"("TCP掉线时间节点") -> ()
              }
              frame True {
                n2076 = Get Date/Time In Seconds() -> (seconds since 1Jan1904=w2644:timestamp)
                n2077 = Format Date/Time String(time format string (%c)="%Y%m%d%H%M%S%3u" ("时间格式字符串(%c)"), seconds (now)=w2644) -> (date/time string=w2646:string)  [unwired: 1 in]
                n2078 = call "格式时间字符串.vi"("字符串"=w2646) -> ("连接的字符串"=w2634:string)  [unwired: 10 in]
                n2079 = local write "TCP掉线时间节点"(w2634) -> ()
                n2080 = call <vilib>:"Application Directory.vi"() -> ("Application Directory"=w2642:path)
                n2081 = Build Path(base path=w2642, name or relative path="data\\Set.ini" ("名称或相对路径")) -> (appended path=w2643:path)
                n2082 = call <vilib>:"Open Config Data.vi"("configuration file path"=w2643) -> ("error out"=w2639:errorcluster, "refnum"=w2640:T8)  [unwired: 8 in, 1 out]
                n2083 = call-poly <vilib>:"Write Key.vi"("section"="掉线时间存储", "error in (no error)"=w2639, "value"=w2634, "key"="掉线时间", "refnum"=w2640) -> ("error out"=w2637:errorcluster, "refnum out"=w2638:T8)  [unwired: 4 in, 1 out]
                n2084 = call <vilib>:"Close Config Data.vi"("error in (no error)"=w2637, "refnum"=w2638) -> ()  [unwired: 8 in, 2 out]
              }
            }
            n2085 = local read "数据发送通道"() -> (w2617:enum16{"TCP", "VISA"})
            n2086 = call "VISATCP组合选择发送.vi"("数据发送通道"=w2617, "命令"="close", "error in (no error)"=w2615) -> ("错误输出"=w2616:errorcluster)  [unwired: 9 in, 3 out]
            n2087 = call <vilib>:"Clear Errors.vi"("error in (no error)"=w2616) -> ("error out"=w2631:errorcluster)  [unwired: 5 in, 1 out]
            n2088 = global write "全局 数据发送重叠.vi" "掉线指示灯"(TRUE ("掉线指示灯")) -> ()
            n2089 = property on="TCP服务端掉线计数" class="DigNum (严格)"() -> ("Value"=w2630:i32)  [unwired: 2 in, 2 out]
            n2090 = Increment(x=w2630) -> (x+1=w2628:i32)
            n2091 = property on="TCP服务端掉线计数" class="DigNum (严格)"("Value"=w2628) -> ()  [unwired: 2 in, 2 out]
          }
          frame 54 {
            # "TCP服务器端口掉线"
            n2092 = local read "查询数据发送"() -> (w2656:bool)
            n2093 = Flush Queue(queue=w2659) -> (queue out=w2660:refnum<queue>)  [unwired: 1 in, 2 out]
            n2094 = property on="TCP服务端掉线计数" class="DigNum (严格)"() -> ("Value"=w2655:i32)  [unwired: 2 in, 2 out]
            n2095 = call <vilib>:"Boolean Crossing PtByPt.vi"("direction"=enum16{"either", "false-true", "true-false"}."false-true", "input"=w2656) -> ("crossing"=w2657:bool)  [unwired: 1 in]
            n2096 = Less Or Equal?(x=w2655, y=1) -> (x <= y?=w2653:bool)
            n2097 = Enqueue Element(queue=w2660, element=T6."初始化" ("元素"), timeout in ms (-1)=1000 ("超时毫秒(-1)")) -> ()  [unwired: 1 in, 3 out]
            n2098 = case shown="真" w2657 {
              frame False {
              }
              frame True {
                n2099 = disable-structure shown="禁用" {
                  frame Disabled {
                    # "判定数据为空时不写入临时表格"
                    n2100 = call "每个元素都写入临时表格 (子VI).vi"("组合框"="小时数据存储") -> ()  [unwired: 10 in, 1 out]
                  }
                  frame Enabled {
                  }
                }
              }
            }
            n2101 = case shown="真" w2653 {
              frame False {
                n2102 = local read "TCP掉线时间节点"() -> (w2666:string)
                n2103 = global write "全局 数据发送重叠.vi" "TCP掉线时间节点"(w2666) -> ()
                n2104 = local write "TCP掉线时间节点"(w2666) -> ()
              }
              frame True {
                n2105 = Get Date/Time In Seconds() -> (seconds since 1Jan1904=w2668:timestamp)
                n2106 = Format Date/Time String(time format string (%c)="%Y%m%d%H%M%S%3u" ("时间格式字符串(%c)"), seconds (now)=w2668) -> (date/time string=w2670:string)  [unwired: 1 in]
                n2107 = call "格式时间字符串.vi"("字符串"=w2670) -> ("连接的字符串"=w2667:string)  [unwired: 10 in]
                n2108 = local write "TCP掉线时间节点"(w2667) -> ()
              }
            }
            n2109 = local read "数据发送通道"() -> (w2650:enum16{"TCP", "VISA"})
            n2110 = property on="TCP服务端掉线计数" class="DigNum (严格)"() -> ("Value"=w2663:i32)  [unwired: 2 in, 2 out]
            n2111 = call "VISATCP组合选择发送.vi"("数据发送通道"=w2650, "命令"="close", "error in (no error)"=w2648) -> ("错误输出"=w2649:errorcluster)  [unwired: 9 in, 3 out]
            n2112 = Increment(x=w2663) -> (x+1=w2661:i32)
            n2113 = property on="TCP服务端掉线计数" class="DigNum (严格)"("Value"=w2661) -> ()  [unwired: 2 in, 2 out]
            n2114 = call <vilib>:"Clear Errors.vi"("error in (no error)"=w2649) -> ("error out"=w2664:errorcluster)  [unwired: 5 in, 1 out]
            n2115 = global write "全局 数据发送重叠.vi" "掉线指示灯"(TRUE ("掉线指示灯")) -> ()
          }
          frame 56 {
            n2116 = Flush Queue(queue=w2673) -> (queue out=w2674:refnum<queue>)  [unwired: 1 in, 2 out]
            n2117 = Enqueue Element(queue=w2674, element=T6."读取数据" ("元素"), timeout in ms (-1)=1000 ("超时毫秒(-1)")) -> ()  [unwired: 1 in, 3 out]
          }
        }
        n2118 = call <vilib>:"Clear Errors.vi"("error in (no error)"=w2604) -> ("error out"=w2603:errorcluster)  [unwired: 5 in, 1 out]
      }
    }
  }
  n2119 = register-events(error in=w17, w18) -> (reference out=w6:refnum<event-registration>, error out=w5:errorcluster)  [unwired: 1 in]
  n2120 = while {
    shift-right: [w2680] -> w9
    shift-left: w5 -> [w2679]
    shift-right: [w2681] -> w12
    shift-left: w7 -> [w2682]
    shift-right: [w2678] -> w11
    shift-left: w6 -> [w2683]
    tunnel: [w2677] -> _
    stop <- w2677 stop-if-true
    n2121 = case shown="无错误" w2679 {
      selector: w2679 -> [w2685 w2719]
      tunnel: w2683 -> [w2690 w2714]
      tunnel: w2682 -> [w2689 w2715]
      tunnel: [w2688 w2715] -> w2681
      tunnel: [w2687 w2717] -> w2680
      tunnel: [w2686 FALSE ("Discard?")] -> w2677
      tunnel: [w2684 w2714] -> w2678
      frame No Error {
        n2122 = event shown="[0] <Public:SelectedItemEvent>: 用户事件" {
          selector: w2690 -> [_ _ _]
          dyn-events: [_ _ _] -> w2684
          timeout: _ -> [_ _ _]
          tunnel: w2685 -> [w2693 w2703 w2712]
          tunnel: [w2693 w2703 w2711] -> w2687
          tunnel: [w2692 TRUE FALSE ("Discard?")] -> w2686
          tunnel: w2689 -> [w2691 w2701 w2713]
          tunnel: [w2691 w2701 w2710] -> w2688
          event User Event {
            # "5."
            n2123 = event-data() -> ("ItemTag"=w2694:string)  [unwired: 1 in]
            n2124 = case shown="\"EXIT线程一\"" w2694 {
              tunnel: [FALSE TRUE] -> w2692
              frame Default {
                n2125 = Current VI's Path() -> (path=w2695:path)
                n2126 = Open VI Reference(vi path=w2695) -> (vi reference=w2696:refnum<vi>)  [unwired: 5 in, 1 out]
                n2127 = invoke class="VI" method="FP.Open"(reference=w2696, "Activate"=TRUE ("激活？")) -> ()  [unwired: 3 in, 5 out]
              }
              frame "EXIT线程一" {
              }
            }
          }
          event "停止 2": Value Change {
            # "5."
            n2128 = event-data() -> ()  [unwired: 1 in, 2 out]
            n2129 = Stop(stop? (T)=TRUE ("可见")) -> ()
          }
          event Panel Close? {
            # "4."
            n2130 = event-data() -> ("VIRef"=w2706:refnum<vi>)  [unwired: 1 in, 3 out]
            n2131 = invoke class="VI" method="FP.Open"(reference=w2706, "State"=T15."Hidden" ("状态")) -> ()  [unwired: 3 in, 5 out]
            n2132 = call <vilib>:"ShowBalloonTip.vi"("Balloon Icon"=BalloonIcon."Information", "error in"=w2712, "Text"="欢迎使用平台发送系统", "NotifyIcon in"=w2713) -> ("error out"=w2711:errorcluster, "NotifyIcon out"=w2710:refnum<class "NotifyIcon.lvclass">)  [unwired: 6 in]
            n2133 = event-data("Discard?"=TRUE ("放弃？")) -> ()  [unwired: 1 in, 1 out]
          }
        }
      }
      frame Error {
        n2134 = call <vilib>:"Simple Error Handler.vi"("error in (no error)"=w2719) -> ("error out"=w2718:errorcluster)  [unwired: 4 in, 4 out]
        n2135 = call <vilib>:"Clear Errors.vi"("error in (no error)"=w2718) -> ("error out"=w2717:errorcluster)  [unwired: 5 in, 1 out]
      }
    }
  }
  n2136 = Unregister For Events(event registration refnum=w11, error in=w9) -> (error out=w8:errorcluster)
  n2137 = property class="App"() -> ("App.Kind"=w13:T14)  [unwired: 2 in, 2 out]
  n2138 = call <vilib>:"Destructor.vi"("error in"=w8, "NotifyIcon"=w12) -> ("error out"=w14:errorcluster)  [unwired: 9 in]
  n2139 = case shown="\"Development System\"" w13 {
    tunnel: w14 -> [_ _ _ _ _ _ _]
    frame "invalid app kind", Default {
    }
    frame "Development System" {
      n2140 = Stop(stop? (T)=TRUE ("可见")) -> ()
    }
    frame "Run Time System" {
      n2141 = Quit LabVIEW(quit? (T)=TRUE ("退出？(T)")) -> ()
    }
    frame "Student Edition" {
    }
    frame "Embedded LabVIEW" {
    }
    frame "Evaluation" {
    }
    frame "Custom" {
    }
  }
  n2142 = call <vilib>:"Simple Error Handler.vi"("error in (no error)"=w14) -> ("error out"=→"error out":errorcluster)  [unwired: 4 in, 4 out]
